vi "MainKinetics.vi"() -> ()   [LabVIEW 2017]
uses:
  <vilib>/Utility/miscctls.llb/LVRowAndColumnTypeDef.ctl
  <vilib>/Utility/sysdir.llb/System Directory Type.ctl
  <vilib>/Utility/config.llb/Read Key (String).vi
  <vilib>/Utility/config.llb/Write Key (String).vi
  <vilib>/Utility/cursorutil.llb/Set Cursor (Icon Pict).vi
  PCAN_Driver/ControlCAN.lvlib
  <vilib>/Utility/config.llb/NI_LVConfig.lvlib
panel:
  out "CurrentOut":string
  out "VISA Current":refnum<visa-resource-name>
  out "Offset":dbl
  out "Analogtest":bool=TRUE
  out "TestinExecution":string
  out "FullSpeed2 Current":dbl
  out "FullSpeed1 Current":dbl
  out "String":string
  out "ParamVersion":string
  out "DSP Board S/N":string
  out "POWER Board S/N":string caption="DRIVER Board S/N"
  in  "EventTimeout":i32=100
  out "SpeedLimit":dbl[](array[numeric])
  out "TestArray":string[](array[string])
  out "Motor Speed RPM Serial":dbl
  out "DAQmx Device Name":tag
  out "PN":string
  out "FileName":string
  out "VenableSpeed":u16
  out "TesterVersion":string
  out "ClosePanel":bool=TRUE
  out "UUT SN Report":string
  out "Automation":bool
  out "Test Failed":bool
  out "VisualInspectionResult":bool
  out "MotorTempResult":bool
  out "VenableDirectionResult":bool
  out "VenableResult":bool
  out "ComTestResult":bool=TRUE
  out "UUT SoftwareVer":string
  out "Next SN":i32
  in  "SetSN":bool
  out "Current SN":i32
  out "FullSpeed2 Speed":dbl
  out "FullSpeed2 Current":dbl
  out "FullSpeed1 Current":dbl
  out "FullSpeed1 Speed":dbl
  out "UUT":u8
  out "CAN Status":bool
  out "Array":u64[][](array[numeric]) format="%016x"
  out "Motor Phase Current RMS":dbl
  out "Ambient Temperature":dbl
  out "Speed error":bool
  out "Commutation err":bool
  out "Under voltage/Over voltage":bool
  out "Derated drive temp":bool
  out "Motor Over temperature":bool
  out "Motor Sensor temp Fauilre":bool
  out "Drive Over temperature":bool
  out "Drive Sensor temp Failure":bool
  out "Ambient Over temp":bool
  out "Ambient Sensor temp":bool
  out "DC Voltage":dbl
  out "DC Current":dbl
  out "Power transistor Heat sink Temp.":dbl
  out "Motor Stator Temp.":dbl
  out "Motor Speed RPM":dbl
  out "ECS State":u16
  out "UUT":string="EBAY"
  in  "Logger Path":path
  in  "Report":bool
  in  "Start":bool
  in  "ATR":string[][](table)=[["Test Communication", "-", "-", "-", "-", ""], ["Set S/N", "-", "-", "-", "-", ""], ["Set Board Number", "-", "-", "-", "-", ""], [" ", "", "", "", "", ""], ["Test Communication", "-", "-", "-", "-", ""], ["Get S/N", "-", "-", "-", "", ""], ["Get Board Number", "-", "-", "-", "", ""], ["Get FW", "-", "-", "-", "", ""], ["Enable Motor", "", "", "", "", ""], ["Small position command", "", "", "", "", ""], ["Measure delta", "", "", "", "", ""], ["Velocity command", "", "", "", "", ""]]
  in  "Settings":bool
  in  "Refresh Button":bool
  out "Serial Status":bool
  in  "VISA Kinetics":refnum<visa-resource-name>="COM6"
  in  "Serial Com":bool
  in  "Help Button":bool
  out "Pannel User Message":string
  in  "Stop Button":bool
  # "Kinetics"
  # "REDLER TECHNOLOGIES LTD"
  # "ver 1.2p"
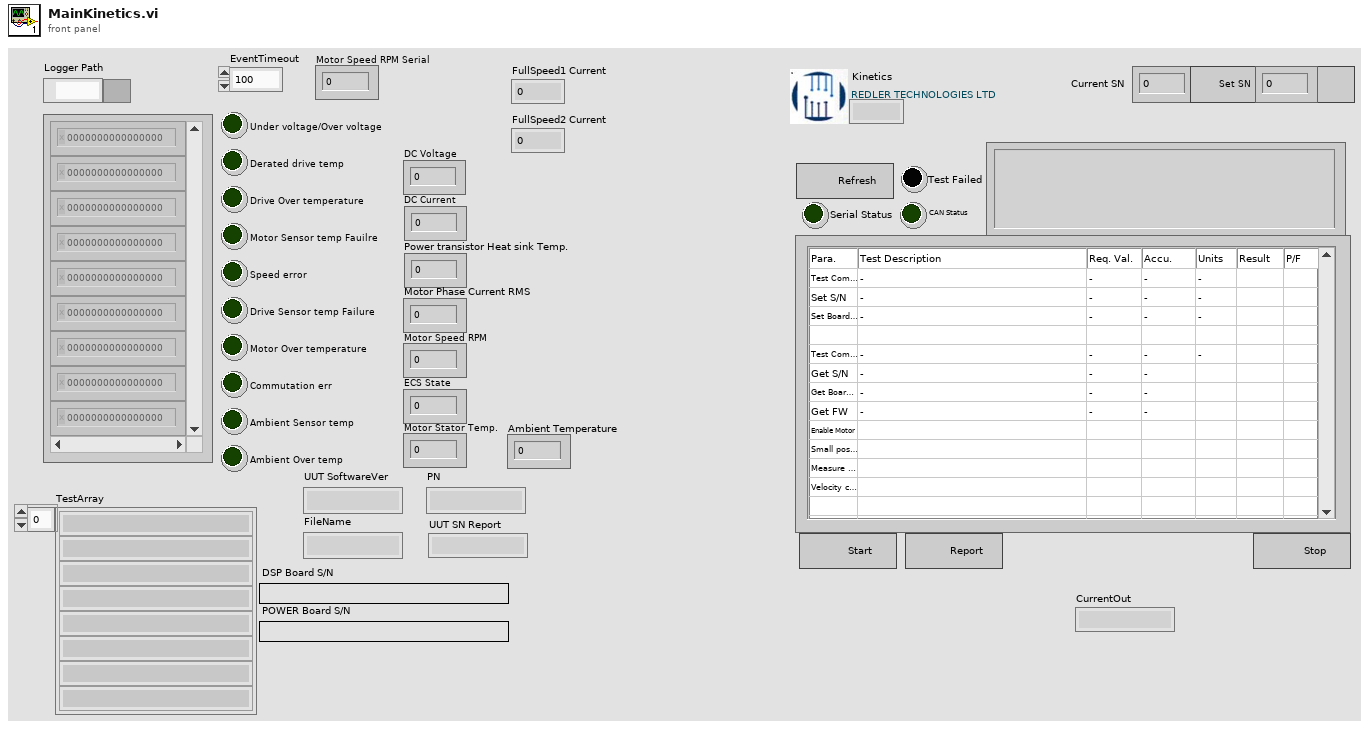
[diagram p1: front panel]
types:
  T1 = cluster{"VISA":refnum<visa-resource-name>, "TestArray":string[]}
  T2 = cluster{"ID":u32, "MSGTYPE":u8, "LEN":u8, "aDATA":u8[]}[]
  T3 = enum16{"Erase ATR Table", "Stop", "MainProgram", "Initialize"}
  T4 = typedef "NI_LVConfig.lvlib/Config Data RefNum.ctl" = refnum<k1>
  T5 = enum16{"Init", "0 ohm", "6 ohm", "13.2 ohm", "15 ohm", "25.9 ohm", "33 ohm", "Down", "Up", "Venable", "Firmware", "PowerSuply"}
  T6 = enum16{"Wait", "Exit", "VC=0", "ReadVC", "VC=1000"}
  T7 = enum16{"Stop", "Result", "FullSpeed2", "MD[1]=1", "FullSpeed1", "MD[1]=0"}
  T8 = enum16{"K15", "K16", "K17", "Venable", "Firmeware", "Fan", "Power", "120C", "110C", "100C", "90C", "80C", "70C", "60C", "50C", "40C", "30C", "25C", "20C", "10C", "0C"}
  T9 = enum8{"Term1", "Term2", "Current", "Fan", "TempCPU"}
  T10 = enum16{"Exit", "AI0/3", "AO0", "Wait", "Read", "Init"}
  T11 = enum16{"Exit", "Wait", "ReadCurrent", "ReadTemp", "Init"}
  T12 = enum16{"Init", "0 ohm", "6 ohm", "13.2 ohm", "15 ohm", "25.9 ohm", "33 ohm", "Down", "Up", "Venable", "Firmware", "PowerSuply"}[]
  T13 = enum8{"Enabled", "Disabled", "Disabled and Grayed Out"}
  T14 = typedef "LVRowAndColumnTypeDef.ctl" = cluster{"Row":i32, "Column":i32}
  T15 = enum32{"Invalid", "Standard", "Closed", "Hidden", "Minimized", "Maximized"}
  T16 = cluster{"ID":u32, "MSGTYPE":u8, "LEN":u8, "aDATA":u8[]}
  T17 = enum16{"open", "replace", "create", "open or create", "replace or create", "replace or create with confirmation"}
  T18 = typedef "ControlCAN.lvlib/DevType.ctl" = u32
  T19 = typedef "ControlCAN.lvlib/CAN Channel.ctl" = u32
  T20 = typedef "ControlCAN.lvlib/VCI_INIT_CONFIG.ctl" = cluster{"AccCode":u32, "AccMask":u32, "InitFlag":T21, "Fliter":T22, "Timing0":u8, "Timing1":u8, "Mode":T23}
  T21 = typedef "ControlCAN.lvlib/InitFlag.ctl" = u32
  T22 = typedef "ControlCAN.lvlib/Fliter.ctl" = u8
  T23 = typedef "ControlCAN.lvlib/Mode.ctl" = u8
  T24 = cluster{"DevType":T18, "DevIndex":u32, "CanIndex":T19, "VCI_INIT_CONFIG":T20}
  T25 = typedef "ControlCAN.lvlib/VCI_CAN_OBJ.ctl" = cluster{"ID":u32, "TimeStamp":u32, "TimeFlag":u8, "SendType":u8, "RemoteFlag":u8, "ExternFlag":u8, "DataLen":u8, "Data":u8[], "Reserved":u8[]}
  T26 = cluster{"Type":enum16{"接收", "发送"}, "Channel":T19, "Time":timestamp, "VCI_CAN_OBJ":T25}[]
  T27 = cluster{"Type":enum16{"接收", "发送"}, "Channel":T19, "Time":timestamp, "VCI_CAN_OBJ":T25}
  T28 = typedef "LVPoint32TypeDef.ctl" = cluster{"Horizontal":i32, "Vertical":i32}
  T29 = typedef "System Directory Type.ctl" = i32
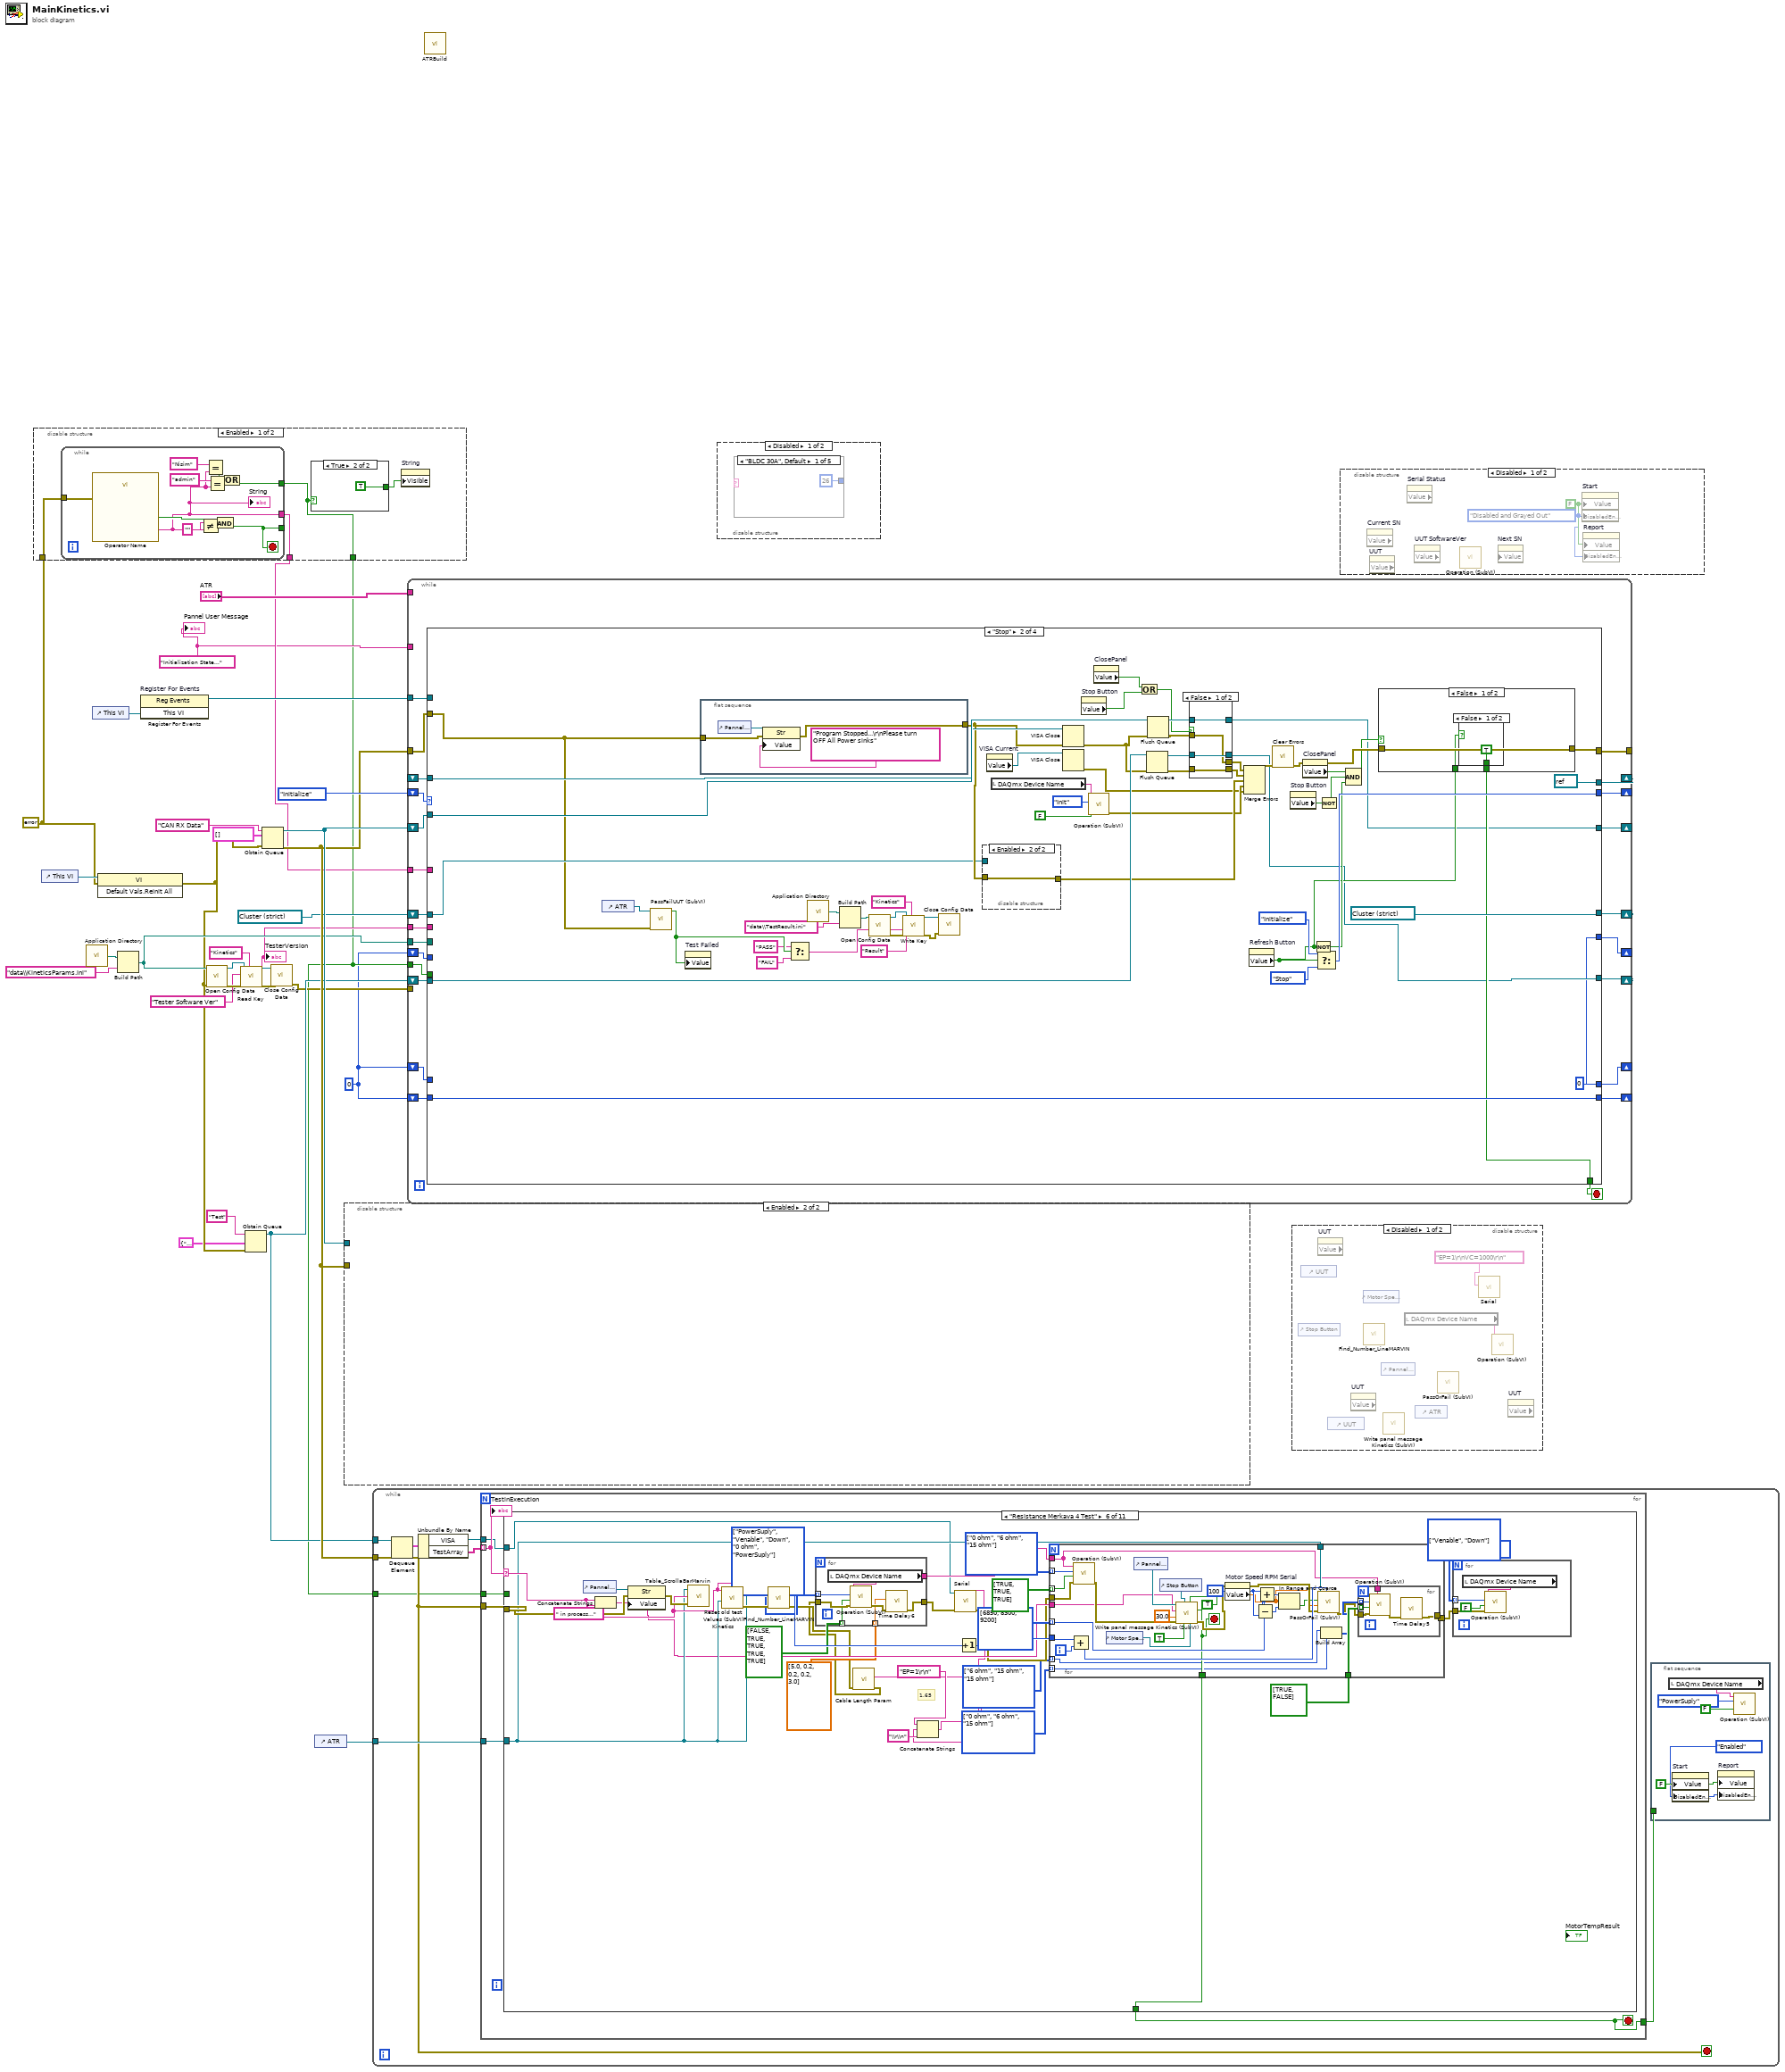
[diagram p0: block diagram]
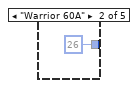
[diagram p2: hidden frame]
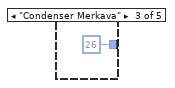
[diagram p3: hidden frame]
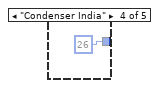
[diagram p4: hidden frame]
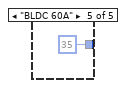
[diagram p5: hidden frame]
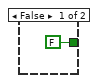
[diagram p7: hidden frame]
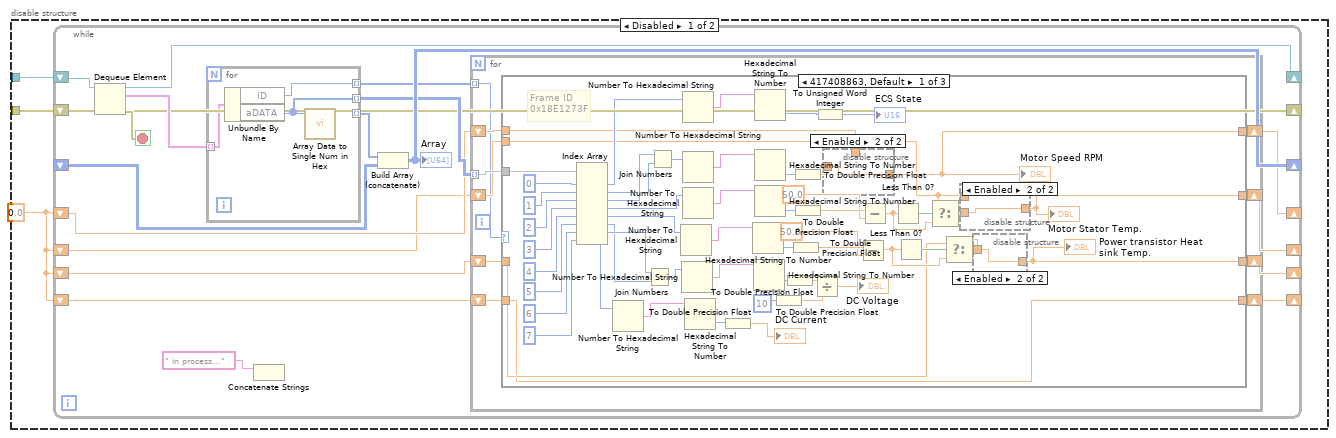
[diagram p9: hidden frame]
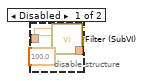
[diagram p10: hidden frame]
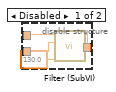
[diagram p11: hidden frame]
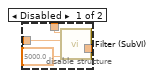
[diagram p12: hidden frame]
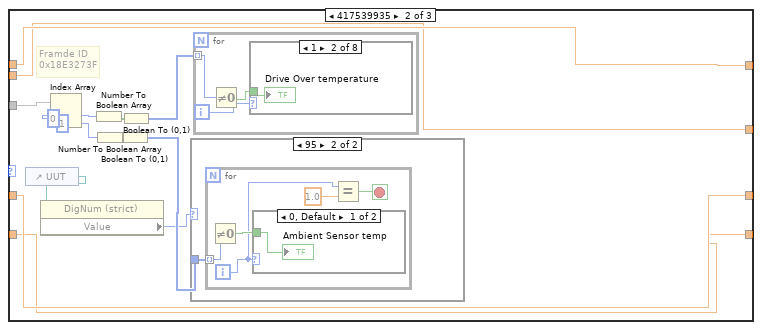
[diagram p13: hidden frame]
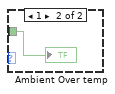
[diagram p15: hidden frame]
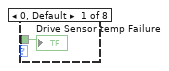
[diagram p16: hidden frame]
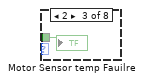
[diagram p17: hidden frame]
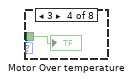
[diagram p18: hidden frame]
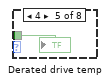
[diagram p19: hidden frame]
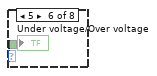
[diagram p20: hidden frame]
diagram:
  w17 = "Initialization State..."
  w2 = 0
  w5 = errorcluster {"status"=FALSE, "code"=0, "source"=""} ("error in (no error)")
  n1 = disable-structure shown="Enabled" {
    disable-tunnel: [w35 _] -> w18
    disable-tunnel: w5 -> [w33 _]
    disable-tunnel: [w32 _] -> w3
    frame Enabled {
      n2 = while {
        tunnel: [w45] -> _
        tunnel: [w38] -> w35
        tunnel: [w42] -> w32
        tunnel: w33 -> [w39]
        stop <- w45 stop-if-true
        n3 = call "Operator Name"("error in (no error)"=w39) -> ("Operator Name"=w38:string, "OK"=w46:bool)  [unwired: 16 in, 1 out]
        "String" <- w38
        n4 = Not Equal?(x=w38, y="") -> (x != y?=w47:bool)
        n5 = Equal?(x="Nisim", y=w38) -> (x = y?=w40:bool)
        n6 = Equal?(x="admin", y=w38) -> (x = y?=w43:bool)
        n7 = And(x=w46, y=w47) -> (x .and. y?=w45:bool)
        n8 = Or(x=w40, y=w43) -> (x .or. y?=w42:bool)
      }
      n9 = case shown="True" w32 {
        tunnel: [FALSE TRUE] -> w34
        frame False {
        }
        frame True {
        }
      }
      n10 = property on="String" class="Str"("Visible"=w34) -> ()  [unwired: 2 in, 2 out]
    }
    frame Disabled {
    }
  }
  n11 = control-ref of="This VI"() -> (w6:refnum<vi>)
  n12 = call <vilib>:"Application Directory.vi"() -> ("Application Directory"=w22:path)
  n13 = control-ref of="This VI"() -> (w20:refnum<vi>)
  n14 = invoke class="VI" method="Default Vals.Reinit All"(reference=w6, error in=w5) -> (error out=w4:errorcluster)  [unwired: 1 in, 2 out]
  n15 = Build Path(base path=w22, name or relative path="data\\KineticsParams.ini") -> (appended path=w9:path)
  n16 = register-events "Register For Events"(w20) -> (reference out=w19:refnum<event-registration>)  [unwired: 2 in, 1 out]
  n17 = call <vilib>:"Open Config Data.vi"("error in (no error)"=w4, "configuration file path"=w9) -> ("error out"=w15:errorcluster, "refnum"=w14:T4)  [unwired: 1 in, 7 out]
  n18 = call-poly <vilib>:"Read Key.vi"("section"="Kinetics", "error in (no error)"=w15, "key"="Tester Software Ver", "refnum"=w14) -> ("error out"=w12:errorcluster, "value"=w7:string, "refnum out"=w11:T4)  [unwired: 2 in, 3 out]
  "TesterVersion" <- w7
  n19 = Obtain Queue(name (unnamed)="Test", element data type=T1 {"VISA"="COM1", "TestArray"=[]}, error in (no error)=w4) -> (queue out=w25:refnum<queue>)  [unwired: 2 in, 2 out]
  n20 = Obtain Queue(name (unnamed)="CAN RX Data", element data type=T2 [], error in (no error)=w4) -> (queue out=w28:refnum<queue>, error out=w26:errorcluster)  [unwired: 2 in, 1 out]
  n21 = call <vilib>:"Close Config Data.vi"("error in (no error)"=w12, "refnum"=w11) -> ("error out"=w10:errorcluster)  [unwired: 8 in, 1 out]
  n22 = control-ref of="ATR"() -> (w16:refnum<vi>)
  n23 = disable-structure shown="Enabled" {
    disable-tunnel: w28 -> [w51 _]
    disable-tunnel: w26 -> [w50 _]
    frame Disabled {
      w49 = 0.0
      n24 = while {
        shift-right: [w68] -> _
        shift-left: w51 -> [w70]
        shift-right: [w66] -> _
        shift-left: _ -> [w67]
        shift-right: [w62] -> _
        shift-left: w50 -> [w62]
        shift-right: [w60] -> _
        shift-left: w49 -> [w61]
        shift-right: [w59] -> _
        shift-left: w49 -> [w58]
        shift-right: [w57] -> _
        shift-left: w49 -> [w56]
        shift-right: [w55] -> _
        shift-left: w49 -> [w54]
        stop <- w69 stop-if-true
        n25 = Dequeue Element(queue=w70, error in (no error)=w62) -> (queue out=w68:refnum<queue>, element=w63:T2, error out=w69:errorcluster)  [unwired: 1 in, 1 out]
        n26 = for {
          tunnel: [w216] -> w65 mode=indexing
          tunnel: w63 -> [w215] mode=indexing
          tunnel: [w214] -> w64 mode=indexing
          tunnel: [w213] -> w53 mode=indexing
          n27 = Unbundle By Name(w215) -> ("ID"=w213:u32, "aDATA"=w214:u8[])
          n28 = call "Array Data to Single Num in Hex.vi"("aDATA"=w214) -> ("Numeric"=w216:u64)  [unwired: 10 in]
        }
        n29 = Concatenate Strings(" in process..." ("Strin")) -> ()  [unwired: 1 in, 1 out]
        n30 = Build Array (concatenate)(w65, w67) -> (w66:u64[][])
        "Array" <- w66
        n31 = for {
          tunnel: w64 -> [w80] mode=indexing
          shift-right: [w78] -> w60
          shift-left: w61 -> [w79]
          shift-right: [w77] -> w59
          shift-left: w58 -> [w76]
          shift-right: [w75] -> w57
          shift-left: w56 -> [w74]
          shift-right: [w73] -> w55
          shift-left: w54 -> [w72]
          tunnel: w53 -> [w71] mode=indexing
          n32 = case shown="417408863, Default" w71 {
            tunnel: w80 -> [w117 w165 w203]
            tunnel: w79 -> [w91 w154 w192]
            tunnel: [w90 w154 w192] -> w78
            tunnel: [w87 w153 w191] -> w77
            tunnel: w76 -> [w86 w153 w191]
            tunnel: [w83 w152 w190] -> w75
            tunnel: w74 -> [w82 w152 w190]
            tunnel: [w81 w151 w186] -> w73
            tunnel: w72 -> [w81 w151 w185]
            frame 417408863, Default {
              # "Frame ID\n0x18E1273F"
              n33 = Index Array(array=w117, index #1=0 ("index"), index #2=1 ("index"), index #3=2 ("index"), index #4=3 ("index"), index #5=4 ("index"), index #6=5 ("index"), index #7=6 ("index"), index #8=7 ("index")) -> (element #1=w101:u8, element #2=w103:u8, element #3=w104:u8, element #4=w108:u8, element #5=w111:u8, element #6=w115:u8, element #7=w116:u8, element #8=w114:u8)
              n34 = Number To Hexadecimal String(2:w114) -> (0:w128:string)  [unwired: 1 in]
              n35 = Join Numbers(hi=w116, lo=w115) -> ((hi.lo)=w135:u16)
              n36 = Join Numbers(hi=w104, lo=w103) -> ((hi.lo)=w105:u16)
              n37 = Number To Hexadecimal String(2:w111) -> (0:w112:string)  [unwired: 1 in]
              n38 = Number To Hexadecimal String(2:w135) -> (0:w134:string)  [unwired: 1 in]
              n39 = Number To Hexadecimal String(2:w101) -> (0:w102:string)  [unwired: 1 in]
              n40 = Number To Hexadecimal String(2:w105) -> (0:w106:string)  [unwired: 1 in]
              n41 = Number To Hexadecimal String(2:w108) -> (0:w109:string)  [unwired: 1 in]
              n42 = Hexadecimal String To Number(string=w128) -> (number=w127:u32)  [unwired: 2 in, 1 out]
              n43 = To Double Precision Float(number=w127) -> (double precision float=→"DC Current":dbl)
              n44 = Hexadecimal String To Number(string=w112) -> (number=w113:u32)  [unwired: 2 in, 1 out]
              n45 = Hexadecimal String To Number(string=w134) -> (number=w133:u32)  [unwired: 2 in, 1 out]
              n46 = Hexadecimal String To Number(string=w102) -> (number=w99:u32)  [unwired: 2 in, 1 out]
              n47 = Hexadecimal String To Number(string=w106) -> (number=w107:u32)  [unwired: 2 in, 1 out]
              n48 = Hexadecimal String To Number(string=w109) -> (number=w110:u32)  [unwired: 2 in, 1 out]
              n49 = To Double Precision Float(number=u32 10 ("y")) -> (double precision float=w131:dbl)
              n50 = To Double Precision Float(number=w133) -> (double precision float=w130:dbl)
              n51 = To Double Precision Float(number=w113) -> (double precision float=w96:dbl)
              n52 = To Double Precision Float(number=w107) -> (double precision float=w92:dbl)
              n53 = To Double Precision Float(number=w110) -> (double precision float=w98:dbl)
              n54 = Divide(x=w130, y=w131) -> (x/y=→"DC Voltage":dbl)
              n55 = To Unsigned Word Integer(number=w99) -> (unsigned 16bit integer=→"ECS State":u16)
              n56 = disable-structure shown="Enabled" {
                disable-tunnel: w92 -> [w149 w150]
                disable-tunnel: w91 -> [w148 _]
                disable-tunnel: [w146 w150] -> w90
                frame Disabled {
                  n57 = call "Filter (SubVI).vi"("Delta"=5000.0, "NewVal"=w149, "OldVal"=w148) -> ("Val"=w146:dbl)  [unwired: 8 in]
                }
                frame Enabled {
                }
              }
              "Motor Speed RPM" <- w90
              n58 = Subtract(x=w96, y=50.0 ("x")) -> (x-y=w85:dbl)
              n59 = Subtract(x=w98, y=50.0 ("x")) -> (x-y=w88:dbl)
              n60 = Less Than 0?(x=w88) -> (x < 0?=w94:bool)
              n61 = Less Than 0?(x=w85) -> (x < 0?=w93:bool)
              n62 = Select(t=w86, s=w94, f=w88) -> (s? t:f=w89:dbl)
              n63 = Select(t=w82, s=w93, f=w85) -> (s? t:f=w84:dbl)
              n64 = disable-structure shown="Enabled" {
                disable-tunnel: w89 -> [w144 w145]
                disable-tunnel: [w143 w145] -> w87
                disable-tunnel: w86 -> [w142 _]
                frame Disabled {
                  n65 = call "Filter (SubVI).vi"("Delta"=130.0, "NewVal"=w144, "OldVal"=w142) -> ("Val"=w143:dbl)  [unwired: 8 in]
                }
                frame Enabled {
                }
              }
              "Motor Stator Temp." <- w87
              n66 = disable-structure shown="Enabled" {
                disable-tunnel: w84 -> [w139 w140]
                disable-tunnel: [w137 w140] -> w83
                disable-tunnel: w82 -> [w136 _]
                frame Disabled {
                  n67 = call "Filter (SubVI).vi"("Delta"=100.0, "NewVal"=w139, "OldVal"=w136) -> ("Val"=w137:dbl)  [unwired: 8 in]
                }
                frame Enabled {
                }
              }
              "Power transistor Heat sink Temp." <- w83
            }
            frame 417539935 {
              # "Framde ID\n0x18E3273F"
              n68 = control-ref of="UUT"() -> (w155:refnum<vi>)
              n69 = property on="Property Node" class="DigNum (strict)"(reference=w155) -> ("Value"=w156:u8)  [unwired: 1 in, 2 out]
              n70 = Index Array(array=w165, index #1=0 ("index"), index #2=1 ("index")) -> (element #1=w163:u8, element #2=w158:u8)
              n71 = Number To Boolean Array(number=w163) -> (Boolean array=w162:bool[])
              n72 = Number To Boolean Array(number=w158) -> (Boolean array=w160:bool[])
              n73 = Boolean To (0,1)(Boolean=w160) -> (0, 1=w157:i16[])
              n74 = Boolean To (0,1)(Boolean=w162) -> (0, 1=w161:i16[])
              n75 = case shown="95" w156 {
                tunnel: w157 -> [_ w166]
                frame 0, Default {
                }
                frame 95 {
                  n76 = for {
                    tunnel: w166 -> [w171] mode=indexing
                    i -> [w167]
                    stop <- w169 stop-if-true
                    n77 = Not Equal To 0?(x=w171) -> (x != 0?=w170:bool)
                    n78 = case shown="0, Default" w167 {
                      tunnel: w170 -> [w172 w173]
                      frame 0, Default {
                        "Ambient Sensor temp" <- w172
                      }
                      frame 1 {
                        "Ambient Over temp" <- w173
                      }
                    }
                    n79 = Equal?(x=w167, y=1.0) -> (x = y?=w169:bool)
                  }
                }
              }
              n80 = for {
                tunnel: w161 -> [w175] mode=indexing
                i -> [w176]
                n81 = Not Equal To 0?(x=w175) -> (x != 0?=w174:bool)
                n82 = case shown="1" w176 {
                  tunnel: w174 -> [w177 w178 w179 w180 w181 w182 w183 w184]
                  frame 0, Default {
                    "Drive Sensor temp Failure" <- w177
                  }
                  frame 1 {
                    "Drive Over temperature" <- w178
                  }
                  frame 2 {
                    "Motor Sensor temp Fauilre" <- w179
                  }
                  frame 3 {
                    "Motor Over temperature" <- w180
                  }
                  frame 4 {
                    "Derated drive temp" <- w181
                  }
                  frame 5 {
                    "Under voltage/Over voltage" <- w182
                  }
                  frame 6 {
                    "Commutation err" <- w183
                  }
                  frame 7 {
                    "Speed error" <- w184
                  }
                }
              }
            }
            frame 417474399 {
              # "Frame ID\n0x18E2273F"
              n83 = Index Array(array=w203, index #1=0 ("index"), index #2=1 ("index")) -> (element #1=w200:u8, element #2=w197:u8)
              n84 = disable-structure shown="Enabled" {
                disable-tunnel: [w211 w212] -> w201
                disable-tunnel: w200 -> [w210 w212]
                frame Disabled {
                  n85 = Number To Hexadecimal String(2:w210) -> (0:w209:string)  [unwired: 1 in]
                  n86 = Hexadecimal String To Number(string=w209) -> (number=w211:u32)  [unwired: 2 in, 1 out]
                }
                frame Enabled {
                }
              }
              n87 = Number To Hexadecimal String(2:w197) -> (0:w195:string)  [unwired: 1 in]
              n88 = Hexadecimal String To Number(string=w195) -> (number=w196:u32)  [unwired: 2 in, 1 out]
              n89 = To Double Precision Float(number=w196) -> (double precision float=w194:dbl)
              n90 = To Double Precision Float(number=w201) -> (double precision float=→"Motor Phase Current RMS":dbl)
              n91 = Subtract(x=w194, y=50.0) -> (x-y=w188:dbl)
              n92 = Less Than 0?(x=w188) -> (x < 0?=w189:bool)
              n93 = Select(t=w185, s=w189, f=w188) -> (s? t:f=w187:dbl)
              n94 = disable-structure shown="Disabled" {
                disable-tunnel: w187 -> [w207 w208]
                disable-tunnel: [w205 w208] -> w186
                disable-tunnel: w185 -> [w204 _]
                frame Disabled {
                  n95 = call "Filter (SubVI).vi"("Delta"=65.0, "NewVal"=w207, "OldVal"=w204) -> ("Val"=w205:dbl)  [unwired: 8 in]
                }
                frame Enabled {
                }
              }
              "Ambient Temperature" <- w186
            }
          }
        }
      }
    }
    frame Enabled {
    }
  }
  n96 = while {
    tunnel: w16 -> [w225]
    tunnel: w26 -> [w223]
    tunnel: w25 -> [w224]
    tunnel: w3 -> [w218]
    stop <- w220 stop-if-true
    n97 = Dequeue Element(queue=w224, error in (no error)=w223) -> (element=w222:T1, error out=w220:errorcluster)  [unwired: 1 in, 2 out]
    n98 = Unbundle By Name(w222) -> ("VISA"=w221:refnum<visa-resource-name>, "TestArray"=w217:string[])
    n99 = for {
      tunnel: w217 -> [w235] mode=indexing
      tunnel: w221 -> [w233]
      tunnel: w225 -> [w232]
      tunnel: w220 -> [w236]
      tunnel: [w231] -> w219
      tunnel: w218 -> [w234]
      stop <- w231 stop-if-true
      n100 = case shown="\"Resistance Merkava 4 Test\"" w235 {
        selector: w235 -> [_ w254 w659 w1120 w1247 w1395 w1475 w1554 w1640 w1801 w1919]
        tunnel: w232 -> [_ w247 _ _ w1240 w1389 w1469 w1548 w1641 w1809 w1917]
        tunnel: w236 -> [_ w257 _ _ w1255 w1394 w1474 w1553 w1642 w1816 w1921]
        tunnel: w234 -> [_ _ _ _ _ _ _ _ _ _ _]
        tunnel: w233 -> [_ w250 w658 w1119 w1243 w1383 w1466 w1539 w1618 w1802 w1918]
        tunnel: [TRUE ("Stopped") w242 w657 w1109 w1236 w1378 w1459 w1541 w1632 w1800 FALSE ("Stopped")] -> w231
        frame "", Default {
        }
        frame "Comm. & Motor Test" {
          n101 = control-ref of="Pannel User Message"() -> (w258:refnum<vi>)
          n102 = Concatenate Strings(w254, " in process..." ("string")) -> (w249:string)
          n103 = property class="Str"(reference=w258, error in=w257, "Value"=w249) -> (error out=w256:errorcluster)  [unwired: 1 out]
          n104 = call "Table_ScrollaBarMarvin.vi"("error in"=w256, "Line to focus"=w254, "reference in"=w247) -> ("error out"=w253:errorcluster)  [unwired: 2 out]
          n105 = property on="UUT" class="Str"() -> ("Value"=w246:string)  [unwired: 2 in, 2 out]
          n106 = call "Find_Number_LineMARVIN.vi"("Test Paragraph"=w254, "error in"=w253, "TableIn"=w247) -> ("error out"=w259:errorcluster, "Line number"=w238:i32)  [unwired: 2 in, 2 out]
          n107 = Concatenate Strings("- Set the FIREWERE switch to OFF position." ("Screen Line"), "- Set the VENABLE switch to ON position." ("Screen Line")) -> (w243:string)
          n108 = call <vilib>:"Clear Errors.vi"("error in (no error)"=w259) -> ("error out"=w252:errorcluster)  [unwired: 5 in, 1 out]
          n109 = Add(x=3, y=w238) -> (x+y=w248:i32)
          n110 = call "Reset old test Values (SubVI) Kinetics.vi"("error in"=w252, "Atr in"=w247, "Test Paragraph"=w254) -> ("error out"=w241:errorcluster)  [unwired: 6 in, 2 out]
          n111 = case shown="\"Condenser India\", \"Condenser Merkava\"" w246 {
            tunnel: w243 -> [_ w656]
            tunnel: w241 -> [w654 w655]
            tunnel: [w654 w655] -> w240
            frame "False", Default {
            }
            frame "Condenser India", "Condenser Merkava" {
              n112 = One Button Dialog(message=w656) -> ()  [unwired: 1 in, 1 out]
            }
          }
          n113 = for {
            N: 2 -> [_]
            tunnel: w250 -> [w267]
            tunnel: w249 -> [w266]
            tunnel: w248 -> [w265]
            tunnel: w247 -> [w264]
            tunnel: [w263] -> w242
            tunnel: w240 -> [w262]
            tunnel: w238 -> [w260]
            i -> [w261]
            n114 = case shown="1" w261 {
              tunnel: w267 -> [w285 w376]
              tunnel: w266 -> [w284 w375]
              tunnel: w265 -> [w282 _]
              tunnel: w264 -> [w275 w373]
              tunnel: [w280 w377] -> w263
              tunnel: w262 -> [w271 _]
              tunnel: w260 -> [w277 _]
              frame 0, Default {
                n115 = Increment(x=w277) -> (x+1=w270:i32)
                n116 = property on="Serial Status" class="Bool (strict)"() -> ("Value"=w279:bool)  [unwired: 2 in, 2 out]
                n117 = property on="UUT SoftwareVer" class="Str"() -> ("Value"=w268:string)  [unwired: 2 in, 2 out]
                n118 = call "PassOrFail (SubVI).vi"("String Res"=w268, "index (row)"=w270, "error in (no error)"=w271, "Data in"=-3.0, "Pass?Fail"=w279, "Table in"=w275) -> ("error out"=w273:errorcluster)  [unwired: 5 in]
                n119 = Increment(x=w270) -> (x+1=w269:i32)
                n120 = property on="CAN Status" class="Bool (strict)"() -> ("Value"=w274:bool)  [unwired: 2 in, 2 out]
                n121 = call "PassOrFail (SubVI).vi"("String Res"=w268, "index (row)"=w269, "error in (no error)"=w273, "Data in"=-3.0, "Pass?Fail"=w274, "Table in"=w275) -> ("error out"=w272:errorcluster)  [unwired: 5 in]
                n122 = while {
                  shift-right: [w296] -> _
                  shift-left: T6."VC=1000" -> [w299]
                  tunnel: w272 -> [w298]
                  tunnel: w285 -> [w297]
                  tunnel: w284 -> [w295]
                  shift-right: [w292] -> w281
                  shift-left: bool[] [FALSE, FALSE] -> [w293]
                  tunnel: w282 -> [w291]
                  tunnel: w275 -> [w290]
                  tunnel: [w288] -> w280
                  i -> [w294]
                  stop <- w289 stop-if-true
                  n123 = case shown="\"VC=0\"" w299 {
                    tunnel: w298 -> [_ w322 _ w353 _]
                    tunnel: w297 -> [w302 w320 w329 w357 _]
                    tunnel: [T6."Exit" T6."Wait" w326 T6."Wait" T6."ReadVC"] -> w296
                    tunnel: w295 -> [_ _ _ _ w365]
                    tunnel: [TRUE FALSE FALSE FALSE FALSE] -> w289
                    tunnel: w294 -> [_ _ w327 _ w360]
                    tunnel: w293 -> [w301 w317 w325 w355 w362]
                    tunnel: [w301 w317 w324 w355 w362] -> w292
                    tunnel: w291 -> [w310 _ _ _ _]
                    tunnel: w290 -> [w312 _ _ _ _]
                    tunnel: [_ _ _ _ w359] -> w288
                    frame "Exit", Default {
                      n124 = And Array Elements(Boolean array=w301) -> (logical AND=w305:bool)
                      n125 = local read "DAQmx Device Name"() -> (w309:tag)
                      n126 = Select(t="OK", s=w305, f="Failed") -> (s? t:f=w311:string)
                      n127 = call "PassOrFail (SubVI).vi"("String Res"=w311, "index (row)"=w310, "Data in"=-3.0, "Pass?Fail"=w305, "Table in"=w312) -> ("error out"=w300:errorcluster)  [unwired: 6 in]
                      n128 = call "Serial.vi"("error in (no error)"=w300, "write buffer"="EP=1\r\nVC=0\r\n", "VISA resource name"=w302) -> ("error out"=w303:errorcluster)  [unwired: 7 in, 1 out]
                      n129 = call "Operation (SubVI).vi"("error in (no error)"=w303, "On/Off"=FALSE, "Operation"=T5."Venable", "DAQmx Device Name"=w309) -> ()  [unwired: 7 in, 1 out]
                    }
                    frame "VC=0" {
                      n130 = call "Serial.vi"("error in (no error)"=w322, "write buffer"="EP=1\r\nVC=0\r\n", "VISA resource name"=w320) -> ()  [unwired: 7 in, 2 out]
                    }
                    frame "ReadVC" {
                      n131 = call "Serial.vi"("write buffer"="VC\r\n", "VISA resource name"=w329) -> ("read buffer"=w328:string)  [unwired: 8 in, 1 out]
                      n132 = case shown="5, Default" w327 {
                        tunnel: w328 -> [w338 w344]
                        tunnel: [T6."VC=0" T6."Exit"] -> w326
                        tunnel: w325 -> [w333 w343]
                        tunnel: [w331 w340] -> w324
                        frame 2 {
                          n133 = Decimal String To Number(string=w338) -> (number=w337:i32)  [unwired: 2 in, 1 out]
                          n134 = In Range and Coerce(upper limit=1100, x=w337, lower limit=900) -> (In Range?=w332:bool)  [unwired: 1 out]
                          n135 = Replace Array Subset(array=w333, new element=w332, index=0) -> (w331:bool[])
                        }
                        frame 5, Default {
                          n136 = Decimal String To Number(string=w344) -> (number=w347:i32)  [unwired: 2 in, 1 out]
                          n137 = In Range and Coerce(upper limit=100, x=w347, lower limit=0) -> (In Range?=w341:bool)  [unwired: 1 out]
                          n138 = Replace Array Subset(array=w343, new element=w341, index=1) -> (w340:bool[])
                        }
                      }
                    }
                    frame "VC=1000" {
                      n139 = local read "DAQmx Device Name"() -> (w354:tag)
                      n140 = call "Operation (SubVI).vi"("error in (no error)"=w353, "On/Off"=TRUE, "Operation"=T5."Venable", "DAQmx Device Name"=w354) -> ("error out"=w352:errorcluster)  [unwired: 7 in]
                      n141 = call "Serial.vi"("error in (no error)"=w352, "write buffer"="EP=1\r\nVC=1000\r\n", "VISA resource name"=w357) -> ()  [unwired: 7 in, 2 out]
                    }
                    frame "Wait" {
                      n142 = case shown="4" w360 {
                        tunnel: [25.0 ("Time to wait") 15.0 ("Time to wait")] -> w366
                        frame 4 {
                        }
                        frame 1, Default {
                        }
                      }
                      n143 = control-ref of="Motor Speed RPM Serial"() -> (w370:refnum<vi>)
                      n144 = control-ref of="Pannel User Message"() -> (w369:refnum<vi>)
                      n145 = control-ref of="Stop Button"() -> (w364:refnum<vi>)
                      n146 = call "Write panel message Kinetics (SubVI).vi"(4:"rpm"=w370, 5:"rpm"=TRUE ("rpm"), "PrintTime"=TRUE, "Stop"=w364, "Time to wait"=w366, "Strin"=w365, "String in"=w369) -> ("Stopped"=w359:bool)  [unwired: 3 in, 1 out]
                    }
                  }
                }
                n147 = And Array Elements(Boolean array=w281) -> (logical AND=→"ComTestResult":bool)
              }
              frame 1 {
                n148 = case shown="False" FALSE {
                  tunnel: [_ w399] -> w377
                  tunnel: w376 -> [w378 w398]
                  tunnel: w375 -> [_ w396]
                  tunnel: w373 -> [w384 _]
                  frame False {
                    n149 = Two Button Dialog(message="Is the motor run in he right direction?", 1:"No" ("F button name (\"Cancel\")"), 2:"Yes" ("T button name (\"OK\")")) -> (T button?=w380:bool)
                    n150 = call "Find_Number_LineMARVIN.vi"("Test Paragraph"="Motor Direction", "TableIn"=w384) -> ("Line number"=w395:i32)  [unwired: 3 in, 3 out]
                    n151 = Select(t="OK", s=w380, f="Failed") -> (s? t:f=w394:string)
                    n152 = call "PassOrFail (SubVI).vi"("String Res"=w394, "index (row)"=w395, "Data in"=-3.0, "Pass?Fail"=w380, "Table in"=w384) -> ("error out"=w392:errorcluster)  [unwired: 6 in]
                    n153 = call "Serial.vi"("error in (no error)"=w392, "write buffer"="EP=1\r\nVC=0\r\n", "VISA resource name"=w378) -> ("error out"=w393:errorcluster)  [unwired: 7 in, 1 out]
                    n154 = local read "DAQmx Device Name"() -> (w379:tag)
                    n155 = call "Operation (SubVI).vi"("error in (no error)"=w393, "On/Off"=FALSE, "Operation"=T5."Venable", "DAQmx Device Name"=w379) -> ()  [unwired: 7 in, 1 out]
                  }
                  frame True {
                    n156 = property on="UUT" class="Str"() -> ("Value"=w401:string)  [unwired: 2 in, 2 out]
                    n157 = case shown="\"BLDC 60A\"" w401 {
                      tunnel: [26 26 26 26 47] -> w402
                      tunnel: [_ _ _ _ 56] -> w403
                      tunnel: [_ _ _ _ "10800"] -> w397
                      frame "BLDC 30A", Default {
                      }
                      frame "Warrior 60A" {
                      }
                      frame "Condenser Merkava" {
                      }
                      frame "Condenser India" {
                      }
                      frame "BLDC 60A" {
                      }
                    }
                    n158 = local read "DAQmx Device Name"() -> (w407:tag)
                    n159 = control-ref of="Stop Button"() -> (w404:refnum<vi>)
                    n160 = control-ref of="ATR"() -> (w408:refnum<vi>)
                    n161 = control-ref of="Pannel User Message"() -> (w405:refnum<vi>)
                    n162 = control-ref of="Motor Speed RPM Serial"() -> (w406:refnum<vi>)
                    n163 = while {
                      shift-right: [w421] -> _
                      shift-left: T7."MD[1]=0" -> [w422]
                      tunnel: w404 -> [w420]
                      tunnel: w405 -> [w419]
                      tunnel: w406 -> [w418]
                      tunnel: w407 -> [w417]
                      tunnel: w402 -> [w416]
                      tunnel: w403 -> [w415]
                      tunnel: w408 -> [w414]
                      tunnel: [w409] -> w399
                      tunnel: w398 -> [w412]
                      tunnel: w397 -> [w411]
                      tunnel: w396 -> [w410]
                      stop <- w413 stop-if-true
                      n164 = case shown="\"MD[1]=1\"" w422 {
                        tunnel: [T7."Stop" T7."Stop" w472 w546 w571 w646] -> w421
                        tunnel: [TRUE w433 FALSE FALSE FALSE FALSE] -> w413
                        tunnel: w420 -> [_ _ w457 w523 w555 w623]
                        tunnel: w419 -> [_ _ w458 w524 w556 w624]
                        tunnel: w418 -> [_ _ w459 w518 w558 w618]
                        tunnel: w417 -> [_ w428 w462 w510 w561 w610]
                        tunnel: w416 -> [_ _ _ _ w557 _]
                        tunnel: w415 -> [_ _ w456 _ _ _]
                        tunnel: w414 -> [_ w435 _ _ _ _]
                        tunnel: w412 -> [_ w427 w452 _ w553 w615]
                        tunnel: w411 -> [_ _ w451 _ w550 _]
                        tunnel: w410 -> [_ _ w449 w515 w548 w614]
                        tunnel: [_ _ w448 w506 w547 w605] -> w409
                        frame "Stop", Default {
                        }
                        frame "Result" {
                          n165 = property on="FullSpeed2 Current" class="DigNum (strict)"() -> ("Value"=w440:dbl)  [unwired: 2 in, 2 out]
                          n166 = property on="FullSpeed1 Current" class="DigNum (strict)"() -> ("Value"=w439:dbl)  [unwired: 2 in, 2 out]
                          n167 = Subtract(x=w440, y=w439) -> (x-y=w447:dbl)
                          n168 = Absolute Value(x=w447) -> (abs(x)=w442:dbl)
                          n169 = Greater Or Equal?(x=w442, y=u32 5) -> (x >= y?=w434:bool)
                          n170 = call "Find_Number_LineMARVIN.vi"("Test Paragraph"="Motor Direction", "TableIn"=w435) -> ("Line number"=w444:i32)  [unwired: 3 in, 3 out]
                          n171 = Select(t="OK", s=w434, f="Failed") -> (s? t:f=w436:string)
                          n172 = call "PassOrFail (SubVI).vi"("String Res"=w436, "index (row)"=w444, "Data in"=-3.0, "Pass?Fail"=w434, "Table in"=w435) -> ("error out"=w426:errorcluster)  [unwired: 6 in]
                          n173 = call "Serial.vi"("error in (no error)"=w426, "write buffer"="EP=1\r\nVC=0\r\n", "VISA resource name"=w427) -> ("error out"=w432:errorcluster)  [unwired: 7 in, 1 out]
                          n174 = Not(x=TRUE) -> (.not. x?=w433:bool)
                          n175 = call "Operation (SubVI).vi"("error in (no error)"=w432, "On/Off"=FALSE, "Operation"=T5."Venable", "DAQmx Device Name"=w428) -> ()  [unwired: 7 in, 1 out]
                        }
                        frame "FullSpeed2" {
                          n176 = Search and Replace String(input string="EP=1\r\nVC=0\r\n" ("write buffer"), search string="0", replace string=w451) -> (result string=w455:string)  [unwired: 5 in, 3 out]
                          n177 = call "Serial.vi"("write buffer"=w455, "VISA resource name"=w452) -> ("error out"=w450:errorcluster)  [unwired: 8 in, 1 out]
                          n178 = Concatenate Strings(w449, "\nFull speed operation " ("string")) -> (w466:string)
                          n179 = call "Write panel message Kinetics (SubVI).vi"(4:"rpm"=w459, 5:"rpm"=TRUE ("rpm"), "PrintTime"=FALSE, "Stop"=w457, "error in (no error)"=w450, "Time to wait"=0.2, "Strin"=w466, "String in"=w458) -> ("error out"=w469:errorcluster, "Stopped"=w461:bool)  [unwired: 2 in]
                          n180 = flat-sequence {
                            tunnel: w469 -> [w476]
                            tunnel: [w476] -> w468
                            tunnel: [w475] -> w467
                            frame #0 {
                              n181 = call <vilib>:"High Resolution Relative Seconds.vi"() -> ("relative seconds"=w475:dbl)
                            }
                          }
                          n182 = while {
                            tunnel: w468 -> [w488]
                            tunnel: [w498] -> _
                            tunnel: w456 -> [w504]
                            tunnel: w467 -> [w502]
                            tunnel: w466 -> [w496]
                            tunnel: w459 -> [w482]
                            tunnel: w462 -> [w490]
                            tunnel: w461 -> [w489]
                            tunnel: [w477] -> w460
                            tunnel: w458 -> [w487]
                            tunnel: w457 -> [w486]
                            tunnel: [w477] -> w448
                            stop <- w505 stop-if-true
                            n183 = call <vilib>:"High Resolution Relative Seconds.vi"() -> ("relative seconds"=w503:dbl)
                            n184 = property class="DigNum (strict)"(reference=w482) -> ("Value"=w481:dbl)  [unwired: 1 in, 2 out]
                            n185 = Subtract(x=w503, y=w502) -> (x-y=w501:dbl)
                            n186 = call "Aquire AI2"("error in"=w488, "device name"=w490) -> ("data"=w493:dynamicdata, "error out"=w492:errorcluster)  [unwired: 15 in, 1 out]
                            n187 = Greater Or Equal?(x=w501, y=120.0) -> (x >= y?=w499:bool)
                            n188 = To Double Precision Float(number=w493) -> (double precision float=w491:dbl)
                            "FullSpeed2 Current" <- w491
                            n189 = Multiply(x=w491, y=25.0) -> (x*y=w485:dbl)
                            n190 = Greater Or Equal?(x=w485, y=w504) -> (x >= y?=w483:bool)
                            n191 = Greater Or Equal?(x=w481, y=10000.0) -> (x >= y?=w478:bool)
                            n192 = And(x=w483, y=w478) -> (x .and. y?=w479:bool)
                            n193 = call "Write panel message Kinetics (SubVI).vi"(4:"rpm"=w482, 5:"rpm"=TRUE ("rpm"), "PrintTime"=FALSE, "Stop"=w486, "error in (no error)"=w492, "Time to wait"=0.2, "Strin"=w496, "String in"=w487) -> ("error out"=w498:errorcluster, "Stopped"=w477:bool)  [unwired: 2 in]
                            n194 = Compound Arithmetic op=OR(w477, w489, w499, w479) -> (w505:bool)
                          }
                          n195 = Select(t=T7."Stop", s=w460, f=T7."Result") -> (s? t:f=w472:T7)
                        }
                        frame "MD[1]=1" {
                          n196 = call "Operation (SubVI).vi"("On/Off"=FALSE, "Operation"=T5."Venable", "DAQmx Device Name"=w510) -> ("error out"=w533:errorcluster)  [unwired: 8 in]
                          n197 = Concatenate Strings(w515, "\nSet Parameters MD[1]=1" ("Strin")) -> (w525:string)
                          n198 = call "Write panel message Kinetics (SubVI).vi"(4:"rpm"=w518, 5:"rpm"=FALSE ("rpm"), "PrintTime"=FALSE, "Stop"=w523, "error in (no error)"=w533, "Time to wait"=30.0, "Strin"=w525, "String in"=w524) -> ("error out"=w532:errorcluster, "Stopped"=w507:bool)  [unwired: 2 in]
                          n199 = call "Serial.vi"("error in (no error)"=w532, "write buffer"="EP=1\r\nVC=0\r\nMD[1]=1\r\n") -> ("error out"=w529:errorcluster)  [unwired: 8 in, 1 out]
                          n200 = call "Operation (SubVI).vi"("error in (no error)"=w529, "On/Off"=FALSE, "Operation"=T5."PowerSuply", "DAQmx Device Name"=w510) -> ("error out"=w528:errorcluster)  [unwired: 7 in]
                          n201 = call "Write panel message Kinetics (SubVI).vi"(4:"rpm"=w518, 5:"rpm"=FALSE ("rpm"), "PrintTime"=TRUE, "Stop"=w523, "error in (no error)"=w528, "Time to wait"=25.0, "Strin"=w525, "String in"=w524) -> ("error out"=w511:errorcluster, "Stopped"=w508:bool)  [unwired: 2 in]
                          n202 = call "Operation (SubVI).vi"("error in (no error)"=w511, "On/Off"=TRUE, "Operation"=T5."PowerSuply", "DAQmx Device Name"=w510) -> ("error out"=w512:errorcluster)  [unwired: 7 in]
                          n203 = call "Operation (SubVI).vi"("error in (no error)"=w512, "On/Off"=TRUE, "Operation"=T5."Venable", "DAQmx Device Name"=w510) -> ("error out"=w520:errorcluster)  [unwired: 7 in]
                          n204 = call "Write panel message Kinetics (SubVI).vi"(4:"rpm"=w518, 5:"rpm"=FALSE ("rpm"), "PrintTime"=TRUE, "Stop"=w523, "error in (no error)"=w520, "Time to wait"=3.0, "Strin"=w525, "String in"=w524) -> ("Stopped"=w509:bool)  [unwired: 2 in, 1 out]
                          n205 = Compound Arithmetic op=OR(w509, w508, w507) -> (w506:bool)
                          n206 = Compound Arithmetic op=OR(w509, w508, w507) -> (w517:bool)
                          n207 = Select(t=T7."Stop", s=w517, f=T7."FullSpeed2") -> (s? t:f=w546:T7)
                        }
                        frame "FullSpeed1" {
                          n208 = Search and Replace String(input string="EP=1\r\nVC=0\r\n" ("write buffer"), search string="0", replace string=w550) -> (result string=w549:string)  [unwired: 5 in, 3 out]
                          n209 = call "Serial.vi"("write buffer"=w549, "VISA resource name"=w553) -> ("error out"=w554:errorcluster)  [unwired: 8 in, 1 out]
                          n210 = Concatenate Strings(w548, "\nFull speed operation " ("string")) -> (w565:string)
                          n211 = call "Write panel message Kinetics (SubVI).vi"(4:"rpm"=w558, 5:"rpm"=TRUE ("rpm"), "PrintTime"=FALSE, "Stop"=w555, "error in (no error)"=w554, "Time to wait"=0.2, "Strin"=w565, "String in"=w556) -> ("error out"=w568:errorcluster, "Stopped"=w560:bool)  [unwired: 2 in]
                          n212 = flat-sequence {
                            tunnel: w568 -> [w575]
                            tunnel: [w575] -> w567
                            tunnel: [w574] -> w566
                            frame #0 {
                              n213 = call <vilib>:"High Resolution Relative Seconds.vi"() -> ("relative seconds"=w574:dbl)
                            }
                          }
                          n214 = while {
                            tunnel: w567 -> [w587]
                            tunnel: [w597] -> _
                            tunnel: w557 -> [w603]
                            tunnel: w566 -> [w601]
                            tunnel: w565 -> [w595]
                            tunnel: w558 -> [w580]
                            tunnel: w561 -> [w589]
                            tunnel: w560 -> [w588]
                            tunnel: [w576] -> w559
                            tunnel: w556 -> [w586]
                            tunnel: w555 -> [w585]
                            tunnel: [w576] -> w547
                            stop <- w604 stop-if-true
                            n215 = call <vilib>:"High Resolution Relative Seconds.vi"() -> ("relative seconds"=w602:dbl)
                            n216 = property class="DigNum (strict)"(reference=w580) -> ("Value"=w579:dbl)  [unwired: 1 in, 2 out]
                            n217 = Subtract(x=w602, y=w601) -> (x-y=w600:dbl)
                            n218 = call "Aquire AI"("error in"=w587, "device name"=w589) -> ("data"=w592:dynamicdata, "error out"=w591:errorcluster)  [unwired: 15 in, 1 out]
                            n219 = Greater Or Equal?(x=w600, y=120.0) -> (x >= y?=w598:bool)
                            n220 = To Double Precision Float(number=w592) -> (double precision float=w590:dbl)
                            "FullSpeed1 Current" <- w590
                            n221 = Multiply(x=25.0, y=w590) -> (x*y=w584:dbl)
                            n222 = Greater Or Equal?(x=w584, y=w603) -> (x >= y?=w582:bool)
                            n223 = Greater Or Equal?(x=w579, y=10000.0) -> (x >= y?=w577:bool)
                            n224 = And(x=w577, y=w582) -> (x .and. y?=w581:bool)
                            n225 = call "Write panel message Kinetics (SubVI).vi"(4:"rpm"=w580, 5:"rpm"=TRUE ("rpm"), "PrintTime"=FALSE, "Stop"=w585, "error in (no error)"=w591, "Time to wait"=0.2, "Strin"=w595, "String in"=w586) -> ("error out"=w597:errorcluster, "Stopped"=w576:bool)  [unwired: 2 in]
                            n226 = Compound Arithmetic op=OR(w576, w588, w598, w581) -> (w604:bool)
                          }
                          n227 = Select(t=T7."Stop", s=w559, f=T7."MD[1]=1") -> (s? t:f=w571:T7)
                        }
                        frame "MD[1]=0" {
                          n228 = call "Operation (SubVI).vi"("On/Off"=FALSE, "Operation"=T5."Venable", "DAQmx Device Name"=w610) -> ("error out"=w633:errorcluster)  [unwired: 8 in]
                          n229 = Concatenate Strings(w614, "\nSet Parameters MD[1]=0" ("Strin")) -> (w625:string)
                          n230 = call "Write panel message Kinetics (SubVI).vi"(4:"rpm"=w618, 5:"rpm"=FALSE ("rpm"), "PrintTime"=FALSE, "Stop"=w623, "error in (no error)"=w633, "Time to wait"=0.2, "Strin"=w625, "String in"=w624) -> ("error out"=w632:errorcluster, "Stopped"=w606:bool)  [unwired: 2 in]
                          n231 = call "Serial.vi"("error in (no error)"=w632, "write buffer"="EP=1\r\nVC=0\r\nMD[1]=0\r\n", "VISA resource name"=w615) -> ("error out"=w629:errorcluster)  [unwired: 7 in, 1 out]
                          n232 = call "Operation (SubVI).vi"("error in (no error)"=w629, "On/Off"=FALSE, "Operation"=T5."PowerSuply", "DAQmx Device Name"=w610) -> ("error out"=w628:errorcluster)  [unwired: 7 in]
                          n233 = call "Write panel message Kinetics (SubVI).vi"(4:"rpm"=w618, 5:"rpm"=FALSE ("rpm"), "PrintTime"=TRUE, "Stop"=w623, "error in (no error)"=w628, "Time to wait"=25.0, "Strin"=w625, "String in"=w624) -> ("error out"=w613:errorcluster, "Stopped"=w607:bool)  [unwired: 2 in]
                          n234 = call "Operation (SubVI).vi"("error in (no error)"=w613, "On/Off"=TRUE, "Operation"=T5."PowerSuply", "DAQmx Device Name"=w610) -> ("error out"=w612:errorcluster)  [unwired: 7 in]
                          n235 = call "Operation (SubVI).vi"("error in (no error)"=w612, "On/Off"=TRUE, "Operation"=T5."Venable", "DAQmx Device Name"=w610) -> ("error out"=w620:errorcluster)  [unwired: 7 in]
                          n236 = call "Write panel message Kinetics (SubVI).vi"(4:"rpm"=w618, 5:"rpm"=FALSE ("rpm"), "PrintTime"=TRUE, "Stop"=w623, "error in (no error)"=w620, "Time to wait"=3.0, "Strin"=w625, "String in"=w624) -> ("Stopped"=w608:bool)  [unwired: 2 in, 1 out]
                          n237 = Compound Arithmetic op=OR(w608, w607, w606) -> (w605:bool)
                          n238 = Compound Arithmetic op=OR(w608, w607, w606) -> (w617:bool)
                          n239 = Select(t=T7."Stop", s=w617, f=T7."FullSpeed1") -> (s? t:f=w646:T7)
                        }
                      }
                    }
                  }
                }
              }
            }
          }
        }
        frame "Venable Test" {
          n240 = control-ref of="Stop Button"() -> (w663:refnum<vi>)
          n241 = control-ref of="ATR"() -> (w664:refnum<vi>)
          n242 = control-ref of="Pannel User Message"() -> (w665:refnum<vi>)
          n243 = control-ref of="Motor Speed RPM Serial"() -> (w666:refnum<vi>)
          n244 = control-ref of="UUT"() -> (w667:refnum<vi>)
          n245 = Concatenate Strings(w659, " in process..." ("Strin")) -> (w660:string)
          n246 = while {
            shift-right: [w674] -> _
            shift-left: enum16{"Stop", "Direction", "Venable", "Start"}."Start" -> [w679]
            tunnel: w663 -> [w678]
            tunnel: w664 -> [w677]
            tunnel: w665 -> [w676]
            tunnel: w666 -> [w675]
            tunnel: w667 -> [w672]
            tunnel: w660 -> [w673]
            tunnel: w659 -> [w671]
            tunnel: w658 -> [w670]
            tunnel: [w668] -> w657
            stop <- w669 stop-if-true
            n247 = case shown="\"Start\"" w679 {
              tunnel: w678 -> [_ w709 w958 w1006]
              tunnel: w677 -> [_ w705 w956 w999]
              tunnel: w676 -> [_ w708 w959 w1012]
              tunnel: w675 -> [_ w707 w960 _]
              tunnel: w672 -> [w680 w701 w961 _]
              tunnel: [w682 FALSE FALSE FALSE] -> w669
              tunnel: [w681 w704 w957 w1010] -> w674
              tunnel: w673 -> [_ w706 w955 w1005]
              tunnel: w671 -> [_ _ _ w998]
              tunnel: w670 -> [_ _ _ w1001]
              tunnel: [_ _ _ w993] -> w668
              frame "Stop", Default {
                n248 = disable-structure shown="Enabled" {
                  disable-tunnel: [w685 TRUE] -> w682
                  disable-tunnel: [w684 enum16{"Stop", "Direction", "Venable", "Start"}."Stop"] -> w681
                  disable-tunnel: w680 -> [w683 _]
                  frame Disabled {
                    n249 = flat-sequence {
                      tunnel: w683 -> [_]
                      tunnel: [TRUE] -> w685
                      tunnel: [enum16{"Stop", "Direction", "Venable", "Start"}."Stop"] -> w684
                      frame #0 {
                        (unwired) u16 0 ("Motor Speed RPM")
                        (unwired) TRUE ("Remote")
                        n250 = property on="VISA Kinetics" class="VISAName"() -> (error out=w689:errorcluster, "Value"=w690:refnum<visa-resource-name>)  [unwired: 2 in, 1 out]
                        n251 = call "Serial.vi"("error in (no error)"=w689, "Clear Log"=FALSE, "write buffer"="EP=1\r\nMD[1]=1\r\n", "VISA resource name"=w690) -> ("error out"=w686:errorcluster)  [unwired: 6 in, 1 out]
                        n252 = call "CANSendMessage.vi"("error in (no error)"=w686) -> ("error out"=w695:errorcluster)  [unwired: 10 in]
                        n253 = call "TesterOption (SubVI).vi"("2 Options"=FALSE, "error in (no error)"=w695, "On/Off"=FALSE, "Tester Option"=T8."Venable") -> ("error out"=w691:errorcluster)  [unwired: 6 in, 1 out]
                        n254 = call "Time Delay9"("error in (no error)"=w691) -> ()  [unwired: 10 in, 1 out]
                      }
                      frame #1 {
                      }
                    }
                  }
                  frame Enabled {
                  }
                }
              }
              frame "Direction" {
                n255 = property on="UUT" class="DigNum (strict)"() -> ("Value"=w700:u8)  [unwired: 2 in, 2 out]
                n256 = while {
                  shift-right: [w720] -> w703
                  shift-left: T7."MD[1]=0" -> [w721]
                  tunnel: w701 -> [w718]
                  tunnel: w709 -> [w717]
                  tunnel: w708 -> [w716]
                  tunnel: w707 -> [w715]
                  tunnel: w706 -> [w714]
                  tunnel: w705 -> [w713]
                  tunnel: w700 -> [w712]
                  stop <- w719 stop-if-true
                  n257 = case shown="\"FullSpeed2\"" w721 {
                    tunnel: [T7."Stop" w745 w782 w852 w880 w950] -> w720
                    tunnel: [TRUE FALSE FALSE FALSE FALSE FALSE] -> w719
                    tunnel: w718 -> [_ _ _ _ _ _]
                    tunnel: w717 -> [_ w732 w759 w822 w860 w918]
                    tunnel: w716 -> [_ _ w758 w831 w859 w928]
                    tunnel: w715 -> [_ _ w775 w820 w874 w924]
                    tunnel: w714 -> [_ _ w770 w839 w872 w936]
                    tunnel: w713 -> [_ w736 _ _ _ _]
                    tunnel: w712 -> [_ w724 w756 _ w854 _]
                    frame "Stop", Default {
                    }
                    frame "Result" {
                      n258 = property on="FullSpeed1 Current" class="DigNum (strict)"() -> ("Value"=w740:dbl)  [unwired: 2 in, 2 out]
                      n259 = property on="FullSpeed2 Current" class="DigNum (strict)"() -> ("Value"=w741:dbl)  [unwired: 2 in, 2 out]
                      n260 = property on="FullSpeed2 Speed" class="DigNum (strict)"() -> ("Value"=w743:dbl)  [unwired: 2 in, 2 out]
                      n261 = property on="FullSpeed1 Speed" class="DigNum (strict)"() -> ("Value"=w742:dbl)  [unwired: 2 in, 2 out]
                      n262 = Subtract(x=w741, y=w740) -> (x-y=w739:dbl)
                      n263 = Absolute Value(x=w739) -> (abs(x)=w728:dbl)
                      n264 = Greater Or Equal?(x=w728, y=u32 5) -> (x >= y?=w734:bool)
                      n265 = Equal?(x=w724, y=u8 95) -> (x = y?=w726:bool)
                      n266 = case shown="True" w726 {
                        tunnel: w743 -> [_ w754]
                        tunnel: w742 -> [_ w753]
                        tunnel: [TRUE w750] -> w735
                        frame False {
                        }
                        frame True {
                          n267 = Subtract(x=w754, y=w753) -> (x-y=w755:dbl)
                          n268 = Absolute Value(x=w755) -> (abs(x)=w752:dbl)
                          n269 = Greater Or Equal?(x=w752, y=500.0) -> (x >= y?=w750:bool)
                        }
                      }
                      n270 = call "Find_Number_LineMARVIN.vi"("Test Paragraph"="Motor Rotation Direction", "TableIn"=w736) -> ("Line number"=w733:i32)  [unwired: 3 in, 3 out]
                      n271 = And(x=w735, y=w734) -> (x .and. y?=w725:bool)
                      "VenableDirectionResult" <- w725
                      n272 = call "PassOrFail (SubVI).vi"("String Res"="", "index (row)"=w733, "Data in"=-3.0, "Pass?Fail"=w725, "Table in"=w736) -> ("error out"=w731:errorcluster)  [unwired: 6 in]
                      n273 = property class="Bool (strict)"(reference=w732, error in=w731) -> ("Value"=w748:bool)  [unwired: 2 out]
                      n274 = Select(t=T7."Stop", s=w748, f=T7."Stop") -> (s? t:f=w745:T7)
                    }
                    frame "FullSpeed2" {
                      (unwired) TRUE ("Remote")
                      n275 = Concatenate Strings(w770, "\nFull speed operation " ("string")) -> (w757:string)
                      n276 = call "CANSendMessage.vi"() -> ("error out"=w777:errorcluster)  [unwired: 11 in]
                      n277 = call "Write panel message Kinetics (SubVI).vi"(4:"rpm"=w775, 5:"rpm"=TRUE ("rpm"), "PrintTime"=FALSE, "Stop"=w759, "error in (no error)"=w777, "Time to wait"=0.2, "Strin"=w757, "String in"=w758) -> ("error out"=w762:errorcluster)  [unwired: 2 in, 1 out]
                      n278 = Equal?(x=w756, y=u8 95) -> (x = y?=w765:bool)
                      n279 = Select(t=u16 15100, s=w765, f=u16 12100 ("y")) -> ()  [unwired: 1 out]
                      n280 = flat-sequence {
                        tunnel: w762 -> [w787]
                        tunnel: [w787] -> w761
                        tunnel: [w786] -> w760
                        frame #0 {
                          n281 = call <vilib>:"High Resolution Relative Seconds.vi"() -> ("relative seconds"=w786:dbl)
                        }
                      }
                      n282 = Select(t=14500.0, s=w765, f=11500.0) -> (s? t:f=w764:dbl)
                      n283 = Select(t=47.0, s=w765, f=24.0) -> (s? t:f=w763:dbl)
                      n284 = while {
                        tunnel: w775 -> [w789]
                        tunnel: w761 -> [w813]
                        tunnel: [w796] -> w772
                        tunnel: w764 -> [w809]
                        tunnel: w763 -> [w808]
                        tunnel: w760 -> [w804]
                        tunnel: w759 -> [w794]
                        tunnel: w758 -> [w795]
                        tunnel: w757 -> [w792]
                        stop <- w806 stop-if-true
                        n285 = call <vilib>:"High Resolution Relative Seconds.vi"() -> ("relative seconds"=w805:dbl)
                        n286 = Subtract(x=w805, y=w804) -> (x-y=w803:dbl)
                        n287 = property class="DigNum (strict)"(reference=w789, error in=w813) -> ("Value"=w810:dbl)  [unwired: 2 out]
                        "FullSpeed2 Speed" <- w810
                        n288 = Greater Or Equal?(x=w803, y=120.0) -> (x >= y?=w801:bool)
                        n289 = Greater Or Equal?(x=w810, y=w809) -> (x >= y?=w800:bool)
                        n290 = property class="Bool (strict)"(reference=w794) -> ("Value"=w799:bool)  [unwired: 1 in, 2 out]
                        n291 = call "GetADCTester (SubVI).vi"("GetADCTester"=T9."Current", "TimeToGet"=5) -> ("error out"=w811:errorcluster, "ADCValOutput Single"=w807:dbl)  [unwired: 7 in, 1 out]
                        "FullSpeed2 Current" <- w807
                        n292 = Greater Or Equal?(x=w807, y=w808) -> (x >= y?=w797:bool)
                        n293 = And(x=w800, y=w797) -> (x .and. y?=w798:bool)
                        n294 = Compound Arithmetic op=OR(w799, w801, w798) -> (w806:bool)
                        n295 = call "Write panel message Kinetics (SubVI).vi"(4:"rpm"=w789, 5:"rpm"=TRUE ("rpm"), "PrintTime"=FALSE, "Stop"=w794, "error in (no error)"=w811, "Time to wait"=0.2, "Strin"=w792, "String in"=w795) -> ("error out"=w796:errorcluster)  [unwired: 2 in, 1 out]
                      }
                      n296 = property class="Bool (strict)"(reference=w759, error in=w772) -> ("Value"=w785:bool)  [unwired: 2 out]
                      n297 = Select(t=T7."Stop", s=w785, f=T7."Result") -> (s? t:f=w782:T7)
                    }
                    frame "MD[1]=1" {
                      (unwired) TRUE ("Remote")
                      (unwired) u16 0 ("Motor Speed RPM")
                      n298 = Concatenate Strings(w839, "\nSet Parameters MD[1]=1" ("Strin")) -> (w830:string)
                      n299 = call "TesterOption (SubVI).vi"("2 Options"=FALSE, "On/Off"=FALSE, "Tester Option"=T8."Venable") -> ("error out"=w844:errorcluster, "VISA Refnum out"=w835:refnum<visa-resource-name>)  [unwired: 7 in]
                      n300 = call "CANSendMessage.vi"("error in (no error)"=w844) -> ("error out"=w846:errorcluster)  [unwired: 10 in]
                      n301 = call "Write panel message Kinetics (SubVI).vi"(4:"rpm"=w820, 5:"rpm"=FALSE ("rpm"), "PrintTime"=TRUE, "Stop"=w822, "error in (no error)"=w846, "Time to wait"=20.0, "Strin"=w830, "String in"=w831) -> ("error out"=w819:errorcluster)  [unwired: 2 in, 1 out]
                      n302 = property on="VISA Kinetics" class="VISAName"(error in=w819) -> (error out=w845:errorcluster, "Value"=w848:refnum<visa-resource-name>)  [unwired: 1 in, 1 out]
                      n303 = call "Serial.vi"("error in (no error)"=w845, "Clear Log"=FALSE, "write buffer"="EP=1\r\nMD[1]=1\r\n", "VISA resource name"=w848) -> ("error out"=w834:errorcluster)  [unwired: 6 in, 1 out]
                      n304 = call "TesterOption (SubVI).vi"("2 Options"=FALSE, "error in (no error)"=w834, "On/Off"=FALSE, "Tester Option"=T8."Power", "VISA Refnum in"=w835) -> ("error out"=w832:errorcluster, "VISA Refnum out"=w823:refnum<visa-resource-name>)  [unwired: 5 in]
                      n305 = call "Write panel message Kinetics (SubVI).vi"(4:"rpm"=w820, 5:"rpm"=FALSE ("rpm"), "PrintTime"=TRUE, "Stop"=w822, "error in (no error)"=w832, "Time to wait"=25.0, "Strin"=w830, "String in"=w831) -> ("error out"=w824:errorcluster)  [unwired: 2 in, 1 out]
                      n306 = call "TesterOption (SubVI).vi"("2 Options"=FALSE, "error in (no error)"=w824, "On/Off"=TRUE, "Tester Option"=T8."Venable", "VISA Refnum in"=w823) -> ("error out"=w821:errorcluster)  [unwired: 5 in, 1 out]
                      n307 = call "Time Delay8"("error in (no error)"=w821) -> ("error out"=w817:errorcluster)  [unwired: 10 in]
                      n308 = property class="Bool (strict)"(reference=w822, error in=w817) -> ("Value"=w853:bool)  [unwired: 2 out]
                      n309 = Select(t=T7."Stop", s=w853, f=T7."FullSpeed2") -> (s? t:f=w852:T7)
                    }
                    frame "FullSpeed1" {
                      (unwired) TRUE ("Remote")
                      n310 = call "CANSendMessage.vi"() -> ("error out"=w875:errorcluster)  [unwired: 11 in]
                      n311 = Concatenate Strings(w872, "\nFull speed operation " ("string")) -> (w858:string)
                      n312 = call "Write panel message Kinetics (SubVI).vi"(4:"rpm"=w874, 5:"rpm"=TRUE ("rpm"), "PrintTime"=FALSE, "Stop"=w860, "error in (no error)"=w875, "Time to wait"=0.2, "Strin"=w858, "String in"=w859) -> ("error out"=w863:errorcluster)  [unwired: 2 in, 1 out]
                      n313 = Equal?(x=w854, y=u8 95) -> (x = y?=w870:bool)
                      n314 = flat-sequence {
                        tunnel: w863 -> [w885]
                        tunnel: [w885] -> w862
                        tunnel: [w884] -> w861
                        frame #0 {
                          n315 = call <vilib>:"High Resolution Relative Seconds.vi"() -> ("relative seconds"=w884:dbl)
                        }
                      }
                      n316 = Select(t=u16 15100, s=w870, f=u16 12100 ("y")) -> ()  [unwired: 1 out]
                      n317 = Select(t=13700.0, s=w870, f=11500.0) -> (s? t:f=w865:dbl)
                      n318 = Select(t=56.0, s=w870, f=33.0) -> (s? t:f=w864:dbl)
                      n319 = while {
                        tunnel: w874 -> [w887]
                        tunnel: w862 -> [w911]
                        tunnel: [w894] -> w873
                        tunnel: w865 -> [w906]
                        tunnel: w864 -> [w903]
                        tunnel: w861 -> [w901]
                        tunnel: w860 -> [w892]
                        tunnel: w859 -> [w893]
                        tunnel: w858 -> [w890]
                        stop <- w908 stop-if-true
                        n320 = property class="DigNum (strict)"(reference=w887, error in=w911) -> ("Value"=w907:dbl)  [unwired: 2 out]
                        "FullSpeed1 Speed" <- w907
                        n321 = call <vilib>:"High Resolution Relative Seconds.vi"() -> ("relative seconds"=w902:dbl)
                        n322 = Subtract(x=w902, y=w901) -> (x-y=w900:dbl)
                        n323 = Greater Or Equal?(x=w900, y=120.0) -> (x >= y?=w898:bool)
                        n324 = Greater Or Equal?(x=w907, y=w906) -> (x >= y?=w905:bool)
                        n325 = call "GetADCTester (SubVI).vi"("GetADCTester"=T9."Current", "TimeToGet"=5) -> ("error out"=w909:errorcluster, "ADCValOutput Single"=w904:dbl)  [unwired: 7 in, 1 out]
                        "FullSpeed1 Current" <- w904
                        n326 = Greater Or Equal?(x=w904, y=w903) -> (x >= y?=w895:bool)
                        n327 = And(x=w895, y=w905) -> (x .and. y?=w896:bool)
                        n328 = property class="Bool (strict)"(reference=w892) -> ("Value"=w897:bool)  [unwired: 1 in, 2 out]
                        n329 = call "Write panel message Kinetics (SubVI).vi"(4:"rpm"=w887, 5:"rpm"=TRUE ("rpm"), "PrintTime"=FALSE, "Stop"=w892, "error in (no error)"=w909, "Time to wait"=0.2, "Strin"=w890, "String in"=w893) -> ("error out"=w894:errorcluster)  [unwired: 2 in, 1 out]
                        n330 = Compound Arithmetic op=OR(w897, w896, w898) -> (w908:bool)
                      }
                      n331 = property class="Bool (strict)"(reference=w860, error in=w873) -> ("Value"=w883:bool)  [unwired: 2 out]
                      n332 = Select(t=T7."Stop", s=w883, f=T7."MD[1]=1") -> (s? t:f=w880:T7)
                    }
                    frame "MD[1]=0" {
                      (unwired) TRUE ("Remote")
                      (unwired) u16 0 ("Motor Speed RPM")
                      n333 = Concatenate Strings(w936, "\nSet Parameters MD[1]=0" ("Strin")) -> (w927:string)
                      n334 = call "TesterOption (SubVI).vi"("2 Options"=FALSE, "On/Off"=FALSE, "Tester Option"=T8."Venable") -> ("error out"=w942:errorcluster, "VISA Refnum out"=w932:refnum<visa-resource-name>)  [unwired: 7 in]
                      n335 = call "CANSendMessage.vi"("error in (no error)"=w942) -> ("error out"=w944:errorcluster)  [unwired: 10 in]
                      n336 = call "Write panel message Kinetics (SubVI).vi"(4:"rpm"=w924, 5:"rpm"=FALSE ("rpm"), "PrintTime"=FALSE, "Stop"=w918, "error in (no error)"=w944, "Time to wait"=0.2, "Strin"=w927, "String in"=w928) -> ("error out"=w939:errorcluster)  [unwired: 2 in, 1 out]
                      n337 = property on="VISA Kinetics" class="VISAName"(error in=w939) -> (error out=w943:errorcluster, "Value"=w946:refnum<visa-resource-name>)  [unwired: 1 in, 1 out]
                      n338 = call "Serial.vi"("error in (no error)"=w943, "Clear Log"=FALSE, "write buffer"="EP=1\r\nMD[1]=0\r\n", "VISA resource name"=w946) -> ("error out"=w931:errorcluster)  [unwired: 6 in, 1 out]
                      n339 = call "TesterOption (SubVI).vi"("2 Options"=FALSE, "error in (no error)"=w931, "On/Off"=FALSE, "Tester Option"=T8."Power", "VISA Refnum in"=w932) -> ("error out"=w929:errorcluster, "VISA Refnum out"=w919:refnum<visa-resource-name>)  [unwired: 5 in]
                      n340 = call "Write panel message Kinetics (SubVI).vi"(4:"rpm"=w924, 5:"rpm"=FALSE ("rpm"), "PrintTime"=TRUE, "Stop"=w918, "error in (no error)"=w929, "Time to wait"=25.0, "Strin"=w927, "String in"=w928) -> ("error out"=w920:errorcluster)  [unwired: 2 in, 1 out]
                      n341 = call "TesterOption (SubVI).vi"("2 Options"=FALSE, "error in (no error)"=w920, "On/Off"=TRUE, "Tester Option"=T8."Venable", "VISA Refnum in"=w919) -> ("error out"=w917:errorcluster)  [unwired: 5 in, 1 out]
                      n342 = call "Time Delay4"("error in (no error)"=w917) -> ("error out"=w913:errorcluster)  [unwired: 10 in]
                      n343 = property class="Bool (strict)"(reference=w918, error in=w913) -> ("Value"=w951:bool)  [unwired: 2 out]
                      n344 = Select(t=T7."Stop", s=w951, f=T7."FullSpeed1") -> (s? t:f=w950:T7)
                    }
                  }
                }
                n345 = flat-sequence {
                  tunnel: [enum16{"Stop", "Direction", "Venable", "Start"}."Stop"] -> w704
                  tunnel: w703 -> [_]
                  frame #0 {
                  }
                }
              }
              frame "Venable" {
                n346 = call "Find_Number_LineMARVIN.vi"("Test Paragraph"="Enable Test", "TableIn"=w956) -> ("Line number"=w962:i32)  [unwired: 3 in, 3 out]
                n347 = Increment(x=w962) -> (x+1=w952:i32)
                n348 = for {
                  tunnel: u16[] [5000, 0, 5000] -> [w987] mode=indexing
                  tunnel: bool[] [TRUE, FALSE, TRUE] -> [w985] mode=indexing
                  tunnel: w952 -> [w988]
                  tunnel: w961 -> [_]
                  tunnel: w960 -> [w978]
                  tunnel: w959 -> [w981]
                  tunnel: w958 -> [w980]
                  tunnel: w956 -> [w974]
                  tunnel: w955 -> [w972]
                  tunnel: [w971] -> w954 mode=indexing
                  i -> [w989]
                  (unwired) u16 5000 ("Motor Speed RPM")
                  (unwired) TRUE ("Remote")
                  w990 = 200.0 ("y")
                  n349 = call "CANSendMessage.vi"() -> ("error out"=w984:errorcluster)  [unwired: 11 in]
                  n350 = Add(x=w988, y=w989) -> (x+y=w975:i32)
                  n351 = call "TesterOption (SubVI).vi"("2 Options"=FALSE, "error in (no error)"=w984, "On/Off"=w985, "Tester Option"=T8."Venable") -> ("error out"=w983:errorcluster)  [unwired: 6 in, 1 out]
                  n352 = call "Write panel message Kinetics (SubVI).vi"(4:"rpm"=w978, 5:"rpm"=TRUE ("rpm"), "PrintTime"=TRUE, "Stop"=w980, "error in (no error)"=w983, "Time to wait"=15.0, "Strin"=w972, "String in"=w981) -> ("error out"=w982:errorcluster)  [unwired: 2 in, 1 out]
                  n353 = property class="DigNum (strict)"(reference=w978, error in=w982) -> ("Value"=w973:dbl)  [unwired: 2 out]
                  n354 = Add(x=w987, y=w990) -> (x+y=w992:dbl)
                  n355 = Subtract(x=w987, y=w990) -> (x-y=w991:dbl)
                  n356 = In Range and Coerce(upper limit=w992, x=w973, lower limit=w991) -> (In Range?=w971:bool)  [unwired: 1 out]
                  n357 = call "PassOrFail (SubVI).vi"("index (row)"=w975, "Data in"=w973, "Pass?Fail"=w971, "Table in"=w974) -> ()  [unwired: 7 in, 1 out]
                }
                n358 = property class="Bool (strict)"(reference=w958) -> ("Value"=w969:bool)  [unwired: 1 in, 2 out]
                n359 = And Array Elements(Boolean array=w954) -> (logical AND=→"VenableResult":bool)
                n360 = Select(t=enum16{"Stop", "Direction", "Venable", "Start"}."Stop", s=w969, f=enum16{"Stop", "Direction", "Venable", "Start"}."Direction") -> (s? t:f=w957:enum16{"Stop", "Direction", "Venable", "Start"})
              }
              frame "Start" {
                n361 = property class="Str"(reference=w1012, "Value"=w1005) -> (error out=w1009:errorcluster)  [unwired: 1 in, 1 out]
                n362 = call "Find_Number_LineMARVIN.vi"("Test Paragraph"=w998, "error in"=w1009, "TableIn"=w999) -> ("error out"=w1000:errorcluster, "Line number"=w997:i32)  [unwired: 2 in, 2 out]
                n363 = call "Table_ScrollaBarMarvin.vi"("error in"=w1000, "Line to focus"=w998, "reference in"=w999) -> ("error out"=w1013:errorcluster)  [unwired: 2 out]
                n364 = call "Reset old test Values (SubVI) Kinetics.vi"("error in"=w1013, "Atr in"=w999, "Test Paragraph"=w998) -> ("error out"=w994:errorcluster)  [unwired: 6 in, 2 out]
                n365 = Increment(x=w997) -> (x+1=w996:i32)
                n366 = while {
                  shift-right: [w1025] -> _
                  shift-left: T6."VC=1000" -> [w1028]
                  tunnel: w994 -> [w1027]
                  tunnel: w1001 -> [w1026]
                  tunnel: w998 -> [w1024]
                  shift-right: [w1021] -> w1004
                  shift-left: bool[] [FALSE, FALSE] -> [w1022]
                  tunnel: w996 -> [w1020]
                  tunnel: w999 -> [w1019]
                  shift-right: [w1017] -> _
                  shift-left: dbl[] [0.0, 0.0] -> [w1018]
                  tunnel: [w1015] -> w993
                  i -> [w1023]
                  stop <- w1016 stop-if-true
                  n367 = case shown="\"Wait\"" w1028 {
                    tunnel: w1027 -> [_ w1046 _ w1092 _]
                    tunnel: w1026 -> [_ w1045 w1061 w1096 _]
                    tunnel: [T6."Exit" T6."Wait" w1058 T6."Wait" T6."ReadVC"] -> w1025
                    tunnel: w1024 -> [_ _ _ _ w1103]
                    tunnel: [TRUE FALSE FALSE FALSE w1098] -> w1016
                    tunnel: w1023 -> [_ _ w1059 _ _]
                    tunnel: w1022 -> [w1030 w1043 w1057 w1094 w1100]
                    tunnel: [w1030 w1043 w1056 w1094 w1100] -> w1021
                    tunnel: w1020 -> [w1031 _ _ _ _]
                    tunnel: w1019 -> [w1032 _ _ _ _]
                    tunnel: w1018 -> [w1029 w1041 w1054 w1087 w1099]
                    tunnel: [w1029 w1041 w1053 w1087 w1099] -> w1017
                    tunnel: [_ _ _ _ w1098] -> w1015
                    frame "Exit", Default {
                      n368 = for {
                        tunnel: w1032 -> [w1040]
                        tunnel: w1031 -> [w1039]
                        tunnel: w1030 -> [w1038] mode=indexing
                        tunnel: w1029 -> [w1035] mode=indexing
                        i -> [w1036]
                        n369 = Add(x=w1036, y=w1039) -> (x+y=w1037:i32)
                        n370 = call "PassOrFail (SubVI).vi"("index (row)"=w1037, "Data in"=w1035, "Pass?Fail"=w1038, "Table in"=w1040) -> ()  [unwired: 7 in, 1 out]
                      }
                    }
                    frame "VC=0" {
                      n371 = disable-structure shown="Enabled" {
                        disable-tunnel: w1046 -> [w1049 _]
                        disable-tunnel: w1045 -> [w1047 _]
                        frame Disabled {
                          n372 = call "Serial.vi"("error in (no error)"=w1049, "write buffer"="EP=1\r\nVC=0\r\n", "VISA resource name"=w1047) -> ()  [unwired: 7 in, 2 out]
                        }
                        frame Enabled {
                          n373 = local read "DAQmx Device Name"() -> (w1052:tag)
                          n374 = call "Operation (SubVI).vi"("On/Off"=FALSE, "Operation"=T5."Venable", "DAQmx Device Name"=w1052) -> ()  [unwired: 8 in, 1 out]
                        }
                      }
                    }
                    frame "ReadVC" {
                      n375 = call "Serial.vi"("write buffer"="VC\r\n", "VISA resource name"=w1061) -> ("read buffer"=w1060:string)  [unwired: 8 in, 1 out]
                      n376 = case shown="5, Default" w1059 {
                        tunnel: w1060 -> [w1073 w1083]
                        tunnel: [T6."VC=0" T6."Exit"] -> w1058
                        tunnel: w1057 -> [w1069 w1082]
                        tunnel: [w1067 w1079] -> w1056
                        tunnel: w1054 -> [w1066 w1078]
                        tunnel: [w1063 w1075] -> w1053
                        frame 2 {
                          n377 = Decimal String To Number(string=w1073) -> (number=w1064:i32)  [unwired: 2 in, 1 out]
                          n378 = In Range and Coerce(upper limit=1100, x=w1064, lower limit=900) -> (In Range?=w1068:bool)  [unwired: 1 out]
                          n379 = Replace Array Subset(array=w1066, new element=w1064, index=0) -> (w1063:dbl[])
                          n380 = Replace Array Subset(array=w1069, new element=w1068, index=0) -> (w1067:bool[])
                        }
                        frame 5, Default {
                          n381 = Decimal String To Number(string=w1083) -> (number=w1076:i32)  [unwired: 2 in, 1 out]
                          n382 = In Range and Coerce(upper limit=100, x=w1076, lower limit=0) -> (In Range?=w1080:bool)  [unwired: 1 out]
                          n383 = Replace Array Subset(array=w1078, new element=w1076, index=1) -> (w1075:dbl[])
                          n384 = Replace Array Subset(array=w1082, new element=w1080, index=1) -> (w1079:bool[])
                        }
                      }
                    }
                    frame "VC=1000" {
                      n385 = local read "DAQmx Device Name"() -> (w1093:tag)
                      n386 = call "Operation (SubVI).vi"("error in (no error)"=w1092, "On/Off"=TRUE, "Operation"=T5."Venable", "DAQmx Device Name"=w1093) -> ("error out"=w1091:errorcluster)  [unwired: 7 in]
                      n387 = call "Serial.vi"("error in (no error)"=w1091, "write buffer"="EP=1\r\nVC=1000\r\n", "VISA resource name"=w1096) -> ()  [unwired: 7 in, 2 out]
                    }
                    frame "Wait" {
                      n388 = control-ref of="Motor Speed RPM Serial"() -> (w1108:refnum<vi>)
                      n389 = control-ref of="Pannel User Message"() -> (w1107:refnum<vi>)
                      n390 = control-ref of="Stop Button"() -> (w1102:refnum<vi>)
                      n391 = call "Write panel message Kinetics (SubVI).vi"(4:"rpm"=w1108, 5:"rpm"=TRUE ("rpm"), "PrintTime"=TRUE, "Stop"=w1102, "Time to wait"=20.0, "Strin"=w1103, "String in"=w1107) -> ("Stopped"=w1098:bool)  [unwired: 3 in, 1 out]
                    }
                  }
                }
                n392 = And Array Elements(Boolean array=w1004) -> ()  [unwired: 1 out]
                n393 = property class="Bool (strict)"(reference=w1006) -> ("Value"=w1014:bool)  [unwired: 1 in, 2 out]
                n394 = Select(t=enum16{"Stop", "Direction", "Venable", "Start"}."Stop", s=w1014, f=enum16{"Stop", "Direction", "Venable", "Start"}."Stop") -> (s? t:f=w1010:enum16{"Stop", "Direction", "Venable", "Start"})
              }
            }
          }
        }
        frame "Motor Thermistor Test" {
          n395 = Concatenate Strings(w1120, " in process..." ("Strin")) -> (w1121:string)
          n396 = control-ref of="ATR"() -> (w1123:refnum<vi>)
          n397 = control-ref of="Pannel User Message"() -> (w1124:refnum<vi>)
          n398 = property class="Str"(reference=w1124, "Value"=w1121) -> (error out=w1117:errorcluster)  [unwired: 1 in, 1 out]
          n399 = call "Find_Number_LineMARVIN.vi"("Test Paragraph"=w1120, "error in"=w1117, "TableIn"=w1123) -> ("error out"=w1114:errorcluster, "Line number"=w1113:i32)  [unwired: 2 in, 2 out]
          n400 = call "Table_ScrollaBarMarvin.vi"("error in"=w1114, "Line to focus"=w1120, "reference in"=w1123) -> ("error out"=w1118:errorcluster)  [unwired: 2 out]
          n401 = call "Reset old test Values (SubVI) Kinetics.vi"("error in"=w1118, "Atr in"=w1123, "Test Paragraph"=w1120) -> ("error out"=w1110:errorcluster)  [unwired: 6 in, 2 out]
          n402 = Increment(x=w1113) -> (x+1=w1112:i32)
          n403 = while {
            shift-right: [w1135] -> _
            shift-left: T6."VC=1000" -> [w1138]
            tunnel: w1110 -> [w1137]
            tunnel: w1119 -> [w1136]
            tunnel: w1120 -> [w1134]
            shift-right: [w1130] -> _
            shift-left: bool[] [FALSE, FALSE] -> [w1131]
            tunnel: w1112 -> [w1129]
            tunnel: w1123 -> [w1128]
            shift-right: [w1126] -> _
            shift-left: dbl[] [0.0, 0.0] -> [w1127]
            tunnel: [w1125] -> w1109
            i -> [w1132]
            stop <- w1133 stop-if-true
            n404 = case shown="\"Wait\"" w1138 {
              tunnel: w1137 -> [_ w1162 _ w1219 _]
              tunnel: w1136 -> [w1139 w1161 w1178 w1223 _]
              tunnel: [T6."Exit" T6."Wait" w1175 T6."Wait" T6."ReadVC"] -> w1135
              tunnel: w1134 -> [_ _ _ _ w1230]
              tunnel: [TRUE FALSE FALSE FALSE w1225] -> w1133
              tunnel: w1132 -> [_ w1156 w1176 _ _]
              tunnel: w1131 -> [w1145 w1159 w1174 w1221 w1227]
              tunnel: [w1145 w1159 w1173 w1221 w1227] -> w1130
              tunnel: w1129 -> [w1146 _ _ _ _]
              tunnel: w1128 -> [w1147 _ _ _ _]
              tunnel: w1127 -> [w1144 w1157 w1171 w1214 w1226]
              tunnel: [w1144 w1157 w1170 w1214 w1226] -> w1126
              tunnel: [_ _ _ _ w1225] -> w1125
              frame "Exit", Default {
                n405 = for {
                  tunnel: w1147 -> [w1155]
                  tunnel: w1146 -> [w1154]
                  tunnel: w1145 -> [w1153] mode=indexing
                  tunnel: w1144 -> [w1150] mode=indexing
                  i -> [w1151]
                  n406 = Add(x=w1151, y=w1154) -> (x+y=w1152:i32)
                  n407 = call "PassOrFail (SubVI).vi"("index (row)"=w1152, "Data in"=w1150, "Pass?Fail"=w1153, "Table in"=w1155) -> ()  [unwired: 7 in, 1 out]
                }
                n408 = local read "DAQmx Device Name"() -> (w1143:tag)
                n409 = call "Serial.vi"("write buffer"="EP=1\r\nVC=0\r\n", "VISA resource name"=w1139) -> ()  [unwired: 8 in, 2 out]
                n410 = call "Operation (SubVI).vi"("On/Off"=FALSE, "Operation"=T5."Venable", "DAQmx Device Name"=w1143) -> ()  [unwired: 8 in, 1 out]
              }
              frame "VC=0" {
                n411 = disable-structure shown="Enabled" {
                  disable-tunnel: w1162 -> [w1165 _]
                  disable-tunnel: w1161 -> [w1163 _]
                  disable-tunnel: w1156 -> [_ w1166]
                  frame Disabled {
                    n412 = call "Serial.vi"("error in (no error)"=w1165, "write buffer"="EP=1\r\nVC=0\r\n", "VISA resource name"=w1163) -> ()  [unwired: 7 in, 2 out]
                  }
                  frame Enabled {
                    n413 = case shown="6, Default" w1166 {
                      tunnel: ["Connect wires of the thermistor" ("message") "Disconnect wires of the thermistor" ("message")] -> w1167
                      frame 6, Default {
                      }
                      frame 3 {
                      }
                    }
                    n414 = One Button Dialog(message=w1167) -> ()  [unwired: 1 in, 1 out]
                  }
                }
              }
              frame "ReadVC" {
                n415 = call "Serial.vi"("write buffer"="VC\r\n", "VISA resource name"=w1178) -> ("read buffer"=w1177:string)  [unwired: 8 in, 1 out]
                n416 = case shown="2" w1176 {
                  tunnel: w1177 -> [w1189 w1198 w1210]
                  tunnel: [w1183 T6."VC=0" T6."Exit"] -> w1175
                  tunnel: w1174 -> [w1180 w1197 w1209]
                  tunnel: [w1180 w1194 w1206] -> w1173
                  tunnel: w1171 -> [w1181 w1193 w1205]
                  tunnel: [w1181 w1190 w1202] -> w1170
                  frame 2 {
                    n417 = Decimal String To Number(string=w1189) -> (number=w1186:i32)  [unwired: 2 in, 1 out]
                    n418 = In Range and Coerce(upper limit=1100, x=w1186, lower limit=900) -> (In Range?=w1185:bool)  [unwired: 1 out]
                    n419 = Select(t=T6."VC=0", s=w1185, f=T6."Exit") -> (s? t:f=w1183:T6)
                  }
                  frame 5, Default {
                    n420 = Decimal String To Number(string=w1198) -> (number=w1191:i32)  [unwired: 2 in, 1 out]
                    n421 = In Range and Coerce(upper limit=100, x=w1191, lower limit=0) -> (In Range?=w1195:bool)  [unwired: 1 out]
                    n422 = Replace Array Subset(array=w1193, new element=w1191, index=0) -> (w1190:dbl[])
                    n423 = Replace Array Subset(array=w1197, new element=w1195, index=0) -> (w1194:bool[])
                  }
                  frame 8 {
                    n424 = Decimal String To Number(string=w1210) -> (number=w1203:i32)  [unwired: 2 in, 1 out]
                    n425 = In Range and Coerce(upper limit=1100, x=w1203, lower limit=900) -> (In Range?=w1207:bool)  [unwired: 1 out]
                    n426 = Replace Array Subset(array=w1205, new element=w1203, index=1) -> (w1202:dbl[])
                    n427 = Replace Array Subset(array=w1209, new element=w1207, index=1) -> (w1206:bool[])
                  }
                }
              }
              frame "VC=1000" {
                n428 = local read "DAQmx Device Name"() -> (w1220:tag)
                n429 = call "Operation (SubVI).vi"("error in (no error)"=w1219, "On/Off"=TRUE, "Operation"=T5."Venable", "DAQmx Device Name"=w1220) -> ("error out"=w1218:errorcluster)  [unwired: 7 in]
                n430 = call "Serial.vi"("error in (no error)"=w1218, "write buffer"="EP=1\r\nVC=1000\r\n", "VISA resource name"=w1223) -> ()  [unwired: 7 in, 2 out]
              }
              frame "Wait" {
                n431 = control-ref of="Motor Speed RPM Serial"() -> (w1235:refnum<vi>)
                n432 = control-ref of="Pannel User Message"() -> (w1234:refnum<vi>)
                n433 = control-ref of="Stop Button"() -> (w1229:refnum<vi>)
                n434 = call "Write panel message Kinetics (SubVI).vi"(4:"rpm"=w1235, 5:"rpm"=TRUE ("rpm"), "PrintTime"=TRUE, "Stop"=w1229, "Time to wait"=20.0, "Strin"=w1230, "String in"=w1234) -> ("Stopped"=w1225:bool)  [unwired: 3 in, 1 out]
              }
            }
          }
        }
        frame "Up/Down Blower Test" {
          n435 = control-ref of="Pannel User Message"() -> (w1256:refnum<vi>)
          n436 = Concatenate Strings(w1247, " in process..." ("Strin")) -> (w1248:string)
          n437 = property class="Str"(reference=w1256, error in=w1255, "Value"=w1248) -> (error out=w1254:errorcluster)  [unwired: 1 out]
          n438 = call "Table_ScrollaBarMarvin.vi"("error in"=w1254, "Line to focus"=w1247, "reference in"=w1240) -> ()  [unwired: 3 out]
          n439 = call "Reset old test Values (SubVI) Kinetics.vi"("Atr in"=w1240, "Test Paragraph"=w1247) -> ("error out"=w1249:errorcluster)  [unwired: 7 in, 2 out]
          n440 = call "Find_Number_LineMARVIN.vi"("Test Paragraph"=w1247, "error in"=w1249, "TableIn"=w1240) -> ("error out"=w1244:errorcluster, "Line number"=w1246:i32)  [unwired: 2 in, 2 out]
          n441 = Increment(x=w1246) -> (x+1=w1239:i32)
          n442 = call "Serial.vi"("error in (no error)"=w1244, "write buffer"="VM[1]\r\n", "VISA resource name"=w1243) -> ("error out"=w1242:errorcluster, "read buffer"=w1237:string)  [unwired: 7 in]
          n443 = call "InsertSingleData.vi"("String In"=w1237, "error in (no error)"=w1242, "Col"=2, "Row"=w1239, "Table in"=w1240) -> ("error out"=w1241:errorcluster)  [unwired: 6 in]
          n444 = while {
            shift-right: [w1268] -> _
            shift-left: T6."VC=1000" -> [w1271]
            tunnel: w1241 -> [w1270]
            tunnel: w1243 -> [w1269]
            tunnel: w1248 -> [w1267]
            shift-right: [w1264] -> _
            shift-left: bool[] [FALSE, FALSE] -> [w1265]
            tunnel: w1239 -> [w1263]
            tunnel: w1240 -> [w1262]
            shift-right: [w1260] -> _
            shift-left: dbl[] [0.0, 0.0] -> [w1261]
            tunnel: w1237 -> [w1259]
            tunnel: [w1257] -> w1236
            i -> [w1266]
            stop <- w1258 stop-if-true
            n445 = case shown="\"Wait\"" w1271 {
              tunnel: w1270 -> [_ w1292 _ w1352 _]
              tunnel: w1269 -> [_ w1291 w1308 w1355 _]
              tunnel: [T6."Exit" T6."Wait" w1305 T6."Wait" T6."ReadVC"] -> w1268
              tunnel: w1267 -> [_ _ _ _ w1362]
              tunnel: [TRUE FALSE FALSE FALSE w1357] -> w1258
              tunnel: w1266 -> [_ _ w1306 _ _]
              tunnel: w1265 -> [w1276 w1289 w1304 w1353 w1359]
              tunnel: [w1276 w1289 w1303 w1353 w1359] -> w1264
              tunnel: w1263 -> [w1277 _ _ _ _]
              tunnel: w1262 -> [w1278 _ _ _ _]
              tunnel: w1261 -> [w1275 w1287 w1301 w1347 w1358]
              tunnel: [w1275 w1287 w1300 w1347 w1358] -> w1260
              tunnel: w1259 -> [_ _ w1299 _ _]
              tunnel: [_ _ _ _ w1357] -> w1257
              frame "Exit", Default {
                n446 = for {
                  tunnel: w1278 -> [w1286]
                  tunnel: w1277 -> [w1285]
                  tunnel: w1276 -> [w1284] mode=indexing
                  tunnel: w1275 -> [w1281] mode=indexing
                  i -> [w1282]
                  n447 = Add(x=w1282, y=w1285) -> (x+y=w1283:i32)
                  n448 = call "PassOrFail (SubVI).vi"("index (row)"=w1283, "Data in"=w1281, "Pass?Fail"=w1284, "Table in"=w1286) -> ()  [unwired: 7 in, 1 out]
                }
                n449 = local read "DAQmx Device Name"() -> (w1274:tag)
                n450 = call "Operation (SubVI).vi"("On/Off"=FALSE, "Operation"=T5."Venable", "DAQmx Device Name"=w1274) -> ()  [unwired: 8 in, 1 out]
              }
              frame "VC=0" {
                n451 = disable-structure shown="Enabled" {
                  disable-tunnel: w1292 -> [w1295 _]
                  disable-tunnel: w1291 -> [w1293 _]
                  frame Disabled {
                    n452 = call "Serial.vi"("error in (no error)"=w1295, "write buffer"="EP=1\r\nVC=0\r\n", "VISA resource name"=w1293) -> ()  [unwired: 7 in, 2 out]
                  }
                  frame Enabled {
                    n453 = local read "DAQmx Device Name"() -> (w1298:tag)
                    n454 = call "Operation (SubVI).vi"("On/Off"=TRUE, "Operation"=T5."Down", "DAQmx Device Name"=w1298) -> ()  [unwired: 8 in, 1 out]
                  }
                }
              }
              frame "ReadVC" {
                n455 = call "Serial.vi"("write buffer"="VC\r\n", "VISA resource name"=w1308) -> ("read buffer"=w1307:string)  [unwired: 8 in, 1 out]
                n456 = case shown="5, Default" w1306 {
                  tunnel: w1307 -> [w1326 w1339]
                  tunnel: [T6."VC=0" T6."Exit"] -> w1305
                  tunnel: w1304 -> [w1324 w1338]
                  tunnel: [w1322 w1335] -> w1303
                  tunnel: w1301 -> [w1321 w1334]
                  tunnel: [w1319 w1331] -> w1300
                  tunnel: w1299 -> [w1313 _]
                  frame 2 {
                    w1314 = 100
                    n457 = Decimal String To Number(string=w1326) -> (number=w1315:i32)  [unwired: 2 in, 1 out]
                    n458 = Decimal String To Number(string=w1313) -> (number=w1310:i32)  [unwired: 2 in, 1 out]
                    n459 = Add(x=w1310, y=w1314) -> (x+y=w1312:i32)
                    n460 = Subtract(x=w1310, y=w1314) -> (x-y=w1311:i32)
                    n461 = In Range and Coerce(upper limit=w1312, x=w1315, lower limit=w1311) -> (In Range?=w1323:bool)  [unwired: 1 out]
                    n462 = Replace Array Subset(array=w1321, new element=w1315, index=0) -> (w1319:dbl[])
                    n463 = Replace Array Subset(array=w1324, new element=w1323, index=0) -> (w1322:bool[])
                    n464 = local read "DAQmx Device Name"() -> (w1318:tag)
                    n465 = call "Operation (SubVI).vi"("On/Off"=FALSE, "Operation"=T5."Up", "DAQmx Device Name"=w1318) -> ()  [unwired: 8 in, 1 out]
                  }
                  frame 5, Default {
                    n466 = Decimal String To Number(string=w1339) -> (number=w1332:i32)  [unwired: 2 in, 1 out]
                    n467 = In Range and Coerce(upper limit=100, x=w1332, lower limit=0) -> (In Range?=w1336:bool)  [unwired: 1 out]
                    n468 = Replace Array Subset(array=w1334, new element=w1332, index=1) -> (w1331:dbl[])
                    n469 = Replace Array Subset(array=w1338, new element=w1336, index=1) -> (w1335:bool[])
                    n470 = local read "DAQmx Device Name"() -> (w1330:tag)
                    n471 = call "Operation (SubVI).vi"("On/Off"=FALSE, "Operation"=T5."Down", "DAQmx Device Name"=w1330) -> ()  [unwired: 8 in, 1 out]
                  }
                }
              }
              frame "VC=1000" {
                n472 = local read "DAQmx Device Name"() -> (w1346:tag)
                n473 = call "Operation (SubVI).vi"("error in (no error)"=w1352, "On/Off"=TRUE, "Operation"=T5."Venable", "DAQmx Device Name"=w1346) -> ("error out"=w1351:errorcluster)  [unwired: 7 in]
                n474 = call "Serial.vi"("error in (no error)"=w1351, "write buffer"="EP=1\r\nVC=0\r\n", "VISA resource name"=w1355) -> ("error out"=w1343:errorcluster)  [unwired: 7 in, 1 out]
                n475 = call "Operation (SubVI).vi"("error in (no error)"=w1343, "On/Off"=TRUE, "Operation"=T5."Up", "DAQmx Device Name"=w1346) -> ()  [unwired: 7 in, 1 out]
              }
              frame "Wait" {
                n476 = control-ref of="Motor Speed RPM Serial"() -> (w1367:refnum<vi>)
                n477 = control-ref of="Pannel User Message"() -> (w1366:refnum<vi>)
                n478 = control-ref of="Stop Button"() -> (w1361:refnum<vi>)
                n479 = call "Write panel message Kinetics (SubVI).vi"(4:"rpm"=w1367, 5:"rpm"=TRUE ("rpm"), "PrintTime"=TRUE, "Stop"=w1361, "Time to wait"=30.0, "Strin"=w1362, "String in"=w1366) -> ("Stopped"=w1357:bool)  [unwired: 3 in, 1 out]
              }
            }
          }
        }
        frame "Resistance Merkava 4 Test" {
          w1376 = T12 [enum."0 ohm", enum."6 ohm", enum."15 ohm"] items=["Init", "0 ohm", "6 ohm", "13.2 ohm", "15 ohm", "25.9 ohm", "33 ohm", "Down", "Up", "Venable", "Firmware", "PowerSuply"]
          w1380 = T12 [enum."6 ohm", enum."15 ohm", enum."15 ohm"] items=["Init", "0 ohm", "6 ohm", "13.2 ohm", "15 ohm", "25.9 ohm", "33 ohm", "Down", "Up", "Venable", "Firmware", "PowerSuply"]
          w1385 = T12 [enum."Venable", enum."Down"] items=["Init", "0 ohm", "6 ohm", "13.2 ohm", "15 ohm", "25.9 ohm", "33 ohm", "Down", "Up", "Venable", "Firmware", "PowerSuply"]
          w1386 = T12 [enum."PowerSuply", enum."Venable", enum."Down", enum."0 ohm", enum."PowerSuply"] items=["Init", "0 ohm", "6 ohm", "13.2 ohm", "15 ohm", "25.9 ohm", "33 ohm", "Down", "Up", "Venable", "Firmware", "PowerSuply"]
          w1393 = T12 [enum."0 ohm", enum."6 ohm", enum."15 ohm"] items=["Init", "0 ohm", "6 ohm", "13.2 ohm", "15 ohm", "25.9 ohm", "33 ohm", "Down", "Up", "Venable", "Firmware", "PowerSuply"]
          # "1.65"
          n480 = control-ref of="Pannel User Message"() -> (w1399:refnum<vi>)
          n481 = Concatenate Strings(w1395, " in process..." ("Strin")) -> (w1387:string)
          n482 = property class="Str"(reference=w1399, error in=w1394, "Value"=w1387) -> (error out=w1398:errorcluster)  [unwired: 1 out]
          n483 = call "Table_ScrollaBarMarvin.vi"("error in"=w1398, "Line to focus"=w1395, "reference in"=w1389) -> ()  [unwired: 3 out]
          n484 = call "Reset old test Values (SubVI) Kinetics.vi"("Atr in"=w1389, "Test Paragraph"=w1395) -> ("error out"=w1397:errorcluster)  [unwired: 7 in, 2 out]
          n485 = call "Find_Number_LineMARVIN.vi"("Test Paragraph"=w1395, "error in"=w1397, "TableIn"=w1389) -> ("error out"=w1370:errorcluster, "Line number"=w1391:i32)  [unwired: 2 in, 2 out]
          n486 = call "Cable Length Param.vi"("error constant"=w1370) -> ("error out"=w1369:errorcluster, "Cable Length Param"=w1372:string)  [unwired: 9 in]
          n487 = for {
            tunnel: w1386 -> [w1410] mode=indexing
            tunnel: [w1408] -> w1388
            tunnel: w1369 -> [w1409]
            tunnel: [w1405] -> w1368
            tunnel: bool[] [FALSE, TRUE, TRUE, TRUE, TRUE] -> [w1407] mode=indexing
            tunnel: dbl[] [5.0, 0.2, 0.2, 0.2, 3.0] -> [w1404] mode=indexing
            n488 = local read "DAQmx Device Name"() -> (w1408:tag)
            n489 = call "Operation (SubVI).vi"("error in (no error)"=w1409, "On/Off"=w1407, "Operation"=w1410, "DAQmx Device Name"=w1408) -> ("error out"=w1406:errorcluster)  [unwired: 7 in]
            n490 = call "Time Delay6"("error in (no error)"=w1406, "Delay Time (s)"=w1404) -> ("error out"=w1405:errorcluster)  [unwired: 9 in]
          }
          n491 = Concatenate Strings("EP=1\r\n" ("write buffer"), w1372, "\\r\\n" ("string")) -> (w1371:string)
          n492 = call "Serial.vi"("error in (no error)"=w1368, "write buffer"=w1371, "VISA resource name"=w1383) -> ("error out"=w1384:errorcluster)  [unwired: 7 in, 1 out]
          n493 = Increment(x=w1391) -> (x+1=w1390:i32)
          n494 = for {
            tunnel: w1393 -> [w1417] mode=indexing
            tunnel: i32[] [6850, 8300, 9200] -> [w1433] mode=indexing
            tunnel: w1390 -> [w1428]
            tunnel: w1389 -> [w1423]
            tunnel: w1384 -> [w1422]
            tunnel: w1388 -> [w1421]
            tunnel: w1387 -> [w1420]
            tunnel: bool[] [TRUE, TRUE, TRUE] -> [w1419] mode=indexing
            tunnel: w1380 -> [w1414] mode=indexing
            tunnel: [w1418] -> w1378
            tunnel: bool[] [TRUE, FALSE] -> [w1416]
            tunnel: w1376 -> [w1413] mode=indexing
            tunnel: [w1412] -> w1375
            i -> [w1429]
            stop <- w1418 stop-if-true
            w1432 = 100 ("x")
            n495 = Add(x=w1428, y=w1429) -> (x+y=w1427:i32)
            n496 = call "Operation (SubVI).vi"("error in (no error)"=w1422, "On/Off"=w1419, "Operation"=w1417, "DAQmx Device Name"=w1421) -> ("error out"=w1435:errorcluster)  [unwired: 7 in]
            n497 = control-ref of="Motor Speed RPM Serial"() -> (w1436:refnum<vi>)
            n498 = control-ref of="Pannel User Message"() -> (w1438:refnum<vi>)
            n499 = control-ref of="Stop Button"() -> (w1441:refnum<vi>)
            n500 = call "Write panel message Kinetics (SubVI).vi"(4:"rpm"=w1436, 5:"rpm"=TRUE ("rpm"), "PrintTime"=TRUE, "Stop"=w1441, "error in (no error)"=w1435, "Time to wait"=30.0, "Strin"=w1420, "String in"=w1438) -> ("error out"=w1434:errorcluster, "Stopped"=w1418:bool)  [unwired: 2 in]
            n501 = property on="Motor Speed RPM Serial" class="DigNum (strict)"(error in=w1434) -> (error out=w1426:errorcluster, "Value"=w1425:dbl)  [unwired: 1 in, 1 out]
            n502 = Subtract(x=w1433, y=w1432) -> (x-y=w1430:i32)
            n503 = Add(x=w1432, y=w1433) -> (x+y=w1431:i32)
            n504 = In Range and Coerce(upper limit=w1431, x=w1425, lower limit=w1430) -> (In Range?=w1424:bool)  [unwired: 1 out]
            n505 = call "PassOrFail (SubVI).vi"("index (row)"=w1427, "error in (no error)"=w1426, "Data in"=w1425, "Pass?Fail"=w1424, "Table in"=w1423) -> ("error out"=w1411:errorcluster)  [unwired: 6 in]
            n506 = Build Array(w1414, w1413) -> (w1415:T12)
            n507 = for {
              tunnel: w1421 -> [w1447]
              tunnel: w1416 -> [w1446] mode=indexing
              tunnel: w1415 -> [w1445] mode=indexing
              tunnel: [w1443] -> w1412
              tunnel: w1411 -> [w1442]
              n508 = call "Operation (SubVI).vi"("error in (no error)"=w1442, "On/Off"=w1446, "Operation"=w1445, "DAQmx Device Name"=w1447) -> ("error out"=w1444:errorcluster)  [unwired: 7 in]
              n509 = call "Time Delay5"("error in (no error)"=w1444) -> ("error out"=w1443:errorcluster)  [unwired: 10 in]
            }
          }
          n510 = for {
            tunnel: w1375 -> [w1401]
            tunnel: w1385 -> [w1400] mode=indexing
            n511 = local read "DAQmx Device Name"() -> (w1402:tag)
            n512 = call "Operation (SubVI).vi"("error in (no error)"=w1401, "On/Off"=FALSE, "Operation"=w1400, "DAQmx Device Name"=w1402) -> ()  [unwired: 7 in, 1 out]
          }
        }
        frame "Resistance Merkava 3 Test" {
          w1457 = T12 [enum."0 ohm", enum."13.2 ohm", enum."33 ohm"] items=["Init", "0 ohm", "6 ohm", "13.2 ohm", "15 ohm", "25.9 ohm", "33 ohm", "Down", "Up", "Venable", "Firmware", "PowerSuply"]
          w1461 = T12 [enum."13.2 ohm", enum."33 ohm", enum."33 ohm"] items=["Init", "0 ohm", "6 ohm", "13.2 ohm", "15 ohm", "25.9 ohm", "33 ohm", "Down", "Up", "Venable", "Firmware", "PowerSuply"]
          w1464 = T12 [enum."PowerSuply", enum."Venable", enum."Up", enum."0 ohm", enum."PowerSuply"] items=["Init", "0 ohm", "6 ohm", "13.2 ohm", "15 ohm", "25.9 ohm", "33 ohm", "Down", "Up", "Venable", "Firmware", "PowerSuply"]
          (unwired) "EP=1\r\nCF[0]=4.5\r\n" ("write buffer")
          w1467 = T12 [enum."Venable", enum."Up"] items=["Init", "0 ohm", "6 ohm", "13.2 ohm", "15 ohm", "25.9 ohm", "33 ohm", "Down", "Up", "Venable", "Firmware", "PowerSuply"]
          w1473 = T12 [enum."0 ohm", enum."13.2 ohm", enum."33 ohm"] items=["Init", "0 ohm", "6 ohm", "13.2 ohm", "15 ohm", "25.9 ohm", "33 ohm", "Down", "Up", "Venable", "Firmware", "PowerSuply"]
          # "6.5"
          n513 = control-ref of="Pannel User Message"() -> (w1479:refnum<vi>)
          n514 = Concatenate Strings(w1475, " in process..." ("Strin")) -> (w1448:string)
          n515 = property class="Str"(reference=w1479, error in=w1474, "Value"=w1448) -> (error out=w1478:errorcluster)  [unwired: 1 out]
          n516 = call "Table_ScrollaBarMarvin.vi"("error in"=w1478, "Line to focus"=w1475, "reference in"=w1469) -> ()  [unwired: 3 out]
          n517 = call "Reset old test Values (SubVI) Kinetics.vi"("Atr in"=w1469, "Test Paragraph"=w1475) -> ("error out"=w1477:errorcluster)  [unwired: 7 in, 2 out]
          n518 = call "Find_Number_LineMARVIN.vi"("Test Paragraph"=w1475, "error in"=w1477, "TableIn"=w1469) -> ("error out"=w1450:errorcluster, "Line number"=w1471:i32)  [unwired: 2 in, 2 out]
          n519 = call "Cable Length Param.vi"("error constant"=w1450) -> ("error out"=w1449:errorcluster, "Cable Length Param"=w1454:string)  [unwired: 9 in]
          n520 = for {
            tunnel: [w1489] -> w1468
            tunnel: w1449 -> [w1490]
            tunnel: [w1485] -> w1451
            tunnel: w1464 -> [w1488] mode=indexing
            tunnel: bool[] [FALSE, TRUE, TRUE, TRUE, TRUE] -> [w1487] mode=indexing
            tunnel: dbl[] [5.0, 0.2, 0.2, 0.2, 3.0] -> [w1484] mode=indexing
            n521 = local read "DAQmx Device Name"() -> (w1489:tag)
            n522 = call "Operation (SubVI).vi"("error in (no error)"=w1490, "On/Off"=w1487, "Operation"=w1488, "DAQmx Device Name"=w1489) -> ("error out"=w1486:errorcluster)  [unwired: 7 in]
            n523 = call "Time Delay7"("error in (no error)"=w1486, "Delay Time (s)"=w1484) -> ("error out"=w1485:errorcluster)  [unwired: 9 in]
          }
          n524 = Concatenate Strings("EP=1\r\n" ("write buffer"), w1454, "\\r\\n" ("string")) -> (w1452:string)
          n525 = Increment(x=w1471) -> (x+1=w1470:i32)
          n526 = call "Serial.vi"("error in (no error)"=w1451, "write buffer"=w1452, "VISA resource name"=w1466) -> ("error out"=w1465:errorcluster)  [unwired: 7 in, 1 out]
          n527 = for {
            tunnel: w1473 -> [w1502] mode=indexing
            tunnel: i32[] [6850, 9000, 9980] -> [w1513] mode=indexing
            tunnel: w1470 -> [w1508]
            tunnel: w1469 -> [w1503]
            tunnel: w1465 -> [w1501]
            tunnel: w1468 -> [w1500]
            tunnel: w1448 -> [w1499]
            tunnel: bool[] [FALSE, TRUE, TRUE] -> [w1498] mode=indexing
            tunnel: w1461 -> [w1495] mode=indexing
            tunnel: [w1497] -> w1459
            tunnel: bool[] [TRUE, FALSE] -> [w1496]
            tunnel: w1457 -> [w1494] mode=indexing
            tunnel: [w1492] -> w1456
            i -> [w1509]
            stop <- w1497 stop-if-true
            w1512 = 100 ("x")
            n528 = Add(x=w1508, y=w1509) -> (x+y=w1507:i32)
            n529 = call "Operation (SubVI).vi"("error in (no error)"=w1501, "On/Off"=w1498, "Operation"=w1502, "DAQmx Device Name"=w1500) -> ("error out"=w1515:errorcluster)  [unwired: 7 in]
            n530 = control-ref of="Motor Speed RPM Serial"() -> (w1516:refnum<vi>)
            n531 = control-ref of="Pannel User Message"() -> (w1518:refnum<vi>)
            n532 = control-ref of="Stop Button"() -> (w1521:refnum<vi>)
            n533 = call "Write panel message Kinetics (SubVI).vi"(4:"rpm"=w1516, 5:"rpm"=TRUE ("rpm"), "PrintTime"=TRUE, "Stop"=w1521, "error in (no error)"=w1515, "Time to wait"=30.0, "Strin"=w1499, "String in"=w1518) -> ("error out"=w1514:errorcluster, "Stopped"=w1497:bool)  [unwired: 2 in]
            n534 = property on="Motor Speed RPM Serial" class="DigNum (strict)"(error in=w1514) -> (error out=w1506:errorcluster, "Value"=w1505:dbl)  [unwired: 1 in, 1 out]
            n535 = Subtract(x=w1513, y=w1512) -> (x-y=w1510:i32)
            n536 = Add(x=w1512, y=w1513) -> (x+y=w1511:i32)
            n537 = In Range and Coerce(upper limit=w1511, x=w1505, lower limit=w1510) -> (In Range?=w1504:bool)  [unwired: 1 out]
            n538 = Build Array(w1495, w1494) -> (w1493:T12)
            n539 = call "PassOrFail (SubVI).vi"("index (row)"=w1507, "error in (no error)"=w1506, "Data in"=w1505, "Pass?Fail"=w1504, "Table in"=w1503) -> ("error out"=w1491:errorcluster)  [unwired: 6 in]
            n540 = for {
              tunnel: w1500 -> [w1527]
              tunnel: w1496 -> [w1526] mode=indexing
              tunnel: w1493 -> [w1525] mode=indexing
              tunnel: [w1523] -> w1492
              tunnel: w1491 -> [w1522]
              n541 = call "Operation (SubVI).vi"("error in (no error)"=w1522, "On/Off"=w1526, "Operation"=w1525, "DAQmx Device Name"=w1527) -> ("error out"=w1524:errorcluster)  [unwired: 7 in]
              n542 = call "Time Delay2"("error in (no error)"=w1524) -> ("error out"=w1523:errorcluster)  [unwired: 10 in]
            }
          }
          n543 = for {
            tunnel: w1456 -> [w1481]
            tunnel: w1467 -> [w1480] mode=indexing
            n544 = local read "DAQmx Device Name"() -> (w1482:tag)
            n545 = call "Operation (SubVI).vi"("error in (no error)"=w1481, "On/Off"=FALSE, "Operation"=w1480, "DAQmx Device Name"=w1482) -> ()  [unwired: 7 in, 1 out]
          }
        }
        frame "Resistance Namer Test" {
          w1536 = T12 [enum."13.2 ohm", enum."25.9 ohm", enum."33 ohm"] items=["Init", "0 ohm", "6 ohm", "13.2 ohm", "15 ohm", "25.9 ohm", "33 ohm", "Down", "Up", "Venable", "Firmware", "PowerSuply"]
          w1537 = T12 [enum."25.9 ohm", enum."33 ohm", enum."33 ohm"] items=["Init", "0 ohm", "6 ohm", "13.2 ohm", "15 ohm", "25.9 ohm", "33 ohm", "Down", "Up", "Venable", "Firmware", "PowerSuply"]
          w1543 = T12 [enum."Init", enum."PowerSuply", enum."Venable", enum."Down", enum."Up", enum."13.2 ohm", enum."PowerSuply", enum."Down", enum."Up"] items=["Init", "0 ohm", "6 ohm", "13.2 ohm", "15 ohm", "25.9 ohm", "33 ohm", "Down", "Up", "Venable", "Firmware", "PowerSuply"]
          (unwired) "EP=1\r\nCF[0]=4.5\r\n" ("write buffer")
          w1546 = T12 [enum."Init", enum."Down", enum."Up"] items=["Init", "0 ohm", "6 ohm", "13.2 ohm", "15 ohm", "25.9 ohm", "33 ohm", "Down", "Up", "Venable", "Firmware", "PowerSuply"]
          w1552 = T12 [enum."13.2 ohm", enum."25.9 ohm", enum."33 ohm"] items=["Init", "0 ohm", "6 ohm", "13.2 ohm", "15 ohm", "25.9 ohm", "33 ohm", "Down", "Up", "Venable", "Firmware", "PowerSuply"]
          n546 = control-ref of="Pannel User Message"() -> (w1558:refnum<vi>)
          n547 = Concatenate Strings(w1554, " in process..." ("Strin")) -> (w1547:string)
          n548 = property class="Str"(reference=w1558, error in=w1553, "Value"=w1547) -> (error out=w1557:errorcluster)  [unwired: 1 out]
          n549 = call "Table_ScrollaBarMarvin.vi"("error in"=w1557, "Line to focus"=w1554, "reference in"=w1548) -> ()  [unwired: 3 out]
          n550 = call "Reset old test Values (SubVI) Kinetics.vi"("Atr in"=w1548, "Test Paragraph"=w1554) -> ("error out"=w1556:errorcluster)  [unwired: 7 in, 2 out]
          n551 = call "Find_Number_LineMARVIN.vi"("Test Paragraph"=w1554, "error in"=w1556, "TableIn"=w1548) -> ("error out"=w1529:errorcluster, "Line number"=w1550:i32)  [unwired: 2 in, 2 out]
          n552 = call "Cable Length Param.vi"("error constant"=w1529) -> ("error out"=w1528:errorcluster, "Cable Length Param"=w1534:string)  [unwired: 9 in]
          n553 = for {
            tunnel: [w1568] -> w1540
            tunnel: w1528 -> [w1569]
            tunnel: [w1565] -> w1530
            tunnel: w1543 -> [w1567] mode=indexing
            tunnel: dbl[] [1.0, 5.0, 0.2, 0.2, 0.2, 0.2, 5.0, 0.2, 0.2] -> [w1564] mode=indexing
            tunnel: bool[] [FALSE, FALSE, TRUE, TRUE, TRUE, TRUE, TRUE, TRUE, TRUE] -> [w1563] mode=indexing
            n554 = local read "DAQmx Device Name"() -> (w1568:tag)
            n555 = call "Operation (SubVI).vi"("error in (no error)"=w1569, "On/Off"=w1563, "Operation"=w1567, "DAQmx Device Name"=w1568) -> ("error out"=w1566:errorcluster)  [unwired: 7 in]
            n556 = call "Time Delay10"("error in (no error)"=w1566, "Delay Time (s)"=w1564) -> ("error out"=w1565:errorcluster)  [unwired: 9 in]
          }
          n557 = Concatenate Strings("EP=1\r\n" ("write buffer"), w1534, "\\r\\n" ("string")) -> (w1531:string)
          n558 = call "Serial.vi"("error in (no error)"=w1530, "write buffer"=w1531, "VISA resource name"=w1539) -> ("error out"=w1545:errorcluster)  [unwired: 7 in, 1 out]
          n559 = Increment(x=w1550) -> (x+1=w1549:i32)
          n560 = for {
            tunnel: w1552 -> [w1576] mode=indexing
            tunnel: i32[] [8350, 8900, 9450] -> [w1591] mode=indexing
            tunnel: w1549 -> [w1586]
            tunnel: w1548 -> [w1581]
            tunnel: w1545 -> [w1580]
            tunnel: w1540 -> [w1579]
            tunnel: w1547 -> [w1578]
            tunnel: [w1577] -> w1541
            tunnel: bool[] [TRUE, FALSE] -> [w1575]
            tunnel: w1537 -> [w1574] mode=indexing
            tunnel: w1536 -> [w1573] mode=indexing
            tunnel: [w1571] -> w1535
            i -> [w1587]
            stop <- w1577 stop-if-true
            w1590 = 100 ("x")
            n561 = Add(x=w1586, y=w1587) -> (x+y=w1585:i32)
            n562 = call "Operation (SubVI).vi"("error in (no error)"=w1580, "On/Off"=TRUE, "Operation"=w1576, "DAQmx Device Name"=w1579) -> ("error out"=w1593:errorcluster)  [unwired: 7 in]
            n563 = control-ref of="Motor Speed RPM Serial"() -> (w1594:refnum<vi>)
            n564 = control-ref of="Pannel User Message"() -> (w1596:refnum<vi>)
            n565 = control-ref of="Stop Button"() -> (w1599:refnum<vi>)
            n566 = call "Write panel message Kinetics (SubVI).vi"(4:"rpm"=w1594, 5:"rpm"=TRUE ("rpm"), "PrintTime"=TRUE, "Stop"=w1599, "error in (no error)"=w1593, "Time to wait"=30.0, "Strin"=w1578, "String in"=w1596) -> ("error out"=w1592:errorcluster, "Stopped"=w1577:bool)  [unwired: 2 in]
            n567 = property on="Motor Speed RPM Serial" class="DigNum (strict)"(error in=w1592) -> (error out=w1584:errorcluster, "Value"=w1583:dbl)  [unwired: 1 in, 1 out]
            n568 = Subtract(x=w1591, y=w1590) -> (x-y=w1588:i32)
            n569 = Add(x=w1590, y=w1591) -> (x+y=w1589:i32)
            n570 = In Range and Coerce(upper limit=w1589, x=w1583, lower limit=w1588) -> (In Range?=w1582:bool)  [unwired: 1 out]
            n571 = Build Array(w1574, w1573) -> (w1572:T12)
            n572 = call "PassOrFail (SubVI).vi"("index (row)"=w1585, "error in (no error)"=w1584, "Data in"=w1583, "Pass?Fail"=w1582, "Table in"=w1581) -> ("error out"=w1570:errorcluster)  [unwired: 6 in]
            n573 = for {
              tunnel: w1579 -> [w1606]
              tunnel: w1575 -> [w1605] mode=indexing
              tunnel: w1572 -> [w1604] mode=indexing
              tunnel: [w1602] -> w1571
              tunnel: w1570 -> [w1601]
              n574 = call "Operation (SubVI).vi"("error in (no error)"=w1601, "On/Off"=w1605, "Operation"=w1604, "DAQmx Device Name"=w1606) -> ("error out"=w1603:errorcluster)  [unwired: 7 in]
              n575 = call "Time Delay13"("error in (no error)"=w1603) -> ("error out"=w1602:errorcluster)  [unwired: 10 in]
            }
          }
          n576 = for {
            tunnel: w1535 -> [w1560]
            tunnel: w1546 -> [w1559] mode=indexing
            n577 = local read "DAQmx Device Name"() -> (w1561:tag)
            n578 = call "Operation (SubVI).vi"("error in (no error)"=w1560, "On/Off"=FALSE, "Operation"=w1559, "DAQmx Device Name"=w1561) -> ()  [unwired: 7 in, 1 out]
          }
        }
        frame "Analog Voltage Test" {
          w1614 = T12 [enum."Init", enum."PowerSuply"] items=["Init", "0 ohm", "6 ohm", "13.2 ohm", "15 ohm", "25.9 ohm", "33 ohm", "Down", "Up", "Venable", "Firmware", "PowerSuply"]
          w1638 = dbl[] [0.0, 1.0, 2.0, 3.0, 4.0, 4.5]
          n579 = control-ref of="Pannel User Message"() -> (w1646:refnum<vi>)
          n580 = Concatenate Strings(w1640, " in process..." ("string")) -> (w1620:string)
          n581 = property class="Str"(reference=w1646, error in=w1642, "Value"=w1620) -> (error out=w1645:errorcluster)  [unwired: 1 out]
          n582 = call "Table_ScrollaBarMarvin.vi"("error in"=w1645, "Line to focus"=w1640, "reference in"=w1641) -> ("error out"=w1644:errorcluster)  [unwired: 2 out]
          n583 = local read "DAQmx Device Name"() -> (w1612:tag)
          n584 = call "Find_Number_LineMARVIN.vi"("Test Paragraph"=w1640, "error in"=w1644, "TableIn"=w1641) -> ("error out"=w1648:errorcluster, "Line number"=w1647:i32)  [unwired: 2 in, 2 out]
          n585 = call <vilib>:"Clear Errors.vi"("error in (no error)"=w1648) -> ("error out"=w1639:errorcluster)  [unwired: 5 in, 1 out]
          n586 = call "Reset old test Values (SubVI) Kinetics.vi"("error in"=w1639, "Atr in"=w1641, "Test Paragraph"=w1640) -> ("error out"=w1628:errorcluster)  [unwired: 6 in, 2 out]
          n587 = for {
            tunnel: w1612 -> [w1653]
            tunnel: w1614 -> [w1652] mode=indexing
            tunnel: bool[] [FALSE, TRUE] -> [w1651] mode=indexing
            shift-right: [w1650] -> w1625
            shift-left: w1628 -> [w1654]
            n588 = call "Operation (SubVI).vi"("error in (no error)"=w1654, "On/Off"=w1651, "Operation"=w1652, "DAQmx Device Name"=w1653) -> ("error out"=w1650:errorcluster)  [unwired: 7 in]
          }
          n589 = control-ref of="Pannel User Message"() -> (w1627:refnum<vi>)
          n590 = control-ref of="Motor Speed RPM Serial"() -> (w1623:refnum<vi>)
          n591 = control-ref of="Stop Button"() -> (w1621:refnum<vi>)
          n592 = call "Write panel message Kinetics (SubVI).vi"(4:"rpm"=w1623, 5:"rpm"=FALSE ("rpm"), "PrintTime"=FALSE, "Stop"=w1621, "error in (no error)"=w1625, "Time to wait"=5.0, "Strin"=w1620, "String in"=w1627) -> ("error out"=w1619:errorcluster)  [unwired: 2 in, 1 out]
          n593 = local read "DAQmx Device Name"() -> (w1631:tag)
          n594 = call "Serial.vi"("error in (no error)"=w1619, "write buffer"="EP=1\r\nVC=0\r\n", "VISA resource name"=w1618) -> ("error out"=w1616:errorcluster)  [unwired: 7 in, 1 out]
          n595 = while {
            tunnel: [w1657] -> w1613
            tunnel: [TRUE] -> w1617
            tunnel: w1616 -> [w1655]
            stop <- w1659 stop-if-true
            n596 = control-ref of="Motor Speed RPM Serial"() -> (w1661:refnum<vi>)
            n597 = property class="DigNum (strict)"(reference=w1661, error in=w1655) -> (error out=w1657:errorcluster, "Value"=w1660:dbl)  [unwired: 1 out]
            n598 = Less Or Equal?(x=w1660, y=50.0) -> (x <= y?=w1659:bool)
          }
          "Analogtest" <- w1617
          n599 = call "Operation (SubVI).vi"("error in (no error)"=w1613, "On/Off"=FALSE, "Operation"=T5."PowerSuply", "DAQmx Device Name"=w1612) -> ("error out"=w1609:errorcluster)  [unwired: 7 in]
          n600 = call "Time Delay14"("error in (no error)"=w1609, "Delay Time (s)"=20.0) -> ("error out"=w1608:errorcluster)  [unwired: 9 in]
          n601 = for {
            tunnel: w1638 -> [w1672] mode=indexing
            tunnel: w1618 -> [w1671]
            tunnel: w1641 -> [w1670]
            tunnel: w1608 -> [w1665]
            tunnel: w1647 -> [w1669]
            tunnel: w1638 -> [w1668]
            tunnel: w1620 -> [w1667]
            tunnel: [w1665] -> w1637
            shift-right: [w1664] -> _
            shift-left: T10."Init" -> [w1673]
            tunnel: [w1663] -> w1632
            tunnel: w1631 -> [w1662]
            i -> [w1666]
            n602 = while {
              shift-right: [w1679] -> w1664
              shift-left: w1673 -> [w1685]
              tunnel: w1672 -> [w1684]
              tunnel: w1671 -> [w1683]
              tunnel: w1670 -> [w1682]
              tunnel: w1669 -> [w1681]
              tunnel: w1668 -> [w1680]
              tunnel: w1667 -> [w1678]
              tunnel: w1666 -> [w1677]
              tunnel: [w1675] -> w1663
              tunnel: w1662 -> [w1674]
              stop <- w1676 stop-if-true
              n603 = case shown="\"AI0/3\"" w1685 {
                tunnel: w1684 -> [_ w1690 w1725 w1731 _ _]
                tunnel: w1683 -> [_ _ _ _ _ w1752]
                tunnel: w1682 -> [_ w1697 _ _ _ w1774]
                tunnel: w1681 -> [_ w1696 _ _ _ w1773]
                tunnel: w1680 -> [_ _ _ _ _ w1772]
                tunnel: [T10."AO0" T10."Exit" T10."Wait" T10."AI0/3" T10."Read" w1756] -> w1679
                tunnel: [TRUE _ _ w1727 TRUE _] -> w1676
                tunnel: w1678 -> [_ _ _ w1735 _ _]
                tunnel: w1677 -> [_ w1691 _ _ _ _]
                tunnel: [_ _ _ w1727 _ _] -> w1675
                tunnel: w1674 -> [_ w1689 w1724 _ _ w1759]
                frame "Exit", Default {
                }
                frame "AI0/3" {
                  n604 = Increment(x=w1696) -> (x+1=w1695:i32)
                  n605 = property on="Motor Speed RPM Serial" class="DigNum (strict)"() -> ("Value"=w1699:dbl)  [unwired: 2 in, 2 out]
                  n606 = Multiply(x=w1691, y=2) -> (x*y=w1693:i32)
                  n607 = call "Aquire AI0"("device name"=w1689) -> ("data"=w1700:dynamicdata)  [unwired: 16 in, 2 out]
                  n608 = Add(x=w1695, y=w1693) -> (x+y=w1694:i32)
                  n609 = property on="Offset" class="DigNum (strict)" props=["Value"]() -> ()  [unwired: 2 in, 3 out]
                  n610 = To Double Precision Float(number=w1700) -> (double precision float=w1688:dbl)
                  n611 = Build Array(w1688, w1699) -> (w1698:dbl[])
                  n612 = for {
                    tunnel: w1698 -> [w1702] mode=indexing
                    tunnel: w1697 -> [w1707]
                    tunnel: w1694 -> [w1709]
                    tunnel: w1691 -> [w1705]
                    tunnel: w1690 -> [w1703]
                    i -> [w1706]
                    n613 = case shown="0, Default" w1706 {
                      tunnel: w1705 -> [_ w1717]
                      tunnel: [w1711 w1720] -> w1704
                      tunnel: w1703 -> [w1713 _]
                      tunnel: w1702 -> [w1710 w1719]
                      frame 0, Default {
                        w1712 = 0.2 ("y")
                        n614 = Add(x=w1712, y=w1713) -> (x+y=w1714:dbl)
                        n615 = Subtract(x=w1713, y=w1712) -> (x-y=w1715:dbl)
                        n616 = In Range and Coerce(upper limit=w1714, x=w1710, lower limit=w1715) -> (In Range?=w1711:bool)  [unwired: 1 out]
                      }
                      frame 1 {
                        w1721 = 200.0 ("y")
                        n617 = property on="SpeedLimit" class="Arr (strict)"() -> ("Value"=w1718:dbl[])  [unwired: 2 in, 2 out]
                        n618 = Index Array(array=w1718, index=w1717) -> (element=w1716:dbl)
                        n619 = Add(x=w1721, y=w1716) -> (x+y=w1722:dbl)
                        n620 = Subtract(x=w1716, y=w1721) -> (x-y=w1723:dbl)
                        n621 = In Range and Coerce(upper limit=w1722, x=w1719, lower limit=w1723) -> (In Range?=w1720:bool)  [unwired: 1 out]
                      }
                    }
                    n622 = Add(x=w1709, y=w1706) -> (x+y=w1708:i32)
                    n623 = call "PassOrFail (SubVI).vi"("index (row)"=w1708, "Data in"=w1702, "Pass?Fail"=w1704, "Table in"=w1707) -> ()  [unwired: 7 in, 1 out]
                  }
                }
                frame "AO0" {
                  n624 = call "Generate AO0"("data"=w1725, "device name"=w1724) -> ()  [unwired: 16 in, 2 out]
                }
                frame "Wait" {
                  n625 = Number To Fractional String(number=w1731, precision (6)=i16 1) -> (F-format string=w1729:string)  [unwired: 2 in]
                  n626 = Concatenate Strings(w1735, "\r\n", "Analog Output: ", w1729, "V." ("string")) -> (w1728:string)
                  n627 = control-ref of="Pannel User Message"() -> (w1737:refnum<vi>)
                  n628 = control-ref of="Motor Speed RPM Serial"() -> (w1736:refnum<vi>)
                  n629 = control-ref of="Stop Button"() -> (w1741:refnum<vi>)
                  n630 = call "Write panel message Kinetics (SubVI).vi"(4:"rpm"=w1736, 5:"rpm"=TRUE ("rpm"), "PrintTime"=TRUE, "Stop"=w1741, "Time to wait"=20.0, "Strin"=w1728, "String in"=w1737) -> ("Stopped"=w1727:bool)  [unwired: 3 in, 1 out]
                }
                frame "Read" {
                  n631 = One Button Dialog(message="No connection.") -> ()  [unwired: 1 in, 1 out]
                }
                frame "Init" {
                  w1766 = T12 [enum."PowerSuply", enum."Venable"] items=["Init", "0 ohm", "6 ohm", "13.2 ohm", "15 ohm", "25.9 ohm", "33 ohm", "Down", "Up", "Venable", "Firmware", "PowerSuply"]
                  n632 = for {
                    tunnel: w1766 -> [w1781] mode=indexing
                    tunnel: bool[] [TRUE, TRUE] -> [w1780] mode=indexing
                    tunnel: [w1779] -> w1746
                    tunnel: dbl[] [10.0, 2.0] -> [w1777] mode=indexing
                    tunnel: w1759 -> [w1776]
                    n633 = call "Operation (SubVI).vi"("On/Off"=w1780, "Operation"=w1781, "DAQmx Device Name"=w1776) -> ("error out"=w1778:errorcluster)  [unwired: 8 in]
                    n634 = call "Time Delay11"("error in (no error)"=w1778, "Delay Time (s)"=w1777) -> ("error out"=w1779:errorcluster)  [unwired: 9 in]
                  }
                  n635 = call "Aquire AI4"("error in"=w1746, "device name"=w1759) -> ("data"=w1760:dynamicdata, "error out"=w1748:errorcluster)  [unwired: 15 in, 1 out]
                  n636 = call "Serial.vi"("error in (no error)"=w1748, "write buffer"="AG[1]\r\n", "VISA resource name"=w1752) -> ("error out"=w1747:errorcluster, "read buffer"=w1751:string)  [unwired: 7 in]
                  n637 = Fract/Exp String To Number(string=w1751, default (0 dbl)=0.0 ("default (0 DBL)")) -> (number=w1749:dbl)  [unwired: 2 in, 1 out]
                  n638 = Equal To 0?(x=w1749) -> (x = 0?=w1758:bool)
                  n639 = for {
                    tunnel: w1752 -> [w1786]
                    tunnel: [w1782] -> w1768
                    tunnel: string[] ["EP=1\r\n", "VC=0\r\n", "CS[0]=0\r\n", "AG[1]\r\n"] -> [w1785] mode=indexing
                    tunnel: w1747 -> [w1783]
                    n640 = call "Time Delay3"("error in (no error)"=w1783) -> ("error out"=w1784:errorcluster)  [unwired: 10 in]
                    n641 = call "Serial.vi"("error in (no error)"=w1784, "write buffer"=w1785, "VISA resource name"=w1786) -> ("read buffer"=w1782:string)  [unwired: 7 in, 1 out]
                  }
                  n642 = Select(t=T10."Read", s=w1758, f=T10."AO0") -> (s? t:f=w1756:T10)
                  n643 = Fract/Exp String To Number(string=w1768, default (0 dbl)=sgl 0.0 ("default (0 DBL)")) -> (number=w1754:sgl)  [unwired: 2 in, 1 out]
                  n644 = To Double Precision Float(number=w1760) -> (double precision float=→"Offset":dbl)
                  n645 = Add(x=w1773, y=2) -> (x+y=w1771:i32)
                  n646 = for {
                    tunnel: w1774 -> [w1798]
                    tunnel: w1771 -> [w1797]
                    tunnel: w1772 -> [w1793] mode=indexing
                    tunnel: w1754 -> [w1794]
                    tunnel: [w1791] -> w1763
                    tunnel: [w1787] -> w1769 mode=indexing
                    i -> [w1789]
                    n647 = Multiply(x=w1789, y=2) -> (x*y=w1790:i32)
                    n648 = Multiply(x=w1794, y=w1793) -> (x*y=w1787:dbl)
                    n649 = Add(x=w1797, y=w1790) -> (x+y=w1796:i32)
                    n650 = Number To Fractional String(number=w1787, precision (6)=i16 1) -> (F-format string=w1792:string)  [unwired: 2 in]
                    n651 = call "InsertSingleData.vi"("String In"=w1792, "Col"=2, "Row"=w1796, "Table in"=w1798) -> ("error out"=w1791:errorcluster)  [unwired: 7 in]
                  }
                  "SpeedLimit" <- w1769
                  n652 = property on="Analogtest" class="Bool (strict)"(error in=w1763, "Value"=FALSE ("Analogtest")) -> ()  [unwired: 1 in, 2 out]
                }
              }
            }
          }
          n653 = local read "DAQmx Device Name"() -> (w1630:tag)
          n654 = call "Generate AO"("data"=0.0, "error in"=w1637, "device name"=w1630) -> ("error out"=w1633:errorcluster)  [unwired: 15 in, 1 out]
          n655 = call "Operation (SubVI).vi"("error in (no error)"=w1633, "On/Off"=FALSE, "Operation"=T5."Venable", "DAQmx Device Name"=w1630) -> ()  [unwired: 7 in, 1 out]
        }
        frame "Motor Run Test" {
          n656 = control-ref of="Pannel User Message"() -> (w1819:refnum<vi>)
          n657 = Concatenate Strings(w1801, " in process..." ("Strin")) -> (w1806:string)
          n658 = property class="Str"(reference=w1819, error in=w1816, "Value"=w1806) -> (error out=w1818:errorcluster)  [unwired: 1 out]
          n659 = call "Table_ScrollaBarMarvin.vi"("error in"=w1818, "Line to focus"=w1801, "reference in"=w1809) -> ()  [unwired: 3 out]
          n660 = call "Reset old test Values (SubVI) Kinetics.vi"("Atr in"=w1809, "Test Paragraph"=w1801) -> ("error out"=w1817:errorcluster)  [unwired: 7 in, 2 out]
          n661 = call "Find_Number_LineMARVIN.vi"("Test Paragraph"=w1801, "error in"=w1817, "TableIn"=w1809) -> ("error out"=w1814:errorcluster, "Line number"=w1808:i32)  [unwired: 2 in, 2 out]
          n662 = Increment(x=w1808) -> (x+1=w1807:i32)
          n663 = while {
            tunnel: w1814 -> [w1822]
            tunnel: w1802 -> [w1829]
            shift-right: [w1827] -> _
            shift-left: T11."Init" -> [w1828]
            tunnel: w1809 -> [w1826]
            tunnel: w1807 -> [w1825]
            tunnel: w1806 -> [w1823]
            tunnel: [w1822] -> w1803
            tunnel: [w1820] -> w1800
            i -> [w1824]
            stop <- w1821 stop-if-true
            n664 = case shown="\"ReadCurrent\"" w1828 {
              tunnel: w1822 -> [_ w1835 w1847 w1891 w1906]
              tunnel: w1829 -> [_ _ _ w1892 w1904]
              tunnel: [T11."Exit" T11."ReadTemp" w1844 T11."ReadCurrent" T11."ReadTemp"] -> w1827
              tunnel: w1826 -> [_ _ w1859 w1886 _]
              tunnel: w1825 -> [_ _ w1861 w1888 _]
              tunnel: w1824 -> [_ _ w1862 w1889 _]
              tunnel: w1823 -> [_ w1836 w1846 _ _]
              tunnel: [TRUE ("Stopped") w1832 w1845 _ _] -> w1821
              tunnel: [_ w1832 _ _ _] -> w1820
              frame "Exit", Default {
              }
              frame "Wait" {
                n665 = control-ref of="Motor Speed RPM Serial"() -> (w1841:refnum<vi>)
                n666 = control-ref of="Pannel User Message"() -> (w1840:refnum<vi>)
                n667 = control-ref of="Stop Button"() -> (w1839:refnum<vi>)
                n668 = call "Write panel message Kinetics (SubVI).vi"(4:"rpm"=w1841, 5:"rpm"=TRUE ("rpm"), "PrintTime"=TRUE, "Stop"=w1839, "error in (no error)"=w1835, "Time to wait"=1140.0, "Strin"=w1836, "String in"=w1840) -> ("Stopped"=w1832:bool)  [unwired: 2 in, 1 out]
              }
              frame "ReadCurrent" {
                w1857 = 3.0 ("x")
                n669 = control-ref of="Motor Speed RPM Serial"() -> (w1853:refnum<vi>)
                n670 = control-ref of="Pannel User Message"() -> (w1852:refnum<vi>)
                n671 = control-ref of="Stop Button"() -> (w1851:refnum<vi>)
                n672 = call "Write panel message Kinetics (SubVI).vi"(4:"rpm"=w1853, 5:"rpm"=TRUE ("rpm"), "PrintTime"=TRUE, "Stop"=w1851, "error in (no error)"=w1847, "Time to wait"=59.0, "Strin"=w1846, "String in"=w1852) -> ("error out"=w1842:errorcluster, "Stopped"=w1845:bool)  [unwired: 2 in]
                n673 = disable-structure shown="Disabled" {
                  disable-tunnel: w1842 -> [w1864 _]
                  frame Disabled {
                    n674 = property on="UUT" class="Str"() -> ("Value"=w1863:string)  [unwired: 2 in, 2 out]
                    n675 = case shown="\"Condenser India\", \"Condenser Merkava\"" w1863 {
                      tunnel: [w1865 w1867] -> _
                      tunnel: w1864 -> [_ w1868]
                      frame "Condenser India", "Condenser Merkava" {
                        n676 = call "Current prob"() -> ("Current"=w1865:dbl)  [unwired: 17 in, 2 out]
                      }
                      frame "True", Default {
                        n677 = local read "DAQmx Device Name"() -> (w1871:tag)
                        n678 = call "Aquire AI3"("error in"=w1868, "device name"=w1871) -> ("data"=w1870:dynamicdata)  [unwired: 15 in, 2 out]
                        n679 = To Double Precision Float(number=w1870) -> (double precision float=w1869:dbl)
                        n680 = Multiply(x=w1869, y=25.0) -> (x*y=w1867:dbl)
                      }
                    }
                  }
                  frame Enabled {
                  }
                }
                n681 = case shown="2, Default" w1862 {
                  tunnel: w1861 -> [w1874 w1877]
                  tunnel: [w1873 w1878] -> w1860
                  tunnel: [T11."Wait" T11."Exit"] -> w1844
                  frame 2, Default {
                    n682 = Increment(x=w1874) -> (x+1=w1873:i32)
                  }
                  frame 5 {
                    n683 = Add(x=w1877, y=3) -> (x+y=w1878:i32)
                  }
                }
                n684 = call "ValFromATR(SubVI).vi"("Row"=w1860, "Table in"=w1859) -> ("Val"=w1858:dbl)  [unwired: 8 in, 1 out]
                n685 = Add(x=w1857, y=w1858) -> (x+y=w1856:dbl)
                n686 = Subtract(x=w1858, y=w1857) -> (x-y=w1855:dbl)
                n687 = call "Current prob2"("error in (no error)"=w1842) -> ("Current"=w1843:dbl)  [unwired: 16 in, 2 out]
                n688 = In Range and Coerce(upper limit=w1856, x=w1843, lower limit=w1855) -> (In Range?=w1854:bool)  [unwired: 1 out]
                n689 = call "PassOrFail (SubVI).vi"("index (row)"=w1860, "Data in"=w1843, "Pass?Fail"=w1854, "Table in"=w1859) -> ()  [unwired: 7 in, 1 out]
              }
              frame "ReadTemp" {
                w1884 = 15.0 ("x")
                n690 = case shown="4" w1889 {
                  tunnel: w1888 -> [w1894 w1896]
                  tunnel: [w1894 w1897] -> w1887
                  frame 1, Default {
                  }
                  frame 4 {
                    n691 = Add(x=w1896, y=2) -> (x+y=w1897:i32)
                  }
                }
                n692 = call "Serial.vi"("error in (no error)"=w1891, "write buffer"="TA[1]\r\n", "VISA resource name"=w1892) -> ("read buffer"=w1890:string)  [unwired: 7 in, 1 out]
                n693 = call "ValFromATR(SubVI).vi"("Row"=w1887, "Table in"=w1886) -> ("Val"=w1885:dbl)  [unwired: 8 in, 1 out]
                n694 = Fract/Exp String To Number(string=w1890) -> (number=w1880:dbl)  [unwired: 3 in, 1 out]
                n695 = Add(x=w1884, y=w1885) -> (x+y=w1883:dbl)
                n696 = Subtract(x=w1885, y=w1884) -> (x-y=w1882:dbl)
                n697 = In Range and Coerce(upper limit=w1883, x=w1880, lower limit=w1882) -> (In Range?=w1881:bool)  [unwired: 1 out]
                n698 = call "PassOrFail (SubVI).vi"("index (row)"=w1887, "Data in"=w1880, "Pass?Fail"=w1881, "Table in"=w1886) -> ()  [unwired: 7 in, 1 out]
              }
              frame "Init" {
                n699 = property on="UUT" class="Str"(error in=w1906) -> (error out=w1903:errorcluster, "Value"=w1907:string)  [unwired: 1 in, 1 out]
                n700 = case shown="\"BLDC 60A\"" w1907 {
                  tunnel: ["EP=1\r\nVC=3700\r\n" ("write buffer") "EP=1\r\nVC=9980\r\n" ("write buffer") "EP=1\r\nCL[0]=55\r\nVC=11300\r\n" ("write buffer") "EP=1\r\n" ("write buffer")] -> w1905
                  frame "BLDC 30A", Default {
                  }
                  frame "BLDC 60A" {
                  }
                  frame "Warrior 60A" {
                  }
                  frame "Condenser India", "Condenser Merkava" {
                  }
                }
                n701 = call "Serial.vi"("error in (no error)"=w1903, "write buffer"=w1905, "VISA resource name"=w1904) -> ("error out"=w1898:errorcluster)  [unwired: 7 in, 1 out]
                n702 = local read "DAQmx Device Name"() -> (w1901:tag)
                n703 = call "Operation (SubVI).vi"("error in (no error)"=w1898, "On/Off"=TRUE, "Operation"=T5."Venable", "DAQmx Device Name"=w1901) -> ()  [unwired: 7 in, 1 out]
              }
            }
          }
          n704 = call "Serial.vi"("error in (no error)"=w1803, "write buffer"="EP=1\r\nVC=0\r\n", "VISA resource name"=w1802) -> ("error out"=w1804:errorcluster)  [unwired: 7 in, 1 out]
          n705 = local read "DAQmx Device Name"() -> (w1810:tag)
          n706 = call "Operation (SubVI).vi"("error in (no error)"=w1804, "On/Off"=FALSE, "Operation"=T5."Venable", "DAQmx Device Name"=w1810) -> ()  [unwired: 7 in, 1 out]
        }
        frame "Set Production Parameters" {
          n707 = control-ref of="Pannel User Message"() -> (w1926:refnum<vi>)
          n708 = Concatenate Strings(w1919, " in process..." ("Strin")) -> (w1923:string)
          n709 = property class="Str"(reference=w1926, error in=w1921, "Value"=w1923) -> (error out=w1925:errorcluster)  [unwired: 1 out]
          n710 = call "Table_ScrollaBarMarvin.vi"("error in"=w1925, "Line to focus"=w1919, "reference in"=w1917) -> ("error out"=w1920:errorcluster)  [unwired: 2 out]
          n711 = call "Reset old test Values (SubVI) Kinetics.vi"("error in"=w1920, "Atr in"=w1917, "Test Paragraph"=w1919) -> ("error out"=w1924:errorcluster)  [unwired: 6 in, 2 out]
          n712 = call "Find_Number_LineMARVIN.vi"("Test Paragraph"=w1919, "error in"=w1924, "TableIn"=w1917) -> ("error out"=w1916:errorcluster, "Line number"=w1914:i32)  [unwired: 2 in, 2 out]
          n713 = Increment(x=w1914) -> (x+1=w1913:i32)
          n714 = for {
            tunnel: w1918 -> [w1935]
            tunnel: w1917 -> [w1934]
            tunnel: w1916 -> [w1933]
            tunnel: string[] ["SN\r\n", "PN\r\n"] -> [w1931] mode=indexing
            tunnel: w1913 -> [w1928]
            i -> [w1929]
            n715 = call "Serial.vi"("error in (no error)"=w1933, "write buffer"=w1931, "VISA resource name"=w1935) -> ("error out"=w1932:errorcluster, "read buffer"=w1930:string)  [unwired: 7 in]
            n716 = Add(x=w1928, y=w1929) -> (x+y=w1927:i32)
            n717 = case shown="0, Default" w1929 {
              tunnel: w1934 -> [w1944 w1951]
              tunnel: w1932 -> [w1943 w1950]
              tunnel: w1930 -> [w1936 w1946]
              tunnel: w1927 -> [w1937 w1945]
              frame 0, Default {
                n718 = property on="Next SN" class="DigNum (strict)"() -> ("Value"=w1941:i32)  [unwired: 2 in, 2 out]
                n719 = Decrement(x=w1941) -> (x-1=w1942:i32)
                n720 = Number To Decimal String(number=w1942) -> (decimal integer string=w1940:string)  [unwired: 1 in]
                n721 = Equal?(x=w1936, y=w1940) -> (x = y?=w1939:bool)
                n722 = call "PassOrFail (SubVI).vi"("String Res"=w1936, "index (row)"=w1937, "error in (no error)"=w1943, "Data in"=-3.0, "Pass?Fail"=w1939, "Table in"=w1944) -> ()  [unwired: 5 in, 1 out]
              }
              frame 1 {
                n723 = property on="PN" class="Str"() -> ("Value"=w1949:string)  [unwired: 2 in, 2 out]
                n724 = Equal?(x=w1949, y=w1946) -> (x = y?=w1948:bool)
                n725 = call "PassOrFail (SubVI).vi"("String Res"=w1946, "index (row)"=w1945, "error in (no error)"=w1950, "Data in"=-3.0, "Pass?Fail"=w1948, "Table in"=w1951) -> ()  [unwired: 5 in, 1 out]
              }
            }
          }
        }
      }
      "TestinExecution" <- w235
    }
    n726 = flat-sequence {
      tunnel: w219 -> [_]
      frame #0 {
        w229 = T13."Enabled" ("Disabled")
        w230 = FALSE ("Start")
        n727 = local read "DAQmx Device Name"() -> (w228:tag)
        n728 = property on="Start" class="Bool (strict)"("Value"=w230, "DisabledEnum"=w229) -> ()  [unwired: 2 in, 2 out]
        n729 = property on="Report" class="Bool (strict)"("Value"=w230, "DisabledEnum"=w229) -> ()  [unwired: 2 in, 2 out]
        n730 = call "Operation (SubVI).vi"("On/Off"=FALSE, "Operation"=T5."PowerSuply", "DAQmx Device Name"=w228) -> ()  [unwired: 8 in, 1 out]
      }
    }
  }
  n731 = while {
    shift-right: [w1956] -> _
    shift-left: T3."Initialize" -> [w1975]
    shift-right: [w1972] -> _
    shift-left: _ -> [w1971]
    shift-right: [w1970] -> _
    shift-left: w28 -> [w1968]
    shift-right: [w1969] -> _
    shift-left: refnum<vi> refnum ("Config_CANAT") -> [w1967]
    shift-right: [w1965] -> _
    shift-left: w25 -> [w1966]
    tunnel: "ATR" -> [_]
    tunnel: w19 -> [w1964]
    tunnel: w18 -> [w1963]
    shift-right: [w1961] -> _
    shift-left: w2 -> [w1962]
    tunnel: w9 -> [w1960]
    tunnel: w3 -> [w1959]
    tunnel: w17 -> [_]
    tunnel: w26 -> [w1974]
    tunnel: [w1973] -> _
    tunnel: w10 -> [_]
    tunnel: w7 -> [w1957]
    shift-right: [w1954] -> _
    shift-left: w2 -> [w1955]
    shift-right: [w1952] -> _
    shift-left: w2 -> [w1953]
    stop <- w1958 stop-if-true
    n732 = case shown="\"Stop\"" w1975 {
      tunnel: [T3."MainProgram" w2155 w2223 w2732] -> w1956
      tunnel: [FALSE w2143 FALSE FALSE] -> w1958
      tunnel: [w2015 w2148 w2217 w2730] -> w1973
      tunnel: w1974 -> [_ w2120 w2221 _]
      tunnel: [w1979 refnum<visa-resource-name> refnum ("VISA resource name") w2218 w2729] -> w1972
      tunnel: w1971 -> [_ w2167 w2219 _]
      tunnel: [w2033 w2137 w2213 w2751] -> w1970
      tunnel: [w2018 refnum<vi> refnum ("Config_CANAT") w2214 w2741] -> w1969
      tunnel: w1968 -> [w2033 w2169 w2216 w2751]
      tunnel: w1967 -> [_ w2158 w2215 w2741]
      tunnel: w1966 -> [w2032 w2162 w2212 w2750]
      tunnel: [w2032 w2136 w2211 w2750] -> w1965
      tunnel: w1964 -> [_ _ w2210 _]
      tunnel: w1963 -> [_ _ w2209 _]
      tunnel: w1962 -> [w2030 w2160 w2208 w2748]
      tunnel: [w2030 w2160 w2207 w2748] -> w1961
      tunnel: w1960 -> [w2029 _ w2206 _]
      tunnel: w1959 -> [_ _ w2205 _]
      tunnel: w1957 -> [_ _ w2204 _]
      tunnel: w1955 -> [_ _ w2203 _]
      tunnel: [w2026 w2135 w2202 w2743] -> w1954
      tunnel: w1953 -> [_ _ w2201 _]
      tunnel: [w2026 w2135 w2200 w2743] -> w1952
      frame "Erase ATR Table", Default {
        w2017 = refnum<visa-resource-name> "COMx" ("VISA Kinetics")
        w2026 = 0
        w2028 = T13."Enabled" ("Disabled")
        w2035 = FALSE ("Visible")
        n733 = property on="Serial Com" class="Bool"(error in=errorcluster {"status"=FALSE, "code"=0, "source"=""} ("error out"), "Visible"=FALSE) -> (error out=w2031:errorcluster)  [unwired: 1 in, 1 out]
        n734 = property on="VISA Kinetics" class="VISAName"(error in=w2031, "Visible"=w2035, "Value"=w2017) -> (error out=w2037:errorcluster)  [unwired: 1 in, 1 out]
        n735 = property on="Serial Status" class="Bool (strict)"(error in=w2037, "Value"=w2035) -> (error out=w2024:errorcluster)  [unwired: 1 in, 1 out]
        n736 = property on="Pannel User Message" class="Str"(error in=w2024, "Value"="Select a UUT from list bellow:") -> (error out=w2023:errorcluster)  [unwired: 1 in, 1 out]
        n737 = call "UUT select.vi"("error constant"=w2023) -> ("error constant 2"=w2003:errorcluster, 2:"UUT Out"=w1978:string, 3:"UUT Out"=w2022:u16)  [unwired: 8 in]
        "UUT" <- w1978
        n738 = property on="Pannel User Message" class="Str"(error in=w2003, "Value"="Tester initialization in process..." ("Pannel User Message")) -> (error out=w2002:errorcluster)  [unwired: 1 in, 1 out]
        n739 = call "ATRBuild.vi"("error constant"=w2002, "UUT In"=w2022) -> ("error constant 2"=w2021:errorcluster, "TestArray"=→"TestArray":string[], "TestArray Out"=w2020:string[][])  [unwired: 7 in]
        n740 = for {
          tunnel: w2020 -> [w2104] mode=indexing
          tunnel: w2021 -> [w2102]
          tunnel: [w2101] -> w2027
          tunnel: w2020 -> [w2100]
          i -> [w2103]
          n741 = for {
            tunnel: w2104 -> [_] mode=indexing
            tunnel: w2103 -> [w2110]
            tunnel: w2102 -> [w2107]
            tunnel: [w2106] -> w2101
            tunnel: w2100 -> [w2105]
            i -> [w2111]
            n742 = Bundle By Name(cluster=T14 {"Row"=0, "Column"=0} ("Active Cell:Active Cell"), "Row"=w2110, "Column"=w2111) -> (w2109:T14)
            n743 = control-ref of="ATR"() -> (w2108:refnum<vi>)
            n744 = property class="Tbl (strict)"(reference=w2108, error in=w2107, "Active Cell"=w2109, "Cell BG Color"=u32 16777226, "Value"=w2105) -> (error out=w2106:errorcluster)  [unwired: 1 out]
          }
        }
        n745 = call "DataFrom_ini (SubVI).vi"("error in (no error)"=w2027, "UUT"=w1978, "appended path"=w2029) -> ("error out"=w1984:errorcluster, "FileName"=w2012:string, "Next SN"=w1994:i32, "UUT SoftwareVer"=w1993:string, "ParamVersion"=→"ParamVersion":string, "PN"=w1991:string)  [unwired: 3 in]
        "UUT SoftwareVer" <- w1993
        "Next SN" <- w1994
        "FileName" <- w2012
        "PN" <- w1991
        n746 = Decrement(x=w1994) -> (x-1=w1995:i32)
        n747 = Number To Decimal String(number=w1995) -> (decimal integer string=w1992:string)  [unwired: 1 in]
        n748 = control-ref of="ATR"() -> (w2008:refnum<vi>)
        n749 = Build Array(w1993, w1993, w1992, w1991) -> (w1990:string[])
        n750 = call "Boards S/N"("error in (no error)"=w1984) -> ("POWER Board S/N"=→"POWER Board S/N":string, "DSP Board S/N"=→"DSP Board S/N":string, "error out"=w1983:errorcluster)  [unwired: 15 in, 1 out]
        n751 = for {
          tunnel: w1983 -> [w2052]
          tunnel: w2008 -> [w2050]
          tunnel: string[] ["RS232 Comm. + Version", "CAN Comm.", "Unit Serial number", "Unit Part number"] -> [w2049] mode=indexing
          tunnel: [w2048] -> w2010
          tunnel: [w2047] -> w1989 mode=indexing
          tunnel: w1990 -> [w2046] mode=indexing
          n752 = call "Find_Number_LineMARVIN.vi"("Test Paragraph"=w2049, "error in"=w2052, "TableIn"=w2050) -> ("error out"=w2051:errorcluster, "Line number"=w2047:i32)  [unwired: 2 in, 2 out]
          n753 = call "InsertSingleData.vi"("String In"=w2046, "error in (no error)"=w2051, "Col"=2, "Row"=w2047, "Table in"=w2050) -> ("error out"=w2048:errorcluster)  [unwired: 6 in]
        }
        n754 = control-ref of="This VI"() -> (w2006:refnum<vi>)
        n755 = Index Array(array=w1989, index=1) -> (element=w1987:i32)
        n756 = call "COM UUT Board.vi"("error in (no error)"=w2010, "VI reference (current VI)"=w2006, "VISA resource name 2"=w2017) -> ("error out"=w2014:errorcluster, ".not. x?"=w2000:bool, "VISA resource name out"=w2013:refnum<visa-resource-name>)  [unwired: 6 in]
        "Serial Status" <- w2000
        n757 = case shown="True" w2000 {
          tunnel: w2014 -> [w2054 w2077]
          tunnel: w2013 -> [w2055 w2076]
          tunnel: [w2055 w2067] -> w1979
          tunnel: [w2054 w2061] -> w1981
          tunnel: w2012 -> [_ w2060]
          tunnel: w1993 -> [_ w2056]
          frame False {
          }
          frame True {
            n758 = VISA Flush I/O Buffer(VISA resource name=w2076, error in (no error)=w2077) -> (VISA resource name out=w2067:refnum<visa-resource-name>, error out=w2075:errorcluster)  [unwired: 1 in]
            n759 = call "Display Message to User2"("error in (no error)"=w2075) -> ("error out"=w2074:errorcluster, "Yes"=w2073:bool)  [unwired: 9 in]
            n760 = case shown="True" w2073 {
              tunnel: w2074 -> [w2078 w2099]
              tunnel: [w2078 w2079] -> w2072
              tunnel: w2067 -> [_ w2097]
              tunnel: w2060 -> [_ w2090]
              frame False {
              }
              frame True {
                w2083 = u16 11 items=["Init", "0 ohm", "6 ohm", "13.2 ohm", "15 ohm", "25.9 ohm", "33 ohm", "Down", "Up", "Venable", "Firmware", "PowerSuply"] ("Operation")
                w2088 = u16 11 items=["Init", "0 ohm", "6 ohm", "13.2 ohm", "15 ohm", "25.9 ohm", "33 ohm", "Down", "Up", "Venable", "Firmware", "PowerSuply"] ("Operation")
                n761 = local read "DAQmx Device Name"() -> (w2081:tag)
                n762 = call "SetParam.vi"("RS"=TRUE, "error in (no error)"=w2099, "Visa"=w2097, "Filein"=w2090) -> ("error out"=w2086:errorcluster)  [unwired: 7 in]
                n763 = call "Operation (SubVI).vi"("error in (no error)"=w2086, "On/Off"=FALSE, "Operation"=w2088, "DAQmx Device Name"=w2081) -> ("error out"=w2085:errorcluster)  [unwired: 7 in]
                n764 = control-ref of="Pannel User Message"() -> (w2096:refnum<vi>)
                n765 = control-ref of="Motor Speed RPM Serial"() -> (w2094:refnum<vi>)
                n766 = control-ref of="Stop Button"() -> (w2095:refnum<vi>)
                n767 = call "Write panel message Kinetics (SubVI).vi"(4:"rpm"=w2094, 5:"rpm"=FALSE ("rpm"), "PrintTime"=TRUE, "Stop"=w2095, "error in (no error)"=w2085, "Time to wait"=20.0, "Strin"="Restart the UUT\nPlease wait...", "String in"=w2096) -> ("error out"=w2082:errorcluster)  [unwired: 2 in, 1 out]
                n768 = call "Operation (SubVI).vi"("error in (no error)"=w2082, "On/Off"=TRUE, "Operation"=w2083, "DAQmx Device Name"=w2081) -> ("error out"=w2080:errorcluster)  [unwired: 7 in]
                n769 = call "Time Delay12"("error in (no error)"=w2080) -> ("error out"=w2079:errorcluster)  [unwired: 10 in]
              }
            }
            n770 = call "Serial.vi"("error in (no error)"=w2072, "write buffer"="SN\r\n", "VISA resource name"=w2067) -> ("error out"=w2068:errorcluster, "read buffer"=w2062:string)  [unwired: 7 in]
            n771 = property on="UUT SN Report" class="Str"("Value"=w2062) -> ()  [unwired: 2 in, 2 out]
            n772 = Decimal String To Number(string=w2062) -> (number=→"Current SN":i32)  [unwired: 2 in, 1 out]
            n773 = call "Serial.vi"("error in (no error)"=w2068, "write buffer"="VR\r\n", "VISA resource name"=w2067) -> ("error out"=w2063:errorcluster, "read buffer"=w2057:string)  [unwired: 7 in]
            n774 = control-ref of="ATR"() -> (w2064:refnum<vi>)
            n775 = call "Find_Number_LineMARVIN.vi"("Test Paragraph"="RS232 Comm. + Version", "TableIn"=w2064) -> ("Line number"=w2065:i32)  [unwired: 3 in, 3 out]
            n776 = Equal?(x=w2057, y=w2056) -> (x = y?=w2058:bool)
            n777 = call "PassOrFail (SubVI).vi"("String Res"=w2057, "index (row)"=w2065, "error in (no error)"=w2063, "Data in"=-3.0, "Pass?Fail"=w2058, "Table in"=w2064) -> ("error out"=w2061:errorcluster)  [unwired: 5 in]
          }
        }
        n778 = case shown="\"Condenser India\", \"Condenser Merkava\"" w1978 {
          tunnel: w1981 -> [w2041 w2044]
          tunnel: [w2041 w2043] -> w1980
          tunnel: w1979 -> [_ w2042]
          frame "False", Default {
          }
          frame "Condenser India", "Condenser Merkava" {
            n779 = call "Serial.vi"("error in (no error)"=w2044, "write buffer"="EP=1\r\nVC=1000\r\n", "VISA resource name"=w2042) -> ("error out"=w2043:errorcluster)  [unwired: 7 in, 1 out]
          }
        }
        n780 = call "KineticsCan.vi"("error in"=w1980) -> ("error out"=w2009:errorcluster, "Version"=w2004:string, "Res_Pass_T"=w1977:bool, "Config_CANAT_out"=w2018:refnum<vi>)  [unwired: 7 in]
        n781 = case shown="\"Condenser India\", \"Condenser Merkava\"" w1978 {
          tunnel: w1977 -> [w2039 _]
          tunnel: [w2039 TRUE ("Res_Pass_T")] -> w1976
          frame "False", Default {
          }
          frame "Condenser India", "Condenser Merkava" {
          }
        }
        "CAN Status" <- w1976
        n782 = Equal?(x=w2004, y=w1993) -> (x = y?=w2005:bool)
        n783 = call "PassOrFail (SubVI).vi"("String Res"=w2004, "index (row)"=w1987, "error in (no error)"=w2009, "Data in"=-3.0, "Pass?Fail"=w2005, "Table in"=w2008) -> ("error out"=w1999:errorcluster)  [unwired: 5 in]
        n784 = property on="Pannel User Message" class="Str"(error in=w1999, "Value"="You can press start to execute(s) test(s)." ("Pannel User Message")) -> (error out=w1998:errorcluster)  [unwired: 1 in, 1 out]
        n785 = property on="Start" class="Bool (strict)"(error in=w1998, "DisabledEnum"=w2028) -> (error out=w2016:errorcluster)  [unwired: 1 in, 1 out]
        n786 = property on="Report" class="Bool (strict)"(error in=w2016, "DisabledEnum"=w2028) -> (error out=w2015:errorcluster)  [unwired: 1 in, 1 out]
      }
      frame "Stop" {
        w2135 = 0
        n787 = control-ref of="ATR"() -> (w2134:refnum<vi>)
        n788 = call "PassFailUUT (SubVI).vi"("error in (no error)"=w2120, "Table in"=w2134) -> ("PassFaileUUTresult"=w2127:bool)  [unwired: 7 in, 2 out]
        n789 = property on="Test Failed" class="Bool (strict)"("Value"=w2127) -> ()  [unwired: 2 in, 2 out]
        n790 = flat-sequence {
          tunnel: w2120 -> [w2197]
          tunnel: [w2196] -> w2159
          frame #0 {
            n791 = control-ref of="Pannel User Message"() -> (w2199:refnum<vi>)
            n792 = property class="Str"(reference=w2199, error in=w2197, "Value"="Program Stopped...\r\nPlease turn OFF All Power sinks") -> (error out=w2196:errorcluster)  [unwired: 1 out]
          }
        }
        n793 = Select(t="PASS" ("name or relative path"), s=w2127, f="FAIL" ("name or relative path")) -> (s? t:f=w2126:string)
        n794 = call <vilib>:"Application Directory.vi"() -> ("Application Directory"=w2130:path)
        n795 = Build Path(base path=w2130, name or relative path="data\\TestResult.ini") -> (appended path=w2133:path)
        n796 = call <vilib>:"Open Config Data.vi"("configuration file path"=w2133) -> ("error out"=w2131:errorcluster, "refnum"=w2132:T4)  [unwired: 2 in, 7 out]
        n797 = call-poly <vilib>:"Write Key.vi"("section"="Kinetics", "error in (no error)"=w2131, "value"=w2126, "key"="Result", "refnum"=w2132) -> ("error out"=w2129:errorcluster, "refnum out"=w2128:T4)  [unwired: 4 in, 1 out]
        n798 = call <vilib>:"Close Config Data.vi"("error in (no error)"=w2129, "refnum"=w2128) -> ()  [unwired: 8 in, 2 out]
        n799 = disable-structure shown="Enabled" {
          disable-tunnel: w2159 -> [w2184 w2185]
          disable-tunnel: w2158 -> [w2182 _]
          disable-tunnel: [w2181 w2185] -> w2147
          frame Disabled {
            n800 = call "Clear CAN Buffer.vi"("error in (no error)"=w2184, "Cluster in"=w2182) -> ("error out"=w2183:errorcluster)  [unwired: 8 in, 1 out]
            n801 = call "Close CAN Device.vi"("error in (no error)"=w2183, "Cluster in"=w2182) -> ("error out"=w2181:errorcluster)  [unwired: 8 in, 1 out]
          }
          frame Enabled {
          }
        }
        n802 = property on="VISA Current" class="VISAName"() -> ("Value"=w2115:refnum<visa-resource-name>)  [unwired: 2 in, 2 out]
        n803 = local read "DAQmx Device Name"() -> (w2119:tag)
        n804 = VISA Close(VISA resource name=w2167, error in (no error)=w2159) -> (error out=w2161:errorcluster)
        n805 = VISA Close(VISA resource name=w2115) -> (error out=w2114:errorcluster)  [unwired: 1 in]
        n806 = property on="Stop Button" class="Bool (strict)"() -> ("Value"=w2139:bool)  [unwired: 2 in, 2 out]
        n807 = call "Operation (SubVI).vi"("On/Off"=FALSE, "Operation"=T5."Init", "DAQmx Device Name"=w2119) -> ("error out"=w2116:errorcluster)  [unwired: 8 in]
        n808 = property on="ClosePanel" class="Bool (strict)"() -> ("Value"=w2140:bool)  [unwired: 2 in, 2 out]
        n809 = Or(x=w2140, y=w2139) -> (x .or. y?=w2138:bool)
        n810 = Flush Queue(queue=w2162, error in (no error)=w2161) -> (queue out=w2164:refnum<queue>, error out=w2163:errorcluster)  [unwired: 1 out]
        n811 = Flush Queue(queue=w2169, error in (no error)=w2161) -> (queue out=w2168:refnum<queue>, error out=w2170:errorcluster)  [unwired: 1 out]
        n812 = case shown="False" w2138 {
          tunnel: w2170 -> [w2172 w2180]
          tunnel: w2168 -> [w2174 w2176]
          tunnel: w2164 -> [w2173 w2175]
          tunnel: w2163 -> [w2171 w2179]
          tunnel: [w2172 w2178] -> w2154
          tunnel: [w2171 w2177] -> w2153
          tunnel: [w2174 w2176] -> w2137
          tunnel: [w2173 w2175] -> w2136
          frame False {
          }
          frame True {
            n813 = Release Queue(queue=w2175, error in (no error)=w2179) -> (error out=w2177:errorcluster)  [unwired: 1 in, 2 out]
            n814 = Release Queue(queue=w2176, error in (no error)=w2180) -> (error out=w2178:errorcluster)  [unwired: 1 in, 2 out]
          }
        }
        n815 = Merge Errors(w2154, w2153, w2147, w2116, w2114) -> (w2152:errorcluster)
        n816 = property on="Refresh Button" class="Bool (strict)"() -> ("Value"=w2141:bool)  [unwired: 2 in, 2 out]
        n817 = call <vilib>:"Clear Errors.vi"("error in (no error)"=w2152) -> ("error out"=w2151:errorcluster)  [unwired: 5 in, 1 out]
        n818 = property on="Stop Button" class="Bool (strict)"() -> ("Value"=w2145:bool)  [unwired: 2 in, 2 out]
        n819 = property on="ClosePanel" class="Bool (strict)"(error in=w2151) -> (error out=w2149:errorcluster, "Value"=w2150:bool)  [unwired: 1 in, 1 out]
        n820 = Not(x=w2141) -> (.not. x?=w2142:bool)
        n821 = Select(t=T3."Initialize", s=w2141, f=T3."Stop") -> (s? t:f=w2155:T3)
        n822 = Not(x=w2145) -> (.not. x?=w2144:bool)
        n823 = Compound Arithmetic op=AND(w2150, w2144, w2142) -> (w2146:bool)
        n824 = case shown="False" w2146 {
          tunnel: w2149 -> [w2188 w2192]
          tunnel: [w2188 w2192] -> w2148
          tunnel: [w2187 w2191] -> w2143
          tunnel: w2141 -> [w2186 _]
          frame False {
            n825 = case shown="False" w2186 {
              tunnel: [TRUE FALSE] -> w2187
              frame False {
              }
              frame True {
              }
            }
          }
          frame True {
            n826 = flat-sequence {
              tunnel: [TRUE] -> w2191
              frame #0 {
              }
              frame #1 {
                n827 = control-ref of="This VI"() -> (w2195:refnum<vi>)
                n828 = property class="VI"(reference=w2195, "FP.State"=T15."Closed" ("Front Panel Window:State")) -> ()  [unwired: 1 in, 2 out]
              }
            }
          }
        }
      }
      frame "MainProgram" {
        n829 = event shown="[0] Timeout" {
          selector: w2210 -> [_ _ _ _ _ _ _ _ _ _ _ _ _]
          dyn-events: _ -> [_ _ _ _ _ _ _ _ _ _ _ _ _]
          timeout: "EventTimeout" -> [_ _ _ _ _ _ _ _ _ _ _ _ _]
          tunnel: [T3."MainProgram" T3."MainProgram" T3."MainProgram" T3."MainProgram" T3."MainProgram" T3."Stop" T3."MainProgram" w2572 T3."MainProgram" T3."MainProgram" T3."MainProgram" T3."Stop" T3."MainProgram"] -> w2223
          tunnel: [w2232 w2345 w2413 w2422 w2433 w2453 w2468 w2618 w2681 w2696 _ w2718 w2719] -> w2217
          tunnel: w2221 -> [w2238 w2345 w2412 w2424 w2433 w2453 _ w2618 w2682 w2695 w2703 w2718 w2719]
          tunnel: [w2229 w2339 w2414 w2423 w2434 w2451 w2460 w2577 w2679 w2693 _ w2716 w2723] -> w2218
          tunnel: w2219 -> [w2229 w2339 w2414 w2423 w2434 w2451 w2460 w2577 w2679 w2693 _ w2716 w2723]
          tunnel: w2216 -> [w2240 w2351 w2408 w2419 w2430 w2450 w2471 w2602 w2678 w2692 w2707 w2715 w2726]
          tunnel: w2215 -> [w2236 w2350 w2409 w2420 w2431 w2449 w2464 w2601 w2677 w2691 w2706 w2714 w2722]
          tunnel: [w2237 w2350 w2409 w2420 w2431 w2449 w2464 w2601 w2677 w2691 w2706 w2714 w2722] -> w2214
          tunnel: [w2239 w2351 w2408 w2419 w2430 w2450 w2471 w2602 w2678 w2692 w2707 w2715 w2726] -> w2213
          tunnel: w2212 -> [w2234 w2349 w2407 w2418 w2429 w2448 w2470 w2600 w2676 w2690 w2705 w2713 w2725]
          tunnel: [w2234 w2349 w2407 w2418 w2429 w2448 w2467 w2600 w2676 w2690 w2705 w2713 w2725] -> w2211
          tunnel: w2209 -> [_ _ _ _ _ _ _ w2555 _ _ _ _ _]
          tunnel: w2208 -> [w2235 w2348 w2406 w2417 w2428 w2446 w2465 w2581 w2675 w2689 w2704 w2712 w2724]
          tunnel: [w2235 w2348 w2406 w2417 w2428 w2446 w2465 w2580 w2675 w2689 w2704 w2712 w2724] -> w2207
          tunnel: w2206 -> [_ w2346 _ _ _ _ _ w2579 _ _ _ _ _]
          tunnel: w2205 -> [_ w2338 _ _ _ _ _ _ _ _ _ _ _]
          tunnel: w2204 -> [_ _ _ _ _ _ _ _ w2674 _ _ _ _]
          tunnel: w2203 -> [_ w2327 w2405 w2416 w2427 w2443 w2463 w2556 w2672 w2688 w2701 w2711 w2721]
          tunnel: [_ w2327 w2405 w2416 w2427 w2443 w2463 w2556 w2672 w2688 w2701 w2711 w2721] -> w2202
          tunnel: w2201 -> [w2231 w2326 w2404 w2415 w2426 w2442 w2462 w2548 w2671 w2687 w2700 w2710 w2720]
          tunnel: [w2230 w2326 w2404 w2415 w2426 w2442 w2462 w2548 w2671 w2687 w2700 w2710 w2720] -> w2200
          event Timeout {
            n830 = event-data() -> ()  [unwired: 1 in, 3 out]
            n831 = disable-structure shown="Enabled" {
              disable-tunnel: w2240 -> [w2257 w2317]
              disable-tunnel: [w2256 w2317] -> w2239
              disable-tunnel: w2238 -> [w2255 w2316]
              disable-tunnel: [w2254 w2314] -> w2237
              disable-tunnel: w2236 -> [w2253 w2314]
              disable-tunnel: [w2250 w2316] -> w2232
              disable-tunnel: w2231 -> [w2248 w2315]
              disable-tunnel: [w2247 w2315] -> w2230
              frame Disabled {
                n832 = property class="Clust (strict)"(reference=w2253, error in=w2255) -> (reference out=w2254:refnum<vi>, error out=w2249:errorcluster, "Value"=w2260:T24)
                n833 = Unbundle By Name(w2260) -> ("DevType"=w2261:T18, "CanIndex"=w2259:T19)
                n834 = call "VCI_Receive.vi"("CANIndex"=w2259, "DevIndex"=u32 0, "DevType"=w2261) -> ("Recieve"=w2258:T25[])  [unwired: 3 in, 5 out]
                n835 = Empty Array?(array=w2258) -> (empty?=w2252:bool)
                n836 = case shown="False" w2252 {
                  tunnel: w2259 -> [w2275 _]
                  tunnel: w2254 -> [w2273 _]
                  tunnel: w2257 -> [w2272 w2305]
                  tunnel: w2249 -> [w2271 w2304]
                  tunnel: w2258 -> [w2276 _]
                  tunnel: [w2266 w2304] -> w2250
                  tunnel: [w2265 w2305] -> w2256
                  tunnel: [TRUE w2299] -> w2251
                  tunnel: w2248 -> [_ w2303]
                  tunnel: [0 w2302] -> w2247
                  frame False {
                    n837 = call "Demo_MakeDispBuff.vi"("Channel"=w2275, "Type"=enum16{"接收", "发送"}."接收", "OBJs"=w2276) -> ("Buffer"=w2274:T26)
                    n838 = for {
                      N: 3 -> [_]
                      tunnel: w2274 -> [w2290]
                      tunnel: w2273 -> [w2289]
                      tunnel: w2272 -> [w2280]
                      tunnel: w2271 -> [w2279]
                      tunnel: [w2282] -> w2269 mode=indexing
                      tunnel: [w2280] -> w2268
                      tunnel: [w2279] -> w2267
                      i -> [w2278]
                      n839 = property class="Clust (strict)"(reference=w2289) -> ("Value"=w2287:T24)  [unwired: 1 in, 2 out]
                      n840 = Index Array(array=w2290, index=w2278) -> (element=w2283:T27)
                      n841 = Unbundle By Name(w2283) -> ("Channel"=w2285:T19, "VCI_CAN_OBJ"=w2288:T25)  [unwired: 2 out]
                      n842 = Unbundle By Name(w2287) -> ("CanIndex"=w2286:T19)
                      n843 = Equal?(x=w2286, y=w2285) -> (x = y?=w2284:bool)
                      n844 = case shown="True" w2284 {
                        tunnel: w2288 -> [_ w2298]
                        tunnel: [w2291 w2294] -> w2282
                        tunnel: T16 {"ID"=0, "MSGTYPE"=0, "LEN"=0, "aDATA"=[]} ("Msg") -> [w2291 w2293]
                        frame False {
                        }
                        frame True {
                          n845 = Unbundle By Name(w2298) -> ("ID"=w2292:u32, "DataLen"=w2297:u8, "Data"=w2295:u8[])
                          n846 = Bundle By Name(cluster=w2293, "ID"=w2292, "MSGTYPE"=u8 0, "LEN"=w2297, "aDATA"=w2295) -> (w2294:T16)
                        }
                      }
                    }
                    n847 = Enqueue Element(queue=w2268, element=w2269, error in (no error)=w2267) -> (queue out=w2265:refnum<queue>, error out=w2266:errorcluster)  [unwired: 2 out]
                  }
                  frame True {
                    n848 = Increment(x=w2303) -> (x+1=w2302:i32)
                    n849 = Greater Or Equal?(x=w2302, y=7) -> (x >= y?=w2300:bool)
                    n850 = Not(x=w2300) -> (.not. x?=w2299:bool)
                  }
                }
                n851 = property on="CAN Status" class="Bool (strict)"("Value"=w2251) -> ()  [unwired: 2 in, 2 out]
              }
              frame Enabled {
                n852 = property on="VISA Current" class="VISAName"() -> ("Value"=w2308:refnum<visa-resource-name>)  [unwired: 2 in, 2 out]
                n853 = Not Equal?(x=w2308, y=refnum<visa-resource-name> "COMx") -> (x != y?=w2309:bool)
                n854 = case shown="True" w2309 {
                  tunnel: w2308 -> [_ w2320]
                  frame False {
                  }
                  frame True {
                    n855 = call "ReadCurrent.vi"("LoopFromMain"=TRUE, "VISA resource name"=w2320) -> ("CurrentOut"=→"CurrentOut":string)  [unwired: 8 in, 1 out]
                  }
                }
                n856 = control-ref of="ATR"() -> (w2306:refnum<vi>)
                n857 = call "PassFailUUT (SubVI).vi"("Table in"=w2306) -> ("PassFaileUUTresult"=w2307:bool)  [unwired: 8 in, 2 out]
                n858 = property on="Test Failed" class="Bool (strict)"("Value"=w2307) -> ()  [unwired: 2 in, 2 out]
                n859 = property on="Automation" class="Bool (strict)"() -> ("Value"=w2313:bool)  [unwired: 2 in, 2 out]
                n860 = property on="Start" class="Bool (strict)"() -> ("Value"=w2311:bool)  [unwired: 2 in, 2 out]
                n861 = Or(x=w2313, y=w2311) -> (x .or. y?=w2312:bool)
                n862 = case shown="False" w2312 {
                  frame False {
                    n863 = property on="Pannel User Message" class="Str"("Value"="You can press start to execute(s) test(s).") -> ()  [unwired: 2 in, 2 out]
                  }
                  frame True {
                  }
                }
              }
            }
            n864 = property on="ClosePanel" class="Bool (strict)"("Value"=FALSE ("ClosePanel")) -> ()  [unwired: 2 in, 2 out]
            n865 = Not Equal?(x=w2229, y=refnum<visa-resource-name> "COMx") -> (x != y?=w2227:bool)
            n866 = property on="Analogtest" class="Bool (strict)"() -> ("Value"=w2225:bool)  [unwired: 2 in, 2 out]
            n867 = Not(x=w2225) -> (.not. x?=w2224:bool)
            n868 = And(x=w2224, y=w2227) -> (x .and. y?=w2226:bool)
            n869 = case shown="True" w2226 {
              tunnel: w2229 -> [_ w2246]
              frame False {
              }
              frame True {
                n870 = call "Serial.vi"("Clear Log"=FALSE, "write buffer"="VC\r\n", "VISA resource name"=w2246) -> ("read buffer"=w2242:string)  [unwired: 7 in, 1 out]
                n871 = Fract/Exp String To Number(string=w2242) -> (number=→"Motor Speed RPM Serial":dbl)  [unwired: 3 in, 1 out]
              }
            }
          }
          event "SetSN": Value Change {
            n872 = event-data() -> ()  [unwired: 1 in, 6 out]
            n873 = property on="UUT" class="Str"() -> ("Value"=w2325:string)  [unwired: 2 in, 2 out]
            n874 = case shown="\"BLDC 30A\", Default" w2325 {
              tunnel: [26 26 26 26 35] -> w2323
              frame "BLDC 30A", Default {
              }
              frame "Warrior 60A" {
              }
              frame "Condenser Merkava" {
              }
              frame "Condenser India" {
              }
              frame "BLDC 60A" {
              }
            }
            n875 = control-ref of="ATR"() -> (w2330:refnum<vi>)
            n876 = property on="Current SN" class="DigNum (strict)"(error in=w2345) -> (error out=w2329:errorcluster, "Value"=w2344:i32)  [unwired: 1 in, 1 out]
            n877 = call "PassFailUUT (SubVI).vi"("error in (no error)"=w2329, "Table in"=w2330) -> ("Total Pass"=w2324:u8)  [unwired: 7 in, 2 out]
            n878 = Equal To 0?(x=w2344) -> (x = 0?=w2341:bool)
            n879 = Equal?(x=w2344, y=-1) -> (x = y?=w2342:bool)
            n880 = Equal?(x=w2324, y=w2323) -> (x = y?=w2322:bool)
            n881 = Or(x=w2342, y=w2341) -> (x .or. y?=w2340:bool)
            n882 = property on="CAN Status" class="Bool (strict)"() -> ("Value"=w2331:bool)  [unwired: 2 in, 2 out]
            n883 = property on="Serial Status" class="Bool (strict)"() -> ("Value"=w2336:bool)  [unwired: 2 in, 2 out]
            n884 = And(x=w2336, y=w2331) -> (x .and. y?=w2332:bool)
            n885 = case shown="True" w2332 {
              tunnel: w2346 -> [_ w2370]
              tunnel: w2340 -> [_ w2359]
              tunnel: w2339 -> [_ w2369]
              tunnel: w2338 -> [_ w2368]
              tunnel: [errorcluster {"status"=FALSE, "code"=0, "source"=""} ("error out") w2367] -> w2335
              tunnel: [w2357 w2366] -> w2337
              tunnel: w2322 -> [_ w2360]
              frame False {
                w2357 = FALSE ("Value")
                n886 = property on="SetSN" class="Bool (strict)"("Value"=w2357) -> ()  [unwired: 2 in, 2 out]
                n887 = call "Display Message to User10"() -> ()  [unwired: 10 in, 2 out]
              }
              frame True {
                n888 = property on="Test Failed" class="Bool (strict)"() -> ("Value"=w2364:bool)  [unwired: 2 in, 2 out]
                n889 = property on="Automation" class="Bool (strict)"() -> ("Value"=w2366:bool)  [unwired: 2 in, 2 out]
                n890 = Not(x=w2364) -> (.not. x?=w2365:bool)
                n891 = Select(t=w2365, s=w2366, f=w2368) -> (s? t:f=w2362:bool)
                n892 = Or(x=w2360, y=w2362) -> (x .or. y?=w2361:bool)
                n893 = And(x=w2359, y=w2361) -> (x .and. y?=w2363:bool)
                n894 = case shown="True" w2363 {
                  tunnel: w2370 -> [_ w2401]
                  tunnel: w2369 -> [_ w2394]
                  tunnel: [w2372 w2386] -> w2367
                  tunnel: w2359 -> [w2371 _]
                  frame False {
                    n895 = case shown="True" w2371 {
                      tunnel: [w2374 w2375] -> w2372
                      frame False {
                        n896 = call "Display Message to User9"() -> ("error out"=w2374:errorcluster)  [unwired: 10 in, 1 out]
                      }
                      frame True {
                        n897 = call "Display Message to User3"() -> ("error out"=w2375:errorcluster)  [unwired: 10 in, 1 out]
                      }
                    }
                    n898 = property on="Automation" class="Bool (strict)"(error in=w2372, "Value"=FALSE ("Automation")) -> ()  [unwired: 1 in, 2 out]
                  }
                  frame True {
                    w2393 = FALSE ("SetSN")
                    n899 = local read "DAQmx Device Name"() -> (w2379:tag)
                    n900 = property on="Next SN" class="DigNum (strict)"() -> ("Value"=w2381:i32)  [unwired: 2 in, 2 out]
                    n901 = call "Operation (SubVI).vi"("On/Off"=FALSE, "Operation"=T5."Venable", "DAQmx Device Name"=w2379) -> ("error out"=w2383:errorcluster)  [unwired: 8 in]
                    n902 = call <vilib>:"Clear Errors.vi"("error in (no error)"=w2383) -> ("error out"=w2384:errorcluster)  [unwired: 5 in, 1 out]
                    n903 = Number To Decimal String(number=w2381) -> (decimal integer string=w2382:string)  [unwired: 1 in]
                    "UUT SN Report" <- w2382
                    n904 = Search and Replace String(input string="EP=1\r\nSN=0\r\n" ("write buffer"), search string="0", replace string=w2382) -> (result string=w2396:string)  [unwired: 5 in, 3 out]
                    n905 = call "Serial.vi"("error in (no error)"=w2384, "Clear Log"=FALSE, "write buffer"=w2396, "VISA resource name"=w2394) -> ("error out"=w2378:errorcluster)  [unwired: 6 in, 1 out]
                    n906 = property on="UUT" class="Str"(error in=w2378) -> ("Value"=w2377:string)  [unwired: 1 in, 2 out]
                    n907 = call <vilib>:"Open Config Data.vi"("create file if necessary (T)"=FALSE, "configuration file path"=w2401) -> ("error out"=w2399:errorcluster, "refnum"=w2400:T4)  [unwired: 1 in, 7 out]
                    n908 = call-poly <vilib>:"Write Key.vi"("section"=w2377, "error in (no error)"=w2399, "value"=w2382, "key"="SN", "refnum"=w2400) -> ("error out"=w2389:errorcluster, "refnum out"=w2388:T4)  [unwired: 4 in, 1 out]
                    n909 = call <vilib>:"Close Config Data.vi"("error in (no error)"=w2389, "refnum"=w2388) -> ("error out"=w2387:errorcluster)  [unwired: 8 in, 1 out]
                    n910 = property on="Current SN" class="DigNum (strict)"("Value"=w2381) -> ()  [unwired: 2 in, 2 out]
                    n911 = property on="SetSN" class="Bool (strict)"(error in=w2387, "Value"=w2393) -> (error out=w2392:errorcluster)  [unwired: 1 in, 1 out]
                    n912 = property on="Automation" class="Bool (strict)"(error in=w2392, "Value"=w2393) -> (error out=w2391:errorcluster)  [unwired: 1 in, 1 out]
                    n913 = Increment(x=w2381) -> (x+1=w2390:i32)
                    n914 = property on="Next SN" class="DigNum (strict)"(error in=w2391, "Value"=w2390) -> (error out=w2386:errorcluster)  [unwired: 1 in, 1 out]
                  }
                }
              }
            }
            n915 = call <vilib>:"Clear Errors.vi"("error in (no error)"=w2335) -> ("error out"=w2328:errorcluster)  [unwired: 5 in, 1 out]
            n916 = property on="SetSN" class="Bool (strict)"(error in=w2328, "Value"=FALSE ("SetSN")) -> (error out=w2334:errorcluster)  [unwired: 1 in, 1 out]
            n917 = case shown="True" w2337 {
              tunnel: w2334 -> [_ _]
              frame False {
              }
              frame True {
                w2403 = TRUE ("Value (Signaling)")
                n918 = property on="Report" class="Bool (strict)"("Val(Sgnl)"=w2403, "Value"=w2403) -> ()  [unwired: 2 in, 2 out]
              }
            }
          }
          event "ATR": Mouse Enter {
            n919 = event-data() -> ()  [unwired: 1 in, 4 out]
            n920 = call-poly <vilib>:"Set Cursor.vi"("error in (no error)"=w2412, "icon"=u16 1) -> ("error out"=w2413:errorcluster)  [unwired: 8 in, 1 out]
          }
          event "ATR": Mouse Leave {
            n921 = event-data() -> ()  [unwired: 1 in, 4 out]
            n922 = call-poly <vilib>:"Set Cursor.vi"("error in (no error)"=w2424, "icon"=u16 0) -> ("error out"=w2422:errorcluster)  [unwired: 8 in, 1 out]
          }
          event "ATR": Mouse Down? {
            n923 = event-data() -> ("Coords"=w2441:T28)  [unwired: 1 in, 4 out]
            n924 = invoke on="ATR" class="Tbl (strict)" method="Point To Row Column"("Point"=w2441) -> ("InBounds"=w2437:bool, "CellPosition"=w2436:T14)  [unwired: 5 in, 4 out]
            n925 = Greater Than 0?(x=w2436) -> (x > 0?=w2440:cluster{"Row":bool, "Column":bool})
            n926 = Cluster To Array(cluster=w2440) -> (array=w2439:bool[])
            n927 = Or Array Elements(Boolean array=w2439) -> (logical OR=w2438:bool)
            n928 = Or(x=w2437, y=w2438) -> (x .or. y?=w2435:bool)
            n929 = event-data("Discard?"=w2435) -> ()  [unwired: 1 in, 1 out]
          }
          event Panel Close? {
            n930 = event-data() -> ("VIRef"=w2447:refnum<vi>)  [unwired: 1 in, 3 out]
            n931 = Close Reference(reference=w2447) -> ()  [unwired: 1 in, 1 out]
            n932 = disable-structure shown="Disabled" {
              frame Disabled {
                n933 = property on="Stop Button" class="Bool (strict)"("Val(Sgnl)"=TRUE ("Stop Button"), "Value"=FALSE ("Stop Button")) -> ()  [unwired: 2 in, 2 out]
              }
              frame Enabled {
              }
            }
            n934 = event-data("Discard?"=TRUE) -> ()  [unwired: 1 in, 1 out]
            "ClosePanel" <- TRUE ("ClosePanel")
          }
          event "Start": Value Change {
            w2458 = string[] []  # TestArray
            n935 = event-data() -> ()  [unwired: 1 in, 2 out]
            n936 = while {
              tunnel: [w2482] -> w2457
              tunnel: [w2481] -> w2469
              shift-right: [w2479] -> _
              shift-left: enum16{"Stop", "Tests", "Bit test", "Start"}."Start" -> [w2480]
              tunnel: w2458 -> [w2478]
              stop <- w2477 stop-if-true
              n937 = case shown="\"Tests\"" w2480 {
                tunnel: [w2487 w2492 w2502 w2513] -> w2482
                tunnel: [errorcluster {"status"=FALSE, "code"=0, "source"=""} ("error out") w2491 errorcluster {"status"=FALSE, "code"=0, "source"=""} ("error out") w2511] -> w2481
                tunnel: [w2486 w2498 enum16{"Stop", "Tests", "Bit test", "Start"}."Stop" w2507] -> w2479
                tunnel: w2478 -> [w2487 _ w2502 w2513]
                tunnel: [w2485 w2497 FALSE FALSE] -> w2477
                frame "Stop", Default {
                  n938 = flat-sequence {
                    tunnel: [enum16{"Stop", "Tests", "Bit test", "Start"}."Stop"] -> w2486
                    tunnel: [TRUE] -> w2485
                    frame #0 {
                    }
                  }
                  n939 = property on="Start" class="Bool (strict)"("Value"=FALSE ("Start")) -> ()  [unwired: 2 in, 2 out]
                }
                frame "Tests" {
                  w2496 = T13."Disabled and Grayed Out" ("Disabled")
                  n940 = property on="TestArray" class="Arr (strict)"() -> (error out=w2491:errorcluster, "Value"=w2493:string[])  [unwired: 2 in, 1 out]
                  n941 = call "Start Test Selection (SubVI).vi"("TestArrayIn"=w2493) -> ("AutoOut"=w2490:bool, "TestArrayOut"=w2492:string[])  [unwired: 9 in]
                  "Automation" <- w2490
                  n942 = property on="Start" class="Bool (strict)"("DisabledEnum"=w2496) -> ()  [unwired: 2 in, 2 out]
                  n943 = property on="Report" class="Bool (strict)"("DisabledEnum"=w2496) -> ()  [unwired: 2 in, 2 out]
                  n944 = control-ref of="ATR"() -> (w2494:refnum<vi>)
                  n945 = property on="Stop Button" class="Bool (strict)"("Value"=FALSE ("Stop Burn-in")) -> ()  [unwired: 2 in, 2 out]
                  n946 = case shown="True" w2490 {
                    tunnel: w2494 -> [_ w2499]
                    frame False {
                    }
                    frame True {
                      n947 = call "ResetTable Result (SubVI).vi"("Table in"=w2499) -> ()  [unwired: 11 in]
                    }
                  }
                  n948 = flat-sequence {
                    tunnel: [enum16{"Stop", "Tests", "Bit test", "Start"}."Tests"] -> w2498
                    tunnel: [TRUE] -> w2497
                    frame #0 {
                    }
                  }
                }
                frame "Bit test" {
                }
                frame "Start" {
                  n949 = property on="CAN Status" class="Bool (strict)"() -> (error out=w2510:errorcluster, "Value"=w2509:bool)  [unwired: 2 in, 1 out]
                  n950 = property on="Serial Status" class="Bool (strict)"(error in=w2510) -> ("Value"=w2508:bool)  [unwired: 1 in, 2 out]
                  n951 = And(x=w2509, y=w2508) -> (x .and. y?=w2506:bool)
                  n952 = case shown="True" w2506 {
                    tunnel: [w2515 w2520] -> w2511
                    tunnel: [enum16{"Stop", "Tests", "Bit test", "Start"}."Stop" enum16{"Stop", "Tests", "Bit test", "Start"}."Tests"] -> w2507
                    frame False {
                      n953 = call "Display Message to User5"() -> ("error out"=w2515:errorcluster)  [unwired: 10 in, 1 out]
                    }
                    frame True {
                      n954 = control-ref of="Motor Speed RPM Serial"() -> (w2517:refnum<vi>)
                      n955 = control-ref of="Stop Button"() -> (w2518:refnum<vi>)
                      n956 = control-ref of="Pannel User Message"() -> (w2519:refnum<vi>)
                      n957 = call "Write panel message Kinetics (SubVI).vi"(4:"rpm"=w2517, 5:"rpm"=FALSE ("rpm"), "PrintTime"=FALSE, "Stop"=w2518, "Time to wait"=0.0, "Strin"="TESTER BIT TEST OPERATION IN PROCESS\nPlease wait...", "String in"=w2519) -> ("error out"=w2520:errorcluster)  [unwired: 3 in, 1 out]
                    }
                  }
                }
              }
            }
            n958 = Array Size(array=w2457) -> (size(s)=w2456:i32)
            n959 = case shown="1, Default" w2456 {
              frame 0 {
              }
              frame 1, Default {
                n960 = local read "DAQmx Device Name"() -> (w2476:tag)
                n961 = call "Operation (SubVI).vi"("On/Off"=TRUE, "Operation"=T5."PowerSuply", "DAQmx Device Name"=w2476) -> ("error out"=w2473:errorcluster)  [unwired: 8 in]
                n962 = call "Time Delay"("error in (no error)"=w2473) -> ()  [unwired: 10 in, 1 out]
              }
            }
            n963 = Bundle By Name(cluster=T1 {"VISA"="COM1", "TestArray"=[]}, "VISA"=w2460, "TestArray"=w2457) -> (w2461:T1)
            n964 = Enqueue Element(queue=w2470, element=w2461, error in (no error)=w2469) -> (queue out=w2467:refnum<queue>, error out=w2468:errorcluster)  [unwired: 2 out]
          }
          event "Report", "Stop Button": Value Change {
            w2558 = T29 1 items=["User Home"=0, "User Desktop"=1, "User Documents"=2, "User Application Data"=3, "User Preferences"=4, "User Temporary"=5, "Public Documents"=6, "Public Application Data"=7, "Public Preferences"=8, "Public Cache"=13, "System Core Libraries"=9, "System Installed Libraries"=10, "Application Files"=11, "Boot Volume Root"=12] ("system directory type")
            w2525 = FALSE ("Report")
            n965 = event-data() -> ("CtlRef"=w2576:refnum<vi>)  [unwired: 1 in]
            n966 = call <vilib>:"Get System Directory.vi"("create directory if not found? (F)"=TRUE, "system directory type"=w2558) -> ("system directory"=w2557:path)  [unwired: 9 in]
            n967 = Build Path(base path=w2557, name or relative path="KineticsReports") -> (appended path=w2611:path)
            n968 = property on="CAN Status" class="Bool (strict)"() -> ("Value"=w2561:bool)  [unwired: 2 in, 2 out]
            n969 = property on="Serial Status" class="Bool (strict)"() -> ("Value"=w2562:bool)  [unwired: 2 in, 2 out]
            n970 = call <vilib>:"Check if File or Folder Exists.vi"("path"=w2611) -> ("error out"=w2609:errorcluster, "file or folder exists?"=w2612:bool, "dup path"=w2610:path)  [unwired: 8 in]
            n971 = And(x=w2562, y=w2561) -> (x .and. y?=w2563:bool)
            n972 = case shown="False" w2612 {
              tunnel: w2609 -> [w2668 w2669]
              tunnel: w2610 -> [w2667 w2670]
              tunnel: [w2666 w2670] -> w2560
              tunnel: [w2665 w2669] -> w2614
              frame False {
                n973 = Create Folder(path (use dialog)=w2667, error in=w2668) -> (created path=w2666:path, error out=w2665:errorcluster)  [unwired: 1 in, 1 out]
              }
              frame True {
              }
            }
            n974 = case shown="True" w2563 {
              tunnel: [w2619 "" ("read buffer")] -> w2598
              tunnel: [w2619 w2621] -> w2551
              tunnel: w2577 -> [_ w2629]
              tunnel: [w2619 w2638] -> w2554
              tunnel: [w2619 w2622] -> w2552
              tunnel: [w2619 "" ("read buffer")] -> w2570
              frame False {
                w2619 = "N_A" ("read buffer")
              }
              frame True {
                n975 = call "Serial.vi"("write buffer"="SN\r\n", "VISA resource name"=w2629) -> ("error out"=w2634:errorcluster, "read buffer"=w2636:string)  [unwired: 8 in]
                n976 = Decimal String To Number(string=w2636) -> (number=w2635:i32)  [unwired: 2 in, 1 out]
                n977 = Number To Decimal String(number=w2635, width (-)=i16 4) -> (decimal integer string=w2638:string)
                n978 = call "Serial.vi"("error in (no error)"=w2634, "write buffer"="VR\r\n", "VISA resource name"=w2629) -> ("error out"=w2630:errorcluster, "read buffer"=w2622:string)  [unwired: 7 in]
                n979 = call "Serial.vi"("error in (no error)"=w2630, "write buffer"="PN\r\n", "VISA resource name"=w2629) -> ("read buffer"=w2620:string)  [unwired: 7 in, 1 out]
                n980 = String Length(string=w2620) -> (length=w2627:i32)
                n981 = Subtract(x=6, y=w2627) -> (x-y=w2626:i32)
                n982 = for {
                  N: w2626 -> [_]
                  shift-right: [w2643] -> w2623
                  shift-left: "" -> [w2642]
                  n983 = Concatenate Strings(w2642, "0" ("string")) -> (w2643:string)
                }
                n984 = Concatenate Strings("RD" ("string"), w2623, w2620) -> (w2621:string)
              }
            }
            n985 = Get Date/Time String(want seconds? (F)=TRUE) -> (date string=w2613:string)  [unwired: 2 in, 1 out]
            n986 = call <vilib>:"Open Config Data.vi"("create file if necessary (T)"=FALSE, "configuration file path"=w2579) -> ("refnum"=w2589:T4)  [unwired: 1 in, 8 out]
            n987 = property on="Logger Path" class="Path"(error in=w2614, "Value"=w2560, "StartPath"=w2560) -> (error out=w2592:errorcluster)  [unwired: 1 in, 1 out]
            n988 = Search and Replace String(replace all?=TRUE ("replace all? (F)"), input string=w2613, search string="/") -> (result string=w2595:string)  [unwired: 5 in, 3 out]
            n989 = local read "UUT"() -> (w2532:string)
            n990 = call-poly <vilib>:"Read Key.vi"("section"=w2532, "key"="version", "refnum"=w2589) -> ("error out"=w2584:errorcluster, "value"=w2587:string, "refnum out"=w2586:T4)  [unwired: 5 in, 1 out]
            n991 = call-poly <vilib>:"Read Key.vi"("section"="Kinetics", "error in (no error)"=w2584, "key"="Tester Software Ver", "refnum"=w2586) -> ("error out"=w2582:errorcluster, "value"=w2553:string, "refnum out"=w2585:T4)  [unwired: 4 in, 1 out]
            n992 = property on="POWER Board S/N" class="Str"() -> ("Value"=w2530:string)  [unwired: 2 in, 2 out]
            n993 = Concatenate Strings("ATR" ("string"), w2598, w2554, "_", w2595, ".docx" ("string")) -> (w2593:string)
            n994 = call <vilib>:"Close Config Data.vi"("error in (no error)"=w2582, "refnum"=w2585) -> ()  [unwired: 8 in, 2 out]
            n995 = Build Path(base path=w2560, name or relative path=w2593) -> (appended path=w2594:path)
            n996 = property on="DSP Board S/N" class="Str"() -> ("Value"=w2529:string)  [unwired: 2 in, 2 out]
            n997 = Concatenate Strings("  Rev-" ("string"), w2587) -> (w2578:string)
            n998 = while {
              tunnel: w2593 -> [w2650]
              tunnel: w2560 -> [w2647]
              shift-right: [w2649] -> w2591
              shift-left: w2594 -> [w2648]
              shift-right: [w2645] -> w2580
              shift-left: w2581 -> [w2646]
              tunnel: w2592 -> [w2651]
              tunnel: [w2652] -> w2559
              stop <- w2644 continue-if-true
              n999 = call <vilib>:"Check if File or Folder Exists.vi"("error in (no error)"=w2651, "path"=w2648) -> ("error out"=w2652:errorcluster, "file or folder exists?"=w2644:bool)  [unwired: 7 in, 1 out]
              n1000 = case shown="True" w2644 {
                tunnel: w2650 -> [_ w2664]
                tunnel: w2646 -> [_ w2656]
                tunnel: [w2654 w2661] -> w2649
                tunnel: w2648 -> [w2654 _]
                tunnel: w2647 -> [_ w2662]
                tunnel: [1 w2655] -> w2645
                frame False {
                }
                frame True {
                  w2657 = ".docx" ("search string")
                  n1001 = Search and Replace String(input string=w2664, search string=w2657) -> (result string=w2663:string)  [unwired: 6 in, 3 out]
                  n1002 = Number To Decimal String(number=w2656) -> (decimal integer string=w2659:string)  [unwired: 1 in]
                  n1003 = call <vilib>:"Space Constant.vi"() -> ("String"=w2658:string)
                  n1004 = Concatenate Strings(w2663, w2658, w2659, w2657) -> (w2660:string)
                  n1005 = Build Path(base path=w2662, name or relative path=w2660) -> (appended path=w2661:path)
                  n1006 = Increment(x=w2656) -> (x+1=w2655:i32)
                }
              }
            }
            n1007 = property on="ParamVersion" class="Str"() -> ("Value"=w2528:string)  [unwired: 2 in, 2 out]
            n1008 = call "HeaderBis.vi"("UUTHeader"=w2532, "POWER SN"=w2530, "Revision Param"=w2528, "P/N UUT"=w2551, "DSP SN"=w2529, "Driver S/N"=w2554, "VR"=w2552, "Oper."=w2555, "Tester Software Ver"=w2553) -> ("table header"=w2550:string, "Array"=w2549:string[][])  [unwired: 4 in, 1 out]
            n1009 = Open/Create/Replace File(file path (use dialog)=w2591, error in=w2559, operation (0:open)=T17."create") -> (error out=w2604:errorcluster)  [unwired: 3 in, 2 out]
            n1010 = control-ref of="ATR"() -> (w2616:refnum<vi>)
            n1011 = property class="Tbl (strict)"(reference=w2616, error in=w2604) -> ("Value"=w2617:string[][])  [unwired: 2 out]
            n1012 = control-ref of="ATR"() -> (w2542:refnum<vi>)
            n1013 = call "PassFailUUT (SubVI).vi"("Table in"=w2542) -> ("PassFaileUUTresult"=w2535:bool)  [unwired: 8 in, 2 out]
            n1014 = property on="Test Failed" class="Bool (strict)"("Value"=w2535) -> ()  [unwired: 2 in, 2 out]
            n1015 = call "MarvinReport.vi"("HEADER1"=w2550, "ATR Or"=w2616, "Steps   pfull"=w2617, "Footer UUT"=w2570, "pageNum"=3, "InputHeaderArray"=w2549, "FILE NAME"=w2593, "Report Folder"=w2591, "REV"=w2578, "Test-Conductor"=w2555) -> ("error out"=w2565:errorcluster)  [unwired: 4 in, 1 out]
            n1016 = Select(t="PASS" ("name or relative path"), s=w2535, f="FAIL" ("name or relative path")) -> (s? t:f=w2534:string)
            n1017 = call <vilib>:"Clear Errors.vi"("error in (no error)"=w2565) -> ("error out"=w2564:errorcluster)  [unwired: 5 in, 1 out]
            n1018 = property class="Bool (strict)"(reference=w2576, error in=w2564) -> ("BoolText.Text"=w2575:string)  [unwired: 2 out]
            n1019 = Equal?(x=w2575, y="Report") -> (x = y?=w2569:bool)
            n1020 = Select(t=T3."MainProgram", s=w2569, f=T3."MainProgram") -> (s? t:f=w2572:T3)
            n1021 = call <vilib>:"Application Directory.vi"() -> ("Application Directory"=w2538:path)
            n1022 = Build Path(base path=w2538, name or relative path="data\\TestResult.ini") -> (appended path=w2541:path)
            n1023 = Select(t="Save Report...", s=w2569, f="Program Stopped...\r\nPlease turn OFF All Power sinks") -> (s? t:f=w2567:string)
            n1024 = property on="Report" class="Bool (strict)"(error in=w2564, "Value"=w2525) -> (error out=w2526:errorcluster)  [unwired: 1 in, 1 out]
            n1025 = call <vilib>:"Open Config Data.vi"("configuration file path"=w2541) -> ("error out"=w2539:errorcluster, "refnum"=w2540:T4)  [unwired: 2 in, 7 out]
            n1026 = property on="Stop Button" class="Bool (strict)"(error in=w2526, "Value"=w2525) -> ()  [unwired: 1 in, 2 out]
            n1027 = property on="Pannel User Message" class="Str"("Value"=w2567) -> ()  [unwired: 2 in, 2 out]
            n1028 = call-poly <vilib>:"Write Key.vi"("section"="Kinetics", "error in (no error)"=w2539, "value"=w2534, "key"="Result", "refnum"=w2540) -> ("error out"=w2537:errorcluster, "refnum out"=w2536:T4)  [unwired: 4 in, 1 out]
            n1029 = call <vilib>:"Close Config Data.vi"("error in (no error)"=w2537, "refnum"=w2536) -> ()  [unwired: 8 in, 2 out]
          }
          event "Help Button": Value Change {
            n1030 = event-data() -> ()  [unwired: 1 in, 6 out]
            n1031 = vi-ref "Help.vi"() -> (w2684:refnum<vi>)
            n1032 = invoke class="VI" method="FP.Open"(reference=w2684, error in=w2682, "Activate"=TRUE ("Activate?"), "State"=T15."Standard") -> (error out=w2683:errorcluster)  [unwired: 1 in, 4 out]
            n1033 = call "Help.vi"("error in"=w2683, "TesterSWVersion"=w2674) -> ("error out"=w2681:errorcluster)  [unwired: 6 in]
            n1034 = property on="Help Button" class="Bool (strict)"("Value"=FALSE ("Help Button")) -> ()  [unwired: 2 in, 2 out]
          }
          event "Serial Com": Value Change {
            n1035 = event-data() -> ()  [unwired: 1 in, 6 out]
            n1036 = property on="Serial Com" class="Bool"(error in=w2695, "Visible"=FALSE) -> (error out=w2699:errorcluster)  [unwired: 1 in, 1 out]
            n1037 = property on="VISA Kinetics" class="VISAName"(error in=w2699, "Visible"=TRUE) -> (error out=w2696:errorcluster)  [unwired: 1 in, 1 out]
          }
          event "VISA Kinetics": Value Change {
            n1038 = event-data() -> ()  [unwired: 1 in, 6 out]
            n1039 = property on="Serial Com" class="Bool"(error in=w2703, "Visible"=FALSE) -> ()  [unwired: 1 in, 2 out]
            n1040 = property on="Pannel User Message" class="Str"(error in=w2703, "Value"="Serial connection in process" ("Pannel User Message")) -> ()  [unwired: 1 in, 2 out]
          }
          event "Refresh Button": Value Change {
            n1041 = event-data() -> ()  [unwired: 1 in, 6 out]
          }
          event "Settings": Value Change {
            n1042 = event-data() -> ()  [unwired: 1 in, 6 out]
          }
        }
      }
      frame "Initialize" {
        w2743 = 0
        w2745 = FALSE ("Visible")
        w2747 = FALSE ("Visible")
        w2729 = refnum<visa-resource-name> "COMx" ("VISA resource name")
        w2734 = FALSE ("Serial Status")
        n1043 = property on="EventTimeout" class="DigNum (strict)"(error in=errorcluster {"status"=FALSE, "code"=0, "source"=""} ("error out"), "Value"=100 ("EventTimeout")) -> (error out=w2737:errorcluster)  [unwired: 1 in, 1 out]
        n1044 = property on="ComTestResult" class="Bool (strict)"("Value"=w2747) -> ()  [unwired: 2 in, 2 out]
        n1045 = property on="VenableResult" class="Bool (strict)"("Value"=w2747) -> ()  [unwired: 2 in, 2 out]
        n1046 = property on="VenableDirectionResult" class="Bool (strict)"("Value"=w2747) -> ()  [unwired: 2 in, 2 out]
        n1047 = property on="Serial Com" class="Bool"(error in=w2737, "Visible"=FALSE) -> (error out=w2753:errorcluster)  [unwired: 1 in, 1 out]
        n1048 = property on="VisualInspectionResult" class="Bool (strict)"("Value"=FALSE ("Visible")) -> ()  [unwired: 2 in, 2 out]
        n1049 = property on="VISA Kinetics" class="VISAName"(error in=w2753, "Visible"=FALSE, "Value"=w2729) -> (error out=w2739:errorcluster)  [unwired: 1 in, 1 out]
        n1050 = property on="Analogtest" class="Bool (strict)"("Value"=w2734) -> ()  [unwired: 2 in, 2 out]
        n1051 = property on="Serial Status" class="Bool (strict)"("Value"=w2734) -> ()  [unwired: 2 in, 2 out]
        n1052 = property on="Refresh Button" class="Bool (strict)"(error in=w2739, "Value"=FALSE ("Refresh Button")) -> (error out=w2740:errorcluster)  [unwired: 1 in, 1 out]
        n1053 = property on="MotorTempResult" class="Bool (strict)"("Value"=w2745) -> ()  [unwired: 2 in, 2 out]
        n1054 = property on="Automation" class="Bool (strict)"("Value"=w2745) -> ()  [unwired: 2 in, 2 out]
        n1055 = call "Find DAQ Devices.vi"("Error In"=w2740) -> ("Error Out"=w2742:errorcluster, "Stop?"=w2733:bool, "DAQmx Device Name"=w2738:tag)  [unwired: 8 in]
        n1056 = case shown="False" w2733 {
          selector: w2733 -> [_ w2773]
          tunnel: w2742 -> [w2765 w2775]
          tunnel: [w2757 w2775] -> w2731
          tunnel: w2738 -> [w2756 _]
          tunnel: [T3."Erase ATR Table" T3."Stop"] -> w2732
          frame False {
            n1057 = call <vilib>:"Clear Errors.vi"("error in (no error)"=w2765) -> ("error out"=w2764:errorcluster)  [unwired: 5 in, 1 out]
            n1058 = Not Equal?(x=w2756, y=tag "") -> (x != y?=w2766:bool)
            n1059 = case shown="True" w2766 {
              tunnel: w2756 -> [_ w2772]
              tunnel: w2764 -> [w2768 w2771]
              tunnel: [w2768 w2770] -> w2763
              frame False {
              }
              frame True {
                n1060 = call "Operation (SubVI).vi"("error in (no error)"=w2771, "Operation"=T5."Init", "DAQmx Device Name"=w2772) -> ("error out"=w2770:errorcluster)  [unwired: 8 in]
              }
            }
            n1061 = call "Operation (SubVI).vi"("error in (no error)"=w2763, "On/Off"=TRUE, "Operation"=T5."0 ohm", "DAQmx Device Name"=w2756) -> ("error out"=w2758:errorcluster)  [unwired: 7 in]
            n1062 = call "Operation (SubVI).vi"("error in (no error)"=w2758, "On/Off"=TRUE, "Operation"=T5."PowerSuply", "DAQmx Device Name"=w2756) -> ("error out"=w2757:errorcluster)  [unwired: 7 in]
            "DAQmx Device Name" <- w2756
          }
          frame True {
            n1063 = Stop(stop? (T)=w2773) -> ()
          }
        }
        n1064 = call "COM Curent Read.vi"("error in (no error)"=w2731, "VISA resource name 2"=w2729) -> ("error out"=w2730:errorcluster, "VISA Current"=→"VISA Current":refnum<visa-resource-name>)  [unwired: 7 in, 1 out]
        "Test Failed" <- w2734
      }
    }
  }
  n1065 = call "ATRBuild.vi"() -> ()  [unwired: 9 in, 3 out]
  n1066 = disable-structure shown="Disabled" {
    frame Disabled {
      n1067 = case shown="\"BLDC 30A\", Default" {
        selector: _ -> [_ _ _ _ _]
        tunnel: [26 26 26 26 35] -> _
        frame "BLDC 30A", Default {
        }
        frame "Warrior 60A" {
        }
        frame "Condenser Merkava" {
        }
        frame "Condenser India" {
        }
        frame "BLDC 60A" {
        }
      }
    }
    frame Enabled {
    }
  }
  n1068 = disable-structure shown="Disabled" {
    frame Disabled {
      n1069 = control-ref of="Stop Button"() -> ()  [unwired: 1 out]
      n1070 = control-ref of="UUT"() -> ()  [unwired: 1 out]
      n1071 = property on="UUT" class="Str" props=["Value"]() -> ()  [unwired: 2 in, 3 out]
      n1072 = control-ref of="UUT"() -> ()  [unwired: 1 out]
      n1073 = property on="UUT" class="DigNum (strict)" props=["Value"]() -> ()  [unwired: 2 in, 3 out]
      n1074 = control-ref of="Motor Speed RPM Serial"() -> ()  [unwired: 1 out]
      n1075 = call "Find_Number_LineMARVIN.vi"() -> ()  [unwired: 5 in, 4 out]
      n1076 = control-ref of="Pannel User Message"() -> ()  [unwired: 1 out]
      n1077 = call "Write panel message Kinetics (SubVI).vi"() -> ()  [unwired: 10 in, 2 out]
      n1078 = local read "DAQmx Device Name"() -> (w2782:tag)
      n1079 = control-ref of="ATR"() -> ()  [unwired: 1 out]
      n1080 = call "PassOrFail (SubVI).vi"() -> ()  [unwired: 11 in, 1 out]
      n1081 = call "Serial.vi"("write buffer"="EP=1\r\nVC=1000\r\n") -> ()  [unwired: 9 in, 2 out]
      n1082 = call "Operation (SubVI).vi"("DAQmx Device Name"=w2782) -> ()  [unwired: 10 in, 1 out]
      n1083 = property on="UUT" class="Str" props=["Value"]() -> ()  [unwired: 2 in, 3 out]
    }
    frame Enabled {
    }
  }
  n1084 = disable-structure shown="Disabled" {
    frame Disabled {
      w2783 = T13."Disabled and Grayed Out" ("Disabled")
      w2784 = FALSE ("Start")
      n1085 = property on="Current SN" class="DigNum (strict)" props=["Value"]() -> ()  [unwired: 2 in, 3 out]
      n1086 = property on="UUT" class="DigNum (strict)" props=["Value"]() -> ()  [unwired: 2 in, 3 out]
      n1087 = property on="Serial Status" class="Bool (strict)" props=["Value"]() -> ()  [unwired: 2 in, 3 out]
      n1088 = property on="UUT SoftwareVer" class="Str" props=["Value"]() -> ()  [unwired: 2 in, 3 out]
      n1089 = call "Operation (SubVI).vi"() -> ()  [unwired: 11 in, 1 out]
      n1090 = property on="Next SN" class="DigNum (strict)" props=["Value"]() -> ()  [unwired: 3 in, 2 out]
      n1091 = property on="Start" class="Bool (strict)"("Value"=w2784, "DisabledEnum"=w2783) -> ()  [unwired: 2 in, 2 out]
      n1092 = property on="Report" class="Bool (strict)"("Value"=w2784, "DisabledEnum"=w2783) -> ()  [unwired: 2 in, 2 out]
    }
    frame Enabled {
    }
  }
  "Pannel User Message" <- w17
